vi "Beampointing_Multi_Pico2_upstairs01.vi"() -> ()   [LabVIEW 2011]
uses:
  GUI_Template/GUI_master/tcp_new_data_event.ctl
  GUI_Template/GUI_master/tcp new data cluster.ctl
  Ctrs/beam detection.ctl
  GUI_Beampointing_single_TRA/Ctrs/move.ctl
  <vilib>/Utility/file.llb/Read From Spreadsheet File (string).vi
  <userlib>/_OpenG.lib/array/array.llb/Filter 1D Array with Scalar (String)__ogtk.vi
  <vilib>/Utility/file.llb/Write To Spreadsheet File (string).vi
  <vilib>/Analysis/NI_AALBase.lvlib
panel:
  out "Moving Y":string
  out "Moving X":string
  out "particles":T1(array[cluster])
  out "millisecond timer value":u32
  out "appended path":path
  out "millisecond timer 2":u32
  in  "GUIdevice 98":string
  in  "Position.Axis 111::98":dbl=77.0 caption="Motor Axis 1" min=-999999.0 max=999999.0 format="%#_6f"
  in  "Position.Axis 112::98":dbl=77.0 caption="Motor Axis 1" min=-999999.0 max=999999.0 format="%#_6f"
  in  "Position.Axis 113::98":dbl=77.0 caption="Motor Axis 1" min=-999999.0 max=999999.0 format="%#_6f"
  in  "Position.Axis 121::98":dbl=77.0 caption="Motor Axis 1" min=-999999.0 max=999999.0 format="%#_6f"
  in  "Position.Axis 122::98":dbl=77.0 caption="Motor Axis 1" min=-999999.0 max=999999.0 format="%#_6f"
  in  "Position.Axis 123::98":dbl=77.0 caption="Motor Axis 1" min=-999999.0 max=999999.0 format="%#_6f"
  in  "Position.Axis 131::98":dbl=77.0 caption="Motor Axis 1" min=-999999.0 max=999999.0 format="%#_6f"
  in  "Position.Axis 132::98":dbl=77.0 caption="Motor Axis 1" min=-999999.0 max=999999.0 format="%#_6f"
  in  "Position.Axis 133::98":dbl=77.0 caption="Motor Axis 1" min=-999999.0 max=999999.0 format="%#_6f"
  in  "Position.Axis 141::98":dbl=77.0 caption="Motor Axis 1" min=-999999.0 max=999999.0 format="%#_6f"
  in  "Position.Axis 142::98":dbl=77.0 caption="Motor Axis 1" min=-999999.0 max=999999.0 format="%#_6f"
  in  "Position.Axis 143::98":dbl=77.0 caption="Motor Axis 1" min=-999999.0 max=999999.0 format="%#_6f"
  in  "Position.Axis 211::98":dbl=77.0 caption="Motor Axis 1" min=-999999.0 max=999999.0 format="%#_6f"
  in  "Position.Axis 212::98":dbl=77.0 caption="Motor Axis 1" min=-999999.0 max=999999.0 format="%#_6f"
  in  "Position.Axis 213::98":dbl=77.0 caption="Motor Axis 1" min=-999999.0 max=999999.0 format="%#_6f"
  in  "Position.Axis 221::98":dbl=77.0 caption="Motor Axis 1" min=-999999.0 max=999999.0 format="%#_6f"
  in  "Position.Axis 222::98":dbl=77.0 caption="Motor Axis 1" min=-999999.0 max=999999.0 format="%#_6f"
  in  "Position.Axis 223::98":dbl=77.0 caption="Motor Axis 1" min=-999999.0 max=999999.0 format="%#_6f"
  in  "Position.Axis 231::98":dbl=77.0 caption="Motor Axis 1" min=-999999.0 max=999999.0 format="%#_6f"
  in  "Position.Axis 232::98":dbl=77.0 caption="Motor Axis 1" min=-999999.0 max=999999.0 format="%#_6f"
  in  "Position.Axis 233::98":dbl=77.0 caption="Motor Axis 1" min=-999999.0 max=999999.0 format="%#_6f"
  in  "Position.Axis 241::98":dbl=77.0 caption="Motor Axis 1" min=-999999.0 max=999999.0 format="%#_6f"
  in  "Position.Axis 242::98":dbl=77.0 caption="Motor Axis 1" min=-999999.0 max=999999.0 format="%#_6f"
  in  "Position.Axis 243::98":dbl=77.0 caption="Motor Axis 1" min=-999999.0 max=999999.0 format="%#_6f"
  in  "Position.Axis 311::98":dbl=77.0 caption="Motor Axis 1" min=-999999.0 max=999999.0 format="%#_6f"
  in  "Position.Axis 312::98":dbl=77.0 caption="Motor Axis 1" min=-999999.0 max=999999.0 format="%#_6f"
  in  "Position.Axis 313::98":dbl=77.0 caption="Motor Axis 1" min=-999999.0 max=999999.0 format="%#_6f"
  in  "Position.Axis 321::98":dbl=77.0 caption="Motor Axis 1" min=-999999.0 max=999999.0 format="%#_6f"
  in  "Position.Axis 322::98":dbl=77.0 caption="Motor Axis 1" min=-999999.0 max=999999.0 format="%#_6f"
  in  "Position.Axis 323::98":dbl=77.0 caption="Motor Axis 1" min=-999999.0 max=999999.0 format="%#_6f"
  in  "Position.Axis 331::98":dbl=77.0 caption="Motor Axis 1" min=-999999.0 max=999999.0 format="%#_6f"
  in  "Position.Axis 332::98":dbl=77.0 caption="Motor Axis 1" min=-999999.0 max=999999.0 format="%#_6f"
  in  "Position.Axis 333::98":dbl=77.0 caption="Motor Axis 1" min=-999999.0 max=999999.0 format="%#_6f"
  in  "Position.Axis 341::98":dbl=77.0 caption="Motor Axis 1" min=-999999.0 max=999999.0 format="%#_6f"
  in  "Position.Axis 342::98":dbl=77.0 caption="Motor Axis 1" min=-999999.0 max=999999.0 format="%#_6f"
  in  "Position.Axis 343::98":dbl=77.0 caption="Motor Axis 1" min=-999999.0 max=999999.0 format="%#_6f"
  in  "Position.Axis 411::98":dbl=77.0 caption="Motor Axis 1" min=-999999.0 max=999999.0 format="%#_6f"
  in  "Position.Axis 412::98":dbl=77.0 caption="Motor Axis 1" min=-999999.0 max=999999.0 format="%#_6f"
  in  "Position.Axis 413::98":dbl=77.0 caption="Motor Axis 1" min=-999999.0 max=999999.0 format="%#_6f"
  in  "Position.Axis 421::98":dbl=77.0 caption="Motor Axis 1" min=-999999.0 max=999999.0 format="%#_6f"
  in  "Position.Axis 422::98":dbl=77.0 caption="Motor Axis 1" min=-999999.0 max=999999.0 format="%#_6f"
  in  "Position.Axis 423::98":dbl=77.0 caption="Motor Axis 1" min=-999999.0 max=999999.0 format="%#_6f"
  in  "Position.Axis 431::98":dbl=77.0 caption="Motor Axis 1" min=-999999.0 max=999999.0 format="%#_6f"
  in  "Position.Axis 432::98":dbl=77.0 caption="Motor Axis 1" min=-999999.0 max=999999.0 format="%#_6f"
  in  "Position.Axis 433::98":dbl=77.0 caption="Motor Axis 1" min=-999999.0 max=999999.0 format="%#_6f"
  in  "Position.Axis 441::98":dbl=77.0 caption="Motor Axis 1" min=-999999.0 max=999999.0 format="%#_6f"
  in  "Position.Axis 442::98":dbl=77.0 caption="Motor Axis 1" min=-999999.0 max=999999.0 format="%#_6f"
  in  "Position.Axis 443::98":dbl=77.0 caption="Motor Axis 1" min=-999999.0 max=999999.0 format="%#_6f"
  in  "Position.Axis 511::98":dbl=77.0 caption="Motor Axis 1" min=-999999.0 max=999999.0 format="%#_6f"
  in  "Position.Axis 512::98":dbl=77.0 caption="Motor Axis 1" min=-999999.0 max=999999.0 format="%#_6f"
  in  "Position.Axis 513::98":dbl=77.0 caption="Motor Axis 1" min=-999999.0 max=999999.0 format="%#_6f"
  in  "Position.Axis 521::98":dbl=77.0 caption="Motor Axis 1" min=-999999.0 max=999999.0 format="%#_6f"
  in  "Position.Axis 522::98":dbl=77.0 caption="Motor Axis 1" min=-999999.0 max=999999.0 format="%#_6f"
  in  "Position.Axis 523::98":dbl=77.0 caption="Motor Axis 1" min=-999999.0 max=999999.0 format="%#_6f"
  in  "Position.Axis 531::98":dbl=77.0 caption="Motor Axis 1" min=-999999.0 max=999999.0 format="%#_6f"
  in  "Position.Axis 532::98":dbl=77.0 caption="Motor Axis 1" min=-999999.0 max=999999.0 format="%#_6f"
  in  "Position.Axis 533::98":dbl=77.0 caption="Motor Axis 1" min=-999999.0 max=999999.0 format="%#_6f"
  in  "Position.Axis 541::98":dbl=77.0 caption="Motor Axis 1" min=-999999.0 max=999999.0 format="%#_6f"
  in  "Position.Axis 542::98":dbl=77.0 caption="Motor Axis 1" min=-999999.0 max=999999.0 format="%#_6f"
  in  "Position.Axis 543::98":dbl=77.0 caption="Motor Axis 1" min=-999999.0 max=999999.0 format="%#_6f"
  in  "Numeric":dbl
  out "Current State":string
  in  "output cluster 2":T5 {"detection para"."smal para"."Measurement Parameter" items=["Center of Mass X", "Center of Mass Y", "First Pixel X", "First Pixel Y", "Bounding Rect Left", "Bounding Rect Top", "Bounding Rect Right", "Bounding Rect Bottom", "Max Feret Diameter Start X", "Max Feret Diameter Start Y", "Max Feret Diameter End X", "Max Feret Diameter End Y", "Max Horiz. Segment Length Left", "Max Horiz. Segment Length Right", "Max Horiz. Segment Length Row", "-", "Bounding Rect Width", "Bounding Rect Height", "Bounding Rect Diagonal", "Perimeter", "Convex Hull Perimeter", "Holes' Perimeter", "Max Feret Diameter", "Equivalent Ellipse Major Axis", "Equivalent Ellipse Minor Axis", "Equivalent Ellipse Minor Axis (Feret)", "Equivalent Rect Long Side", "Equivalent Rect Short Side", "Equivalent Rect Diagonal", "Equivalent Rect Short Side (Feret)", "Average Horiz. Segment Length", "Average Vert. Segment Length", "Hydraulic Radius", "Waddel Disk Diameter", "-", "Area", "Holes' Area", "Particle & Holes' Area", "Convex Hull Area", "Image Area", "-", "Number of Holes", "Number of Horiz. Segments", "Number of Vert. Segments", "-", "Orientation", "Max Feret Diameter Orientation", "-", "% Area/Image Area", "% Area/(Particle & Holes' Area)", "Ratio of Equivalent Ellipse Axes", "Ratio of Equivalent Rect Sides", "-", "Elongation Factor", "Compactness Factor", "Heywood Circularity Factor", "Type Factor", "-", "Sum X", "Sum Y", "Sum XX", "Sum XY", "Sum YY", "Sum XXX", "Sum XXY", "Sum XYY", "Sum YYY", "-", "Moment of Inertia XX", "Moment of Inertia XY", "Moment of Inertia YY", "Moment of Inertia XXX", "Moment of Inertia XXY", "Moment of Inertia XYY", "Moment of Inertia YYY", "Norm. Moment of Inertia XX", "Norm. Moment of Inertia XY", "Norm. Moment of Inertia YY", "Norm. Moment of Inertia XXX", "Norm. Moment of Inertia XXY", "Norm. Moment of Inertia XYY", "Norm. Moment of Inertia YYY", "Hu Moment 1", "Hu Moment 2", "Hu Moment 3", "Hu Moment 4", "Hu Moment 5", "Hu Moment 6", "Hu Moment 7"]; "detection para"."smal para"."Range Lower Value" format="%.2f"; "detection para"."smal para"."Range Upper Value" format="%.2f"; "detection para"."detection method" items=["clustering", "entropy", "metric", "moments", "inter-class variance"]; "detection para"."Filter" items=["No Filter", "Median Filter", "Low Pass Filter"]}
  out "CCDs":string[](array[string])
  in  "GUIdevice 12":string
  in  "GUIdevice 11":string
  in  "GUIdevice 10":string
  in  "GUIdevice 9":string
  out "error out 2":errorcluster
  in  "active cams":string[](array[string])
  in  "Motor Y":dbl[][](array[numeric])
  in  "Motor X":dbl[][](array[numeric])
  out "Names":string[](array[string])
  in  "Offset X stats":dbl[][](array[numeric])
  in  "Offset Y stats":dbl[][](array[numeric])
  out "Box":T6(array[cluster])
  in  "Tab Control 2":enum32{"Config ", "Main", "History"}(tab)=enum."Main"
  out "Waveform Chart":u32(graph)
  in  "associated motors":T7 {"Motor CCD 12" items=["PA2_Input1", "PA2_Input2", "XPW_cam", "L1_TelInpNear", "A", "B", "a", "D", "", "TSa", "", "", "Focuscam", "Mirrorcam", "", "", "", "", "", ""]; "Motor CCD 11" items=["PA2_Input1", "PA2_Input2", "XPW_cam", "L1_TelInpNear", "A", "B", "a", "D", "", "TSa", "", "", "Focuscam", "Mirrorcam", "", "", "", "", "", ""]; "Motor CCD 10" items=["PA2_Input1", "PA2_Input2", "XPW_cam", "L1_TelInpNear", "A", "B", "a", "D", "", "TSa", "", "", "Focuscam", "Mirrorcam", "", "", "", "", "", ""]; "Motor CCD 9" items=["PA2_Input1", "PA2_Input2", "XPW_cam", "L1_TelInpNear", "A", "B", "a", "D", "", "TSa", "", "", "Focuscam", "Mirrorcam", "", "", "", "", "", ""]; "Motor CCD 8" items=["PA2_Input1", "PA2_Input2", "XPW_cam", "L1_TelInpNear", "A", "B", "a", "D", "", "TSa", "", "", "Focuscam", "Mirrorcam", "", "", "", "", "", ""]; "Motor CCD 7" items=["PA2_Input1", "PA2_Input2", "XPW_cam", "L1_TelInpNear", "A", "B", "a", "D", "", "TSa", "", "", "Focuscam", "Mirrorcam", "", "", "", "", "", ""]; "Motor CCD 6" items=["PA2_Input1", "PA2_Input2", "XPW_cam", "L1_TelInpNear", "A", "B", "a", "D", "", "TSa", "", "", "Focuscam", "Mirrorcam", "", "", "", "", "", ""]; "Motor CCD 5" items=["PA2_Input1", "PA2_Input2", "XPW_cam", "L1_TelInpNear", "A", "B", "a", "D", "", "TSa", "", "", "Focuscam", "Mirrorcam", "", "", "", "", "", ""]; "Motor CCD 4" items=["PA2_Input1", "PA2_Input2", "XPW_cam", "L1_TelInpNear", "A", "B", "a", "D", "", "TSa", "", "", "Focuscam", "Mirrorcam", "", "", "", "", "", ""]; "Motor CCD 3" items=["PA2_Input1", "PA2_Input2", "XPW_cam", "L1_TelInpNear", "A", "B", "a", "D", "", "TSa", "", "", "Focuscam", "Mirrorcam", "", "", "", "", "", ""]; "Motor CCD 2" items=["PA2_Input1", "PA2_Input2", "XPW_cam", "L1_TelInpNear", "A", "B", "a", "D", "", "TSa", "", "", "Focuscam", "Mirrorcam", "", "", "", "", "", ""]; "Motor CCD 1" items=["PA2_Input1", "PA2_Input2", "XPW_cam", "L1_TelInpNear", "A", "B", "a", "D", "", "TSa", "", "", "Focuscam", "Mirrorcam", "", "", "", "", "", ""]}
  out "Cameras":T8
  out "Status":cluster{i32, i32, "Centroid X":dbl[][]}(graph)
  in  "Exposure:12":dbl=0.095 min=0.0001 max=1.0 format="%#_6f"
  in  "Triggerdelay::12":dbl=0.003 min=0.0 max=0.09 format="%#_6f"
  in  "Exposure::11":dbl=0.095 min=0.0001 max=1.0 format="%#_6f"
  in  "Triggerdelay::11":dbl=0.003 min=0.0 max=0.09 format="%#_6f"
  in  "Exposure::10":dbl=0.095 min=0.0001 max=1.0 format="%#_6f"
  in  "Triggerdelay::10":dbl=0.003 min=0.0 max=0.09 format="%#_6f"
  in  "Exposure::9":dbl=0.095 min=0.0001 max=1.0 format="%#_6f"
  in  "Triggerdelay::9":dbl=0.003 min=0.0 max=0.09 format="%#_6f"
  in  "Trigger::9":bool
  in  "Trigger::10":bool caption="Trigger:10"
  in  "Trigger::11":bool
  in  "Trigger::12":bool
  in  "Target.Y::9":dbl=45.0 caption="T9y" min=0.0 max=2000.0 format="%#_6f"
  in  "Target.X::9":dbl=47.0 caption="Tx9" min=0.0 max=2000.0 format="%#_6f"
  in  "Target.Y::10":dbl=45.0 caption="T10y" min=0.0 max=2000.0 format="%#_6f"
  in  "Target.X::10":dbl=47.0 caption="T10x" min=0.0 max=2000.0 format="%#_6f"
  in  "Target.Y::11":dbl=45.0 caption="T11y" min=0.0 max=2000.0 format="%#_6f"
  in  "Target.X::11":dbl=47.0 caption="T11x" min=0.0 max=2000.0 format="%#_6f"
  in  "Target.Y::12":dbl=45.0 caption="T12y" min=0.0 max=2000.0 format="%#_6f"
  in  "Target.X::12":dbl=47.0 caption="T12x" min=0.0 max=2000.0 format="%#_6f"
  in  "Exposure::8":dbl=0.095 min=0.01 max=1.0 format="%#_6f"
  in  "Triggerdelay::8":dbl=0.003 min=0.0 max=0.09 format="%#_6f"
  in  "Trigger::8":bool
  in  "Target.Y::8":dbl=45.0 caption="T8y" min=0.0 max=2000.0 format="%#_6f"
  in  "Target.X::8":dbl=47.0 caption="T8x" min=0.0 max=2000.0 format="%#_6f"
  in  "Target.Y::7":dbl=45.0 caption="T7x" min=0.0 max=2000.0 format="%#_6f"
  in  "Target.X::7":dbl=47.0 caption="T7y" min=0.0 max=2000.0 format="%#_6f"
  in  "Target.Y::6":dbl=45.0 caption="T6y" min=0.0 max=2000.0 format="%#_6f"
  in  "Target.X::6":dbl=47.0 caption="T6x" min=0.0 max=2000.0 format="%#_6f"
  in  "Target.Y::5":dbl=45.0 caption="T5y" min=0.0 max=2000.0 format="%#_6f"
  in  "Target.X::5":dbl=47.0 caption="T5x" min=0.0 max=2000.0 format="%#_6f"
  in  "Target.Y::4":dbl=45.0 caption="T4y" min=0.0 max=2000.0 format="%#_6f"
  in  "Target.X::4":dbl=47.0 caption="T4x" min=0.0 max=2000.0 format="%#_6f"
  in  "Target.Y::3":dbl=163.0 caption="T3y" min=0.0 max=2000.0 format="%#_6f"
  in  "Target.X::3":dbl=152.0 caption="T3x" min=0.0 max=2000.0 format="%#_6f"
  in  "Target.Y::2":dbl=74.0 caption="T2y" min=0.0 max=2000.0 format="%#_6f"
  in  "Target.X::2":dbl=75.0 caption="T2x" min=0.0 max=2000.0 format="%#_6f"
  in  "Target.Y::1":dbl=61.0 caption="T1y" min=0.0 max=2000.0 format="%#_6f"
  in  "Target.X::1":dbl=77.0 caption="T1x" min=0.0 max=2000.0 format="%#_6f"
  in  "Exposure::7":dbl=0.095 min=0.0001 max=1.0 format="%#_6f"
  in  "Triggerdelay::7":dbl=0.003 min=0.0 max=0.09 format="%#_6f"
  in  "Trigger::7":bool
  in  "Exposure::6":dbl=0.095 min=0.0001 max=1.0 format="%#_6f"
  in  "Triggerdelay::6":dbl=0.003 min=0.0 max=0.09 format="%#_6f"
  in  "Trigger::6":bool
  in  "Exposure::5":dbl=0.095 min=0.0001 max=1.0 format="%#_6f"
  in  "Triggerdelay::5":dbl=0.003 min=0.0 max=0.09 format="%#_6f"
  in  "Trigger::5":bool
  in  "Exposure::4":dbl=0.095 min=0.0001 max=1.0 format="%#_6f"
  in  "Triggerdelay::4":dbl=0.003 min=0.0 max=0.09 format="%#_6f"
  in  "Trigger::4":bool
  in  "Exposure::3":dbl=0.095 min=0.0001 max=1.0 format="%#_6f"
  in  "Triggerdelay::3":dbl=0.003 min=0.0 max=0.09 format="%#_6f"
  in  "Trigger::3":bool
  in  "Exposure::2":dbl=0.095 min=0.0001 max=1.0 format="%#_6f"
  in  "Triggerdelay::2":dbl=0.003 min=0.0 max=0.09 format="%#_6f"
  in  "Trigger::2":bool
  out "image::1":T9(plugin-control) caption="LM_Mirrorcam"
  out "image::2":T9(plugin-control) caption="LM_Focuscam"
  out "image::3":T9(plugin-control) caption="TS-253a_in"
  out "image::4":T9(plugin-control)
  out "image::5":T9(plugin-control)
  out "image::6":T9(plugin-control)
  out "image::7":T9(plugin-control)
  out "image::8":T9(plugin-control)
  in  "Exposure::1":dbl=0.095 min=0.0001 max=1.0 format="%#_6f"
  in  "Triggerdelay::1":dbl=0.003 min=0.0 max=0.09 format="%#_6f"
  in  "Trigger::1":bool
  in  "UDP error message":string
  out "required Y":bool[](array[boolean])
  out "required X":bool[](array[boolean])
  out "detected":bool[](array[boolean])
  out "name array":string[](array[string])
  out "image::9":T9(plugin-control)
  out "image::10":T9(plugin-control)
  out "image::11":T9(plugin-control)
  out "image::12":T9(plugin-control)
  out "speedmode X":bool[](array[boolean])
  out "speedmode Y":bool[](array[boolean])
  out "CCD 9":cluster{timestamp[], dbl[]}[](graph)
  out "CCD 10":cluster{timestamp[], dbl[]}[](graph)
  out "CCD 11":cluster{timestamp[], dbl[]}[](graph)
  out "CCD 12":cluster{timestamp[], dbl[]}[](graph)
  out "CCD 5":cluster{timestamp[], dbl[]}[](graph)
  out "CCD 6":cluster{timestamp[], dbl[]}[](graph)
  out "CCD 7":cluster{timestamp[], dbl[]}[](graph)
  out "CCD 8":cluster{timestamp[], dbl[]}[](graph)
  out "CCD 2":cluster{timestamp[], dbl[]}[](graph)
  out "CCD 1":cluster{timestamp[], dbl[]}[](graph)
  out "CCD 3":cluster{timestamp[], dbl[]}[](graph)
  out "CCD 4":cluster{timestamp[], dbl[]}[](graph)
  out "History index":i32
  in  "History Size":i32=500
  out "Particle Reports (Pixels)":T10(array[cluster])
  in  "Feedback Global":bool
  in  "detection para":T3[](array[typedef])=[{"Filter"=1, "Filter Para"={"X Size"=5, "Y Size"=5, "% Tolerance"=1}, "detection method"=4, "smal para"=[{"Measurement Parameter"=35, "Range Lower Value"=0.0, "Range Upper Value"=0.0, "Range"=TRUE, "Measurement Type"=FALSE}], "Remove small Objects"=TRUE, "Restrict to round Objects"=FALSE}, {"Filter"=1, "Filter Para"={"X Size"=5, "Y Size"=5, "% Tolerance"=1}, "detection method"=4, "smal para"=[{"Measurement Parameter"=35, "Range Lower Value"=0.0, "Range Upper Value"=500.0, "Range"=FALSE, "Measurement Type"=FALSE}], "Remove small Objects"=TRUE, "Restrict to round Objects"=FALSE}, {"Filter"=1, "Filter Para"={"X Size"=5, "Y Size"=5, "% Tolerance"=1}, "detection method"=4, "smal para"=[{"Measurement Parameter"=35, "Range Lower Value"=0.0, "Range Upper Value"=500.0, "Range"=TRUE, "Measurement Type"=FALSE}], "Remove small Objects"=TRUE, "Restrict to round Objects"=FALSE}, {"Filter"=1, "Filter Para"={"X Size"=5, "Y Size"=5, "% Tolerance"=1}, "detection method"=4, "smal para"=[{"Measurement Parameter"=35, "Range Lower Value"=0.0, "Range Upper Value"=500.0, "Range"=TRUE, "Measurement Type"=FALSE}], "Remove small Objects"=TRUE, "Restrict to round Objects"=FALSE}, {"Filter"=1, "Filter Para"={"X Size"=5, "Y Size"=5, "% Tolerance"=1}, "detection method"=4, "smal para"=[{"Measurement Parameter"=35, "Range Lower Value"=0.0, "Range Upper Value"=500.0, "Range"=TRUE, "Measurement Type"=FALSE}], "Remove small Objects"=TRUE, "Restrict to round Objects"=FALSE}, {"Filter"=1, "Filter Para"={"X Size"=5, "Y Size"=5, "% Tolerance"=1}, "detection method"=4, "smal para"=[{"Measurement Parameter"=35, "Range Lower Value"=0.0, "Range Upper Value"=500.0, "Range"=TRUE, "Measurement Type"=FALSE}], "Remove small Objects"=TRUE, "Restrict to round Objects"=FALSE}, {"Filter"=1, "Filter Para"={"X Size"=5, "Y Size"=5, "% Tolerance"=1}, "detection method"=4, "smal para"=[{"Measurement Parameter"=35, "Range Lower Value"=0.0, "Range Upper Value"=500.0, "Range"=TRUE, "Measurement Type"=FALSE}], "Remove small Objects"=TRUE, "Restrict to round Objects"=FALSE}, {"Filter"=1, "Filter Para"={"X Size"=5, "Y Size"=5, "% Tolerance"=1}, "detection method"=3, "smal para"=[{"Measurement Parameter"=35, "Range Lower Value"=0.0, "Range Upper Value"=0.0, "Range"=FALSE, "Measurement Type"=FALSE}], "Remove small Objects"=TRUE, "Restrict to round Objects"=FALSE}, {"Filter"=1, "Filter Para"={"X Size"=5, "Y Size"=5, "% Tolerance"=1}, "detection method"=4, "smal para"=[{"Measurement Parameter"=35, "Range Lower Value"=0.0, "Range Upper Value"=0.0, "Range"=FALSE, "Measurement Type"=FALSE}], "Remove small Objects"=TRUE, "Restrict to round Objects"=FALSE}, {"Filter"=1, "Filter Para"={"X Size"=5, "Y Size"=5, "% Tolerance"=1}, "detection method"=4, "smal para"=[{"Measurement Parameter"=35, "Range Lower Value"=0.0, "Range Upper Value"=500.0, "Range"=TRUE, "Measurement Type"=FALSE}], "Remove small Objects"=TRUE, "Restrict to round Objects"=FALSE}, {"Filter"=1, "Filter Para"={"X Size"=5, "Y Size"=5, "% Tolerance"=1}, "detection method"=4, "smal para"=[{"Measurement Parameter"=35, "Range Lower Value"=0.0, "Range Upper Value"=500.0, "Range"=TRUE, "Measurement Type"=FALSE}], "Remove small Objects"=TRUE, "Restrict to round Objects"=FALSE}, {"Filter"=1, "Filter Para"={"X Size"=5, "Y Size"=5, "% Tolerance"=1}, "detection method"=4, "smal para"=[{"Measurement Parameter"=35, "Range Lower Value"=0.0, "Range Upper Value"=500.0, "Range"=TRUE, "Measurement Type"=FALSE}], "Remove small Objects"=TRUE, "Restrict to round Objects"=FALSE}] {"smal para"."Measurement Parameter" items=["Center of Mass X", "Center of Mass Y", "First Pixel X", "First Pixel Y", "Bounding Rect Left", "Bounding Rect Top", "Bounding Rect Right", "Bounding Rect Bottom", "Max Feret Diameter Start X", "Max Feret Diameter Start Y", "Max Feret Diameter End X", "Max Feret Diameter End Y", "Max Horiz. Segment Length Left", "Max Horiz. Segment Length Right", "Max Horiz. Segment Length Row", "-", "Bounding Rect Width", "Bounding Rect Height", "Bounding Rect Diagonal", "Perimeter", "Convex Hull Perimeter", "Holes' Perimeter", "Max Feret Diameter", "Equivalent Ellipse Major Axis", "Equivalent Ellipse Minor Axis", "Equivalent Ellipse Minor Axis (Feret)", "Equivalent Rect Long Side", "Equivalent Rect Short Side", "Equivalent Rect Diagonal", "Equivalent Rect Short Side (Feret)", "Average Horiz. Segment Length", "Average Vert. Segment Length", "Hydraulic Radius", "Waddel Disk Diameter", "-", "Area", "Holes' Area", "Particle & Holes' Area", "Convex Hull Area", "Image Area", "-", "Number of Holes", "Number of Horiz. Segments", "Number of Vert. Segments", "-", "Orientation", "Max Feret Diameter Orientation", "-", "% Area/Image Area", "% Area/(Particle & Holes' Area)", "Ratio of Equivalent Ellipse Axes", "Ratio of Equivalent Rect Sides", "-", "Elongation Factor", "Compactness Factor", "Heywood Circularity Factor", "Type Factor", "-", "Sum X", "Sum Y", "Sum XX", "Sum XY", "Sum YY", "Sum XXX", "Sum XXY", "Sum XYY", "Sum YYY", "-", "Moment of Inertia XX", "Moment of Inertia XY", "Moment of Inertia YY", "Moment of Inertia XXX", "Moment of Inertia XXY", "Moment of Inertia XYY", "Moment of Inertia YYY", "Norm. Moment of Inertia XX", "Norm. Moment of Inertia XY", "Norm. Moment of Inertia YY", "Norm. Moment of Inertia XXX", "Norm. Moment of Inertia XXY", "Norm. Moment of Inertia XYY", "Norm. Moment of Inertia YYY", "Hu Moment 1", "Hu Moment 2", "Hu Moment 3", "Hu Moment 4", "Hu Moment 5", "Hu Moment 6", "Hu Moment 7"]; "smal para"."Range Lower Value" format="%.2f"; "smal para"."Range Upper Value" format="%.2f"; "detection method" items=["clustering", "entropy", "metric", "moments", "inter-class variance"]; "Filter" items=["No Filter", "Median Filter", "Low Pass Filter"]}
  in  "GUIdevice 8":string="B5_CompressorOut"
  in  "Tab Control":T11(tab)
  in  "Center":bool
  in  "Save Stats":bool
  in  "Save Config":bool
  in  "Load Config":bool
  in  "update speed [ms]":i32=200
  in  "Img to avg":i32=20
  in  "Reset History":bool
  in  "save path":path=path "W:/BP_DATA"
  in  "autodetect":bool
  in  "Detection Rate":dbl=0.8 min=0.001 max=1.0
  in  "new tdms":bool
  in  "Speedmode @":dbl=3.0 min=1.0 max=20.0
  in  "Align":bool
  in  "deivice ini":bool
  in  "beam detection para":T3={"Filter"=1, "Filter Para"={"X Size"=5, "Y Size"=5, "% Tolerance"=1}, "detection method"=4, "smal para"=[{"Measurement Parameter"=35, "Range Lower Value"=0.0, "Range Upper Value"=500.0, "Range"=FALSE, "Measurement Type"=FALSE}], "Remove small Objects"=TRUE, "Restrict to round Objects"=FALSE} {"smal para"."Measurement Parameter" items=["Center of Mass X", "Center of Mass Y", "First Pixel X", "First Pixel Y", "Bounding Rect Left", "Bounding Rect Top", "Bounding Rect Right", "Bounding Rect Bottom", "Max Feret Diameter Start X", "Max Feret Diameter Start Y", "Max Feret Diameter End X", "Max Feret Diameter End Y", "Max Horiz. Segment Length Left", "Max Horiz. Segment Length Right", "Max Horiz. Segment Length Row", "-", "Bounding Rect Width", "Bounding Rect Height", "Bounding Rect Diagonal", "Perimeter", "Convex Hull Perimeter", "Holes' Perimeter", "Max Feret Diameter", "Equivalent Ellipse Major Axis", "Equivalent Ellipse Minor Axis", "Equivalent Ellipse Minor Axis (Feret)", "Equivalent Rect Long Side", "Equivalent Rect Short Side", "Equivalent Rect Diagonal", "Equivalent Rect Short Side (Feret)", "Average Horiz. Segment Length", "Average Vert. Segment Length", "Hydraulic Radius", "Waddel Disk Diameter", "-", "Area", "Holes' Area", "Particle & Holes' Area", "Convex Hull Area", "Image Area", "-", "Number of Holes", "Number of Horiz. Segments", "Number of Vert. Segments", "-", "Orientation", "Max Feret Diameter Orientation", "-", "% Area/Image Area", "% Area/(Particle & Holes' Area)", "Ratio of Equivalent Ellipse Axes", "Ratio of Equivalent Rect Sides", "-", "Elongation Factor", "Compactness Factor", "Heywood Circularity Factor", "Type Factor", "-", "Sum X", "Sum Y", "Sum XX", "Sum XY", "Sum YY", "Sum XXX", "Sum XXY", "Sum XYY", "Sum YYY", "-", "Moment of Inertia XX", "Moment of Inertia XY", "Moment of Inertia YY", "Moment of Inertia XXX", "Moment of Inertia XXY", "Moment of Inertia XYY", "Moment of Inertia YYY", "Norm. Moment of Inertia XX", "Norm. Moment of Inertia XY", "Norm. Moment of Inertia YY", "Norm. Moment of Inertia XXX", "Norm. Moment of Inertia XXY", "Norm. Moment of Inertia XYY", "Norm. Moment of Inertia YYY", "Hu Moment 1", "Hu Moment 2", "Hu Moment 3", "Hu Moment 4", "Hu Moment 5", "Hu Moment 6", "Hu Moment 7"]; "smal para"."Range Lower Value" format="%.2f"; "smal para"."Range Upper Value" format="%.2f"; "detection method" items=["clustering", "entropy", "metric", "moments", "inter-class variance"]; "Filter" items=["No Filter", "Median Filter", "Low Pass Filter"]}
  in  "move config":T2={"Tolerance [%]"=0.1, "Stepsize"=0.0001, "Invert Axis"=TRUE, "Invert Direction X"=FALSE, "Invert Direction Y"=TRUE, "enable feedback"=FALSE, "Set Centriod Target"=FALSE}
  in  "ActiveMotor":u16(ring)=7 items=["PA2_Input1", "PA2_Input2", "XPW_cam", "L1_TelInpNear", "A", "B", "a", "D", "", "TSa", "", "", "Focuscam", "Mirrorcam", "", "", "", "", "", ""]
  in  "ActiveMotorName::99":string
  in  "RelativeMove.Axis 1.CCW::99":bool caption="RelativeMove.Axis 1.CCW::1"
  in  "RelativeMove.Axis 1.CW::99":bool caption="RelativeMove.Axis 1.CW::1"
  in  "RelativeMove.Axis 2.CCW::99":bool caption="RelativeMove.Axis. 2.CCW::1"
  in  "RelativeMove.Axis 2.CW::99":bool caption="RelativeMove.Axis 2.CW::1"
  in  "RelativeSettings.Axis 1.Position::99":dbl caption="Axis 1 Position" min=-999999.0 max=999999.0 format="%_4p"
  in  "RelativeSettings.Axis 2.Position::99":dbl caption="Axis 2 Position" min=-999999.0 max=999999.0 format="%_4p"
  in  "RelativeSettings.Axis 2.StepSize::99":dbl=50.0 caption="Axis 2 StepSize" min=0.0 max=999999.0 format="%_4p"
  in  "RelativeSettings.Axis 1.StepSize::99":dbl=50.0 caption="Axis 1 Stepsize" min=0.0 max=999999.0 format="%_4p"
  out "Arguments Y":string
  in  "active axis refs 2":T12(array[cluster])
  in  "active Axis ref":cluster{"Ref X":refnum<vi>, "Ref Y":refnum<vi>}
  in  "CCDs":u16(ring) items=["LM_Mirrorcam", "LM_Focuscam", "TS-253a_in", "", "", "", "", "", "", "", "", ""]
  out "motor refs":refnum<vi>[](array[refnum])
  in  "Position.Axis 511::99":dbl=77.0 caption="Motor Axis 1" min=-999999.0 max=999999.0 format="%#_6f"
  in  "Position.Axis 512::99":dbl=77.0 caption="Motor Axis 1" min=-999999.0 max=999999.0 format="%#_6f"
  in  "Position.Axis 513::99":dbl=77.0 caption="Motor Axis 1" min=-999999.0 max=999999.0 format="%#_6f"
  in  "Position.Axis 521::99":dbl=77.0 caption="Motor Axis 1" min=-999999.0 max=999999.0 format="%#_6f"
  in  "Position.Axis 522::99":dbl=77.0 caption="Motor Axis 1" min=-999999.0 max=999999.0 format="%#_6f"
  in  "Position.Axis 523::99":dbl=77.0 caption="Motor Axis 1" min=-999999.0 max=999999.0 format="%#_6f"
  in  "Position.Axis 531::99":dbl=77.0 caption="Motor Axis 1" min=-999999.0 max=999999.0 format="%#_6f"
  in  "Position.Axis 532::99":dbl=77.0 caption="Motor Axis 1" min=-999999.0 max=999999.0 format="%#_6f"
  in  "Position.Axis 533::99":dbl=77.0 caption="Motor Axis 1" min=-999999.0 max=999999.0 format="%#_6f"
  in  "Position.Axis 541::99":dbl=77.0 caption="Motor Axis 1" min=-999999.0 max=999999.0 format="%#_6f"
  in  "Position.Axis 542::99":dbl=77.0 caption="Motor Axis 1" min=-999999.0 max=999999.0 format="%#_6f"
  in  "Position.Axis 543::99":dbl=77.0 caption="Motor Axis 1" min=-999999.0 max=999999.0 format="%#_6f"
  in  "Position.Axis 411::99":dbl=77.0 caption="Motor Axis 1" min=-999999.0 max=999999.0 format="%#_6f"
  in  "Position.Axis 412::99":dbl=77.0 caption="Motor Axis 1" min=-999999.0 max=999999.0 format="%#_6f"
  in  "Position.Axis 413::99":dbl=77.0 caption="Motor Axis 1" min=-999999.0 max=999999.0 format="%#_6f"
  in  "Position.Axis 421::99":dbl=77.0 caption="Motor Axis 1" min=-999999.0 max=999999.0 format="%#_6f"
  in  "Position.Axis 422::99":dbl=77.0 caption="Motor Axis 1" min=-999999.0 max=999999.0 format="%#_6f"
  in  "Position.Axis 423::99":dbl=77.0 caption="Motor Axis 1" min=-999999.0 max=999999.0 format="%#_6f"
  in  "Position.Axis 431::99":dbl=77.0 caption="Motor Axis 1" min=-999999.0 max=999999.0 format="%#_6f"
  in  "Position.Axis 432::99":dbl=77.0 caption="Motor Axis 1" min=-999999.0 max=999999.0 format="%#_6f"
  in  "Position.Axis 433::99":dbl=77.0 caption="Motor Axis 1" min=-999999.0 max=999999.0 format="%#_6f"
  in  "Position.Axis 441::99":dbl=77.0 caption="Motor Axis 1" min=-999999.0 max=999999.0 format="%#_6f"
  in  "Position.Axis 442::99":dbl=77.0 caption="Motor Axis 1" min=-999999.0 max=999999.0 format="%#_6f"
  in  "Position.Axis 443::99":dbl=77.0 caption="Motor Axis 1" min=-999999.0 max=999999.0 format="%#_6f"
  in  "Position.Axis 311::99":dbl=77.0 caption="Motor Axis 1" min=-999999.0 max=999999.0 format="%#_6f"
  in  "Position.Axis 312::99":dbl=77.0 caption="Motor Axis 1" min=-999999.0 max=999999.0 format="%#_6f"
  in  "Position.Axis 313::99":dbl=77.0 caption="Motor Axis 1" min=-999999.0 max=999999.0 format="%#_6f"
  in  "Position.Axis 321::99":dbl=77.0 caption="Motor Axis 1" min=-999999.0 max=999999.0 format="%#_6f"
  in  "Position.Axis 322::99":dbl=77.0 caption="Motor Axis 1" min=-999999.0 max=999999.0 format="%#_6f"
  in  "Position.Axis 323::99":dbl=77.0 caption="Motor Axis 1" min=-999999.0 max=999999.0 format="%#_6f"
  in  "Position.Axis 331::99":dbl=77.0 caption="Motor Axis 1" min=-999999.0 max=999999.0 format="%#_6f"
  in  "Position.Axis 332::99":dbl=77.0 caption="Motor Axis 1" min=-999999.0 max=999999.0 format="%#_6f"
  in  "Position.Axis 333::99":dbl=77.0 caption="Motor Axis 1" min=-999999.0 max=999999.0 format="%#_6f"
  in  "Position.Axis 341::99":dbl=77.0 caption="Motor Axis 1" min=-999999.0 max=999999.0 format="%#_6f"
  in  "Position.Axis 342::99":dbl=77.0 caption="Motor Axis 1" min=-999999.0 max=999999.0 format="%#_6f"
  in  "Position.Axis 343::99":dbl=77.0 caption="Motor Axis 1" min=-999999.0 max=999999.0 format="%#_6f"
  in  "Position.Axis 241::99":dbl=77.0 caption="Motor Axis 1" min=-999999.0 max=999999.0 format="%#_6f"
  in  "Position.Axis 242::99":dbl=77.0 caption="Motor Axis 1" min=-999999.0 max=999999.0 format="%#_6f"
  in  "Position.Axis 243::99":dbl=77.0 caption="Motor Axis 1" min=-999999.0 max=999999.0 format="%#_6f"
  in  "Position.Axis 231::99":dbl=77.0 caption="Motor Axis 1" min=-999999.0 max=999999.0 format="%#_6f"
  in  "Position.Axis 232::99":dbl=77.0 caption="Motor Axis 1" min=-999999.0 max=999999.0 format="%#_6f"
  in  "Position.Axis 233::99":dbl=77.0 caption="Motor Axis 1" min=-999999.0 max=999999.0 format="%#_6f"
  in  "Position.Axis 221::99":dbl=77.0 caption="Motor Axis 1" min=-999999.0 max=999999.0 format="%#_6f"
  in  "Position.Axis 222::99":dbl=77.0 caption="Motor Axis 1" min=-999999.0 max=999999.0 format="%#_6f"
  in  "Position.Axis 223::99":dbl=77.0 caption="Motor Axis 1" min=-999999.0 max=999999.0 format="%#_6f"
  in  "Position.Axis 211::99":dbl=77.0 caption="Motor Axis 1" min=-999999.0 max=999999.0 format="%#_6f"
  in  "Position.Axis 212::99":dbl=77.0 caption="Motor Axis 1" min=-999999.0 max=999999.0 format="%#_6f"
  in  "Position.Axis 213::99":dbl=77.0 caption="Motor Axis 1" min=-999999.0 max=999999.0 format="%#_6f"
  in  "Position.Axis 141::99":dbl=77.0 caption="Motor Axis 1" min=-999999.0 max=999999.0 format="%#_6f"
  in  "Position.Axis 142::99":dbl=77.0 caption="Motor Axis 1" min=-999999.0 max=999999.0 format="%#_6f"
  in  "Position.Axis 143::99":dbl=77.0 caption="Motor Axis 1" min=-999999.0 max=999999.0 format="%#_6f"
  in  "Position.Axis 131::99":dbl=77.0 caption="Motor Axis 1" min=-999999.0 max=999999.0 format="%#_6f"
  in  "Position.Axis 132::99":dbl=77.0 caption="Motor Axis 1" min=-999999.0 max=999999.0 format="%#_6f"
  in  "Position.Axis 133::99":dbl=77.0 caption="Motor Axis 1" min=-999999.0 max=999999.0 format="%#_6f"
  in  "Position.Axis 121::99":dbl=77.0 caption="Motor Axis 1" min=-999999.0 max=999999.0 format="%#_6f"
  in  "Position.Axis 122::99":dbl=77.0 caption="Motor Axis 1" min=-999999.0 max=999999.0 format="%#_6f"
  in  "Position.Axis 123::99":dbl=77.0 caption="Motor Axis 1" min=-999999.0 max=999999.0 format="%#_6f"
  in  "Position.Axis 113::99":dbl=77.0 caption="Motor Axis 1" min=-999999.0 max=999999.0 format="%#_6f"
  in  "Position.Axis 112::99":dbl=77.0 caption="Motor Axis 1" min=-999999.0 max=999999.0 format="%#_6f"
  in  "Position.Axis 111::99":dbl=77.0 caption="Motor Axis 1" min=-999999.0 max=999999.0 format="%#_6f"
  out "Arguments X":string
  in  "GUIdevice 99":string="Picopad23"
  in  "move properties":T2[](array[typedef])=[{"Tolerance [%]"=0.1, "Stepsize"=0.0001, "Invert Axis"=TRUE, "Invert Direction X"=FALSE, "Invert Direction Y"=TRUE, "enable feedback"=FALSE, "Set Centriod Target"=FALSE}, {"Tolerance [%]"=0.1, "Stepsize"=0.0001, "Invert Axis"=TRUE, "Invert Direction X"=FALSE, "Invert Direction Y"=TRUE, "enable feedback"=FALSE, "Set Centriod Target"=FALSE}, {"Tolerance [%]"=0.1, "Stepsize"=0.0001, "Invert Axis"=TRUE, "Invert Direction X"=FALSE, "Invert Direction Y"=TRUE, "enable feedback"=FALSE, "Set Centriod Target"=FALSE}, {"Tolerance [%]"=0.1, "Stepsize"=0.0001, "Invert Axis"=TRUE, "Invert Direction X"=FALSE, "Invert Direction Y"=TRUE, "enable feedback"=FALSE, "Set Centriod Target"=FALSE}, {"Tolerance [%]"=0.1, "Stepsize"=0.0001, "Invert Axis"=TRUE, "Invert Direction X"=FALSE, "Invert Direction Y"=TRUE, "enable feedback"=FALSE, "Set Centriod Target"=FALSE}, {"Tolerance [%]"=0.1, "Stepsize"=0.0001, "Invert Axis"=TRUE, "Invert Direction X"=FALSE, "Invert Direction Y"=TRUE, "enable feedback"=FALSE, "Set Centriod Target"=FALSE}, {"Tolerance [%]"=0.1, "Stepsize"=0.0001, "Invert Axis"=TRUE, "Invert Direction X"=FALSE, "Invert Direction Y"=TRUE, "enable feedback"=FALSE, "Set Centriod Target"=FALSE}, {"Tolerance [%]"=0.1, "Stepsize"=0.0001, "Invert Axis"=TRUE, "Invert Direction X"=FALSE, "Invert Direction Y"=TRUE, "enable feedback"=FALSE, "Set Centriod Target"=FALSE}, {"Tolerance [%]"=0.1, "Stepsize"=0.0001, "Invert Axis"=TRUE, "Invert Direction X"=FALSE, "Invert Direction Y"=TRUE, "enable feedback"=FALSE, "Set Centriod Target"=FALSE}, {"Tolerance [%]"=0.1, "Stepsize"=0.0001, "Invert Axis"=TRUE, "Invert Direction X"=FALSE, "Invert Direction Y"=TRUE, "enable feedback"=FALSE, "Set Centriod Target"=FALSE}, {"Tolerance [%]"=0.1, "Stepsize"=0.0001, "Invert Axis"=TRUE, "Invert Direction X"=FALSE, "Invert Direction Y"=TRUE, "enable feedback"=FALSE, "Set Centriod Target"=FALSE}, {"Tolerance [%]"=0.1, "Stepsize"=0.0001, "Invert Axis"=TRUE, "Invert Direction X"=FALSE, "Invert Direction Y"=TRUE, "enable feedback"=FALSE, "Set Centriod Target"=FALSE}, {"Tolerance [%]"=0.1, "Stepsize"=0.0001, "Invert Axis"=TRUE, "Invert Direction X"=FALSE, "Invert Direction Y"=TRUE, "enable feedback"=FALSE, "Set Centriod Target"=FALSE}]
  in  "Time":timestamp[][](array[timestamp])
  in  "Mean Size":dbl[][](array[numeric])
  in  "Size":dbl[][](array[numeric])
  in  "active CCDs":i32(listbox)=1
  in  "Offset Y":dbl[][](array[numeric])
  in  "Offset X":dbl[][](array[numeric])
  in  "Mean Centroid X":dbl[][](array[numeric])
  in  "Mean Centroid Y":dbl[][](array[numeric])
  in  "Centroid Y":dbl[][](array[numeric])
  in  "Centroid X":dbl[][](array[numeric])
  in  "GUIdevice 7":string="B2_TelLens1"
  in  "GUIdevice 6":string="B1_TelInput"
  in  "GUIdevice 5":string="L8_M10Leak"
  in  "GUIdevice 4":string="L7_TREXPass4"
  in  "GUIdevice 3":string="L6_TREXpass3"
  in  "GUIdevice 2":string="L5_TREXPass2"
  in  "insert tag":bool=TRUE
  in  "stop":bool
  in  "GUIdevice 1":string="L4_TREXpass1"
  out "tcp data event":T13
  out "error IO 2":errorcluster
  # "x [Tolerance]"
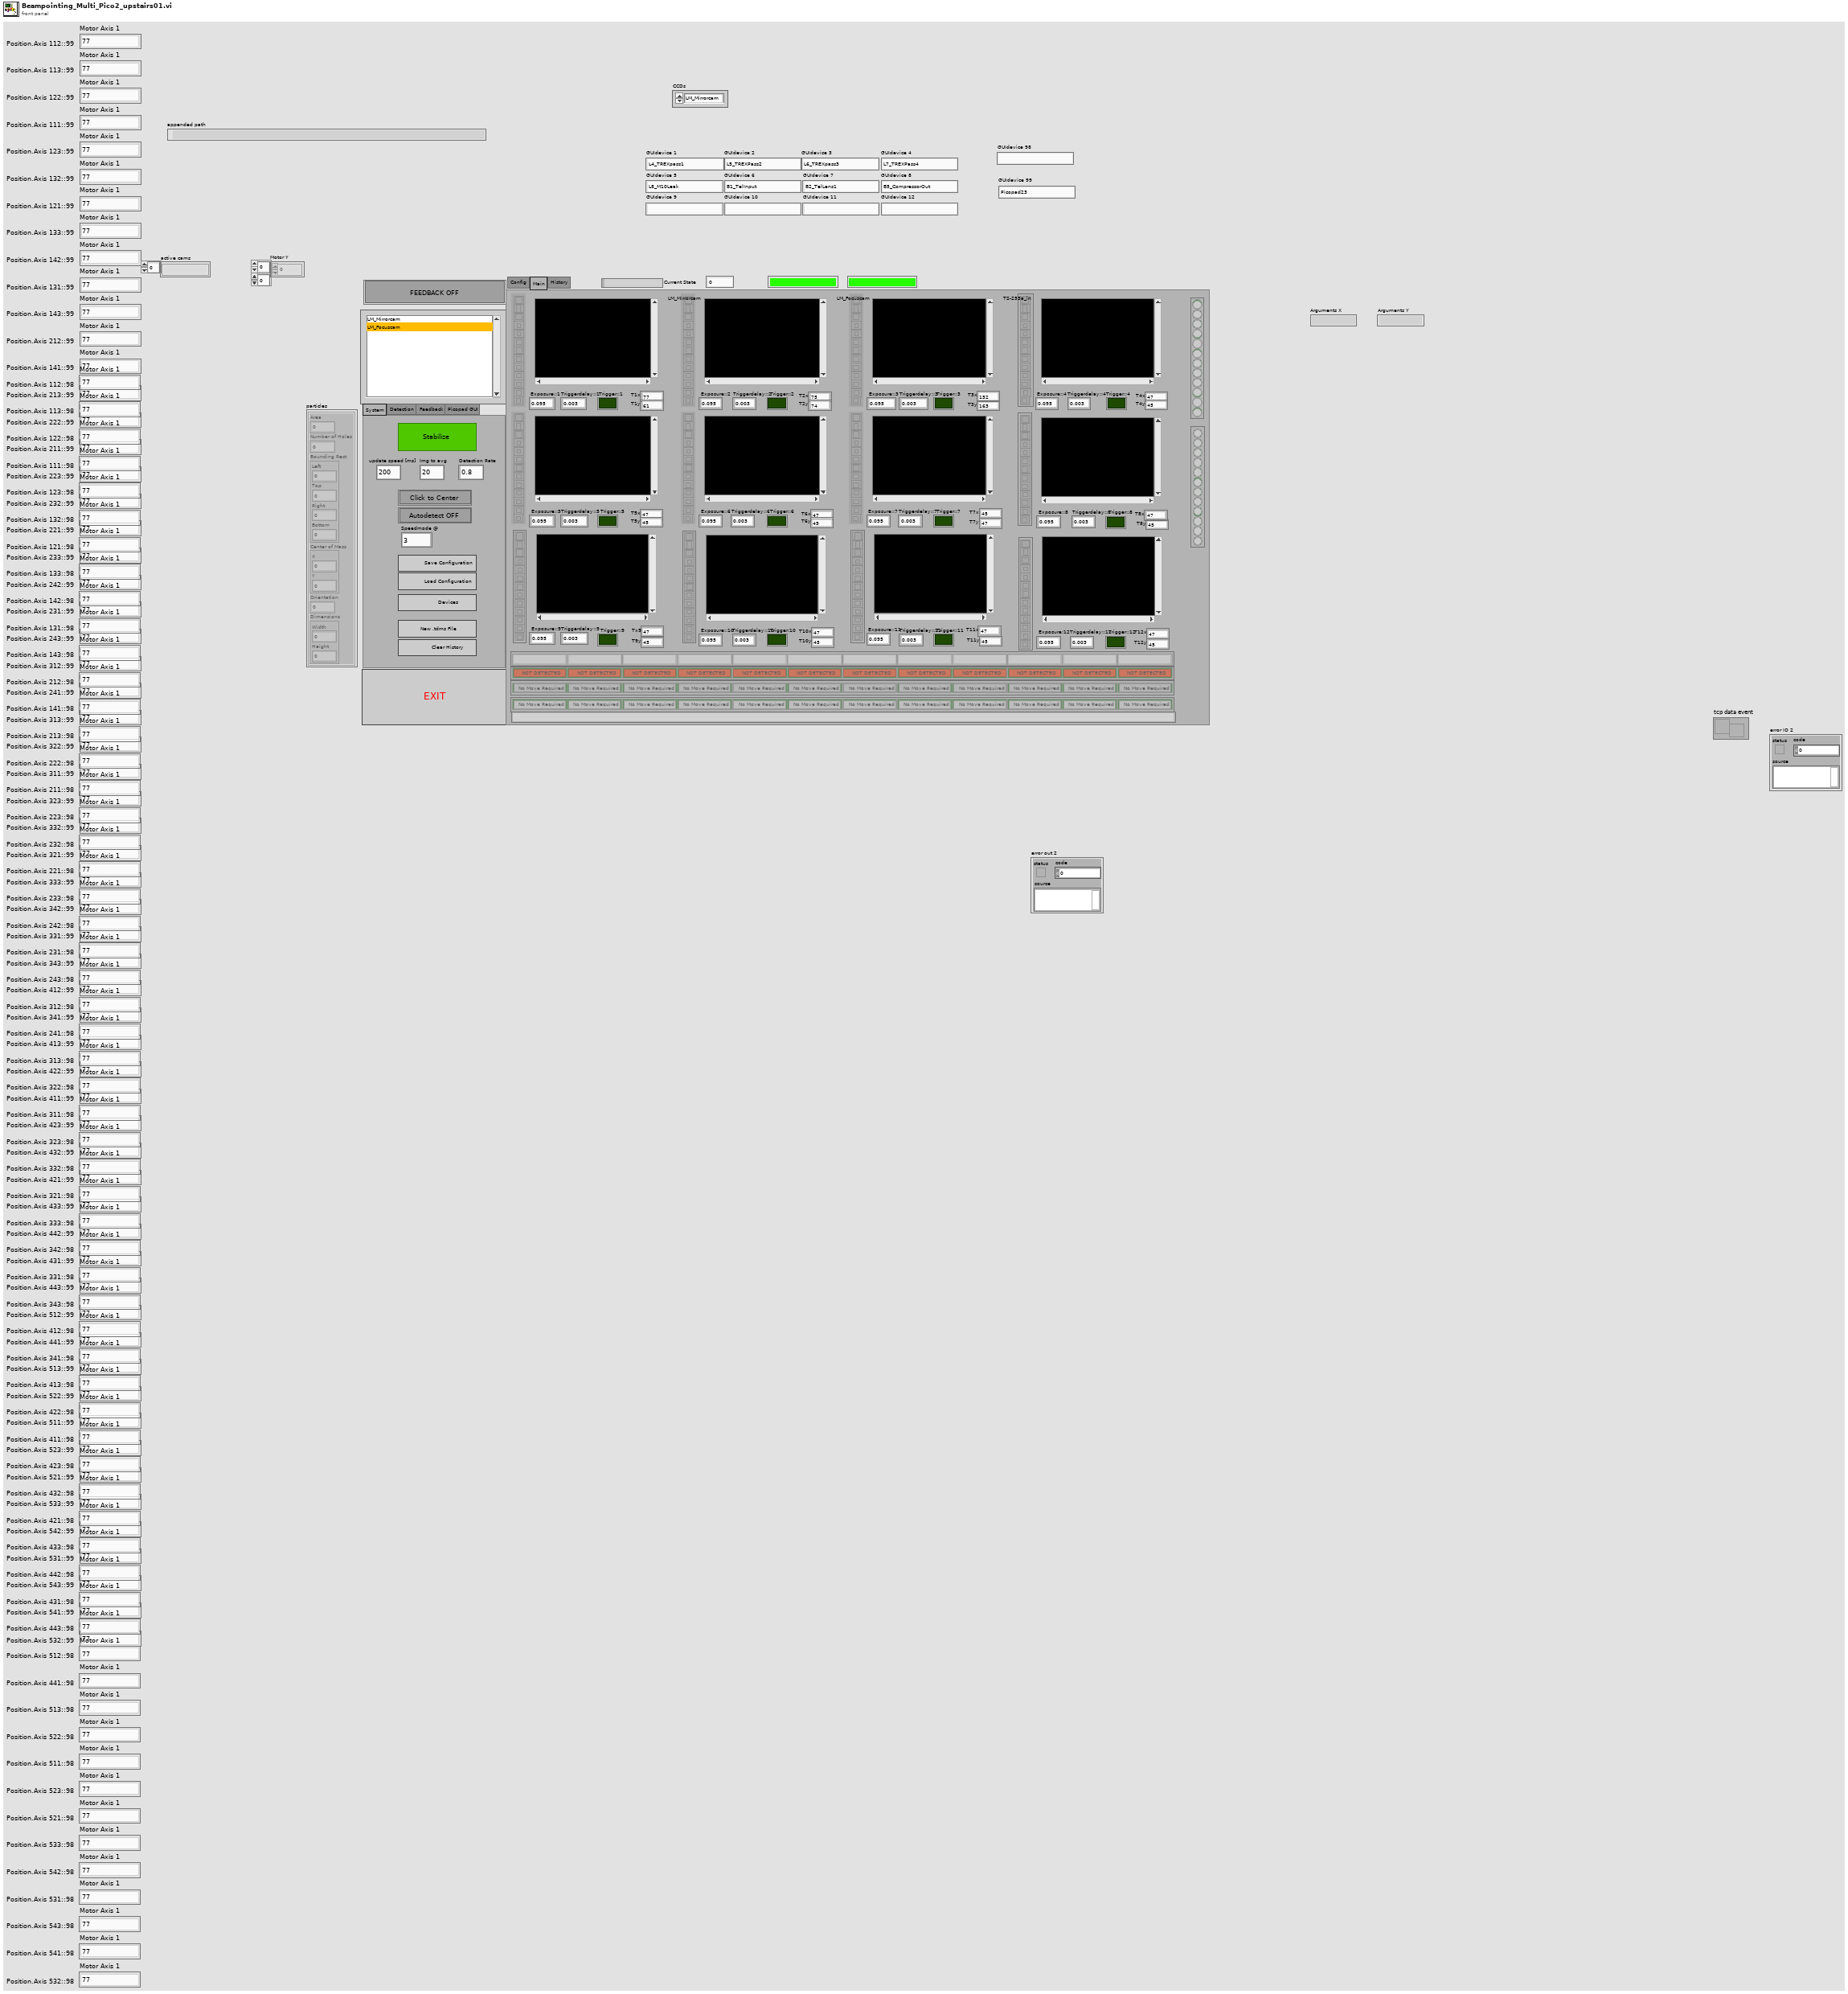
[diagram p1: front panel]
types:
  T1 = cluster{"Area":dbl, "Number of Holes":dbl, "Bounding Rect":cluster{"Left":dbl, "Top":dbl, "Right":dbl, "Bottom":dbl}, "Center of Mass":cluster{"X":dbl, "Y":dbl}, "Orientation":dbl, "Dimensions":cluster{"Width":dbl, "Height":dbl}}[]
  T2 = typedef "move.ctl" = cluster{"Tolerance [%]":dbl, "Stepsize":dbl, "Invert Axis":bool, "Invert Direction X":bool, "Invert Direction Y":bool, "enable feedback":bool, "Set Centriod Target":bool}
  T3 = typedef "beam detection.ctl" = cluster{"Filter":u16, "Filter Para":cluster{"X Size":i32, "Y Size":i32, "% Tolerance":i32}, "detection method":i32, "smal para":cluster{"Measurement Parameter":T4, "Range Lower Value":dbl, "Range Upper Value":dbl, "Range":bool, "Measurement Type":bool}[], "Remove small Objects":bool, "Restrict to round Objects":bool}
  T4 = typedef "Particle Parameters" = i32
  T5 = cluster{"CCDs":string[], "move properties":T2[], "detection para":T3[], "thresholds":cluster{"Lower value":sgl, "Upper value":sgl}[], "Value":cluster{"Motor CCD 1":u16, "Motor CCD 2":u16, "Motor CCD 3":u16, "Motor CCD 4":u16, "Motor CCD 5":u16, "Motor CCD 6":u16, "Motor CCD 7":u16, "Motor CCD 8":u16, "Motor CCD 9":u16, "Motor CCD 10":u16, "Motor CCD 11":u16, "Motor CCD 12":u16}}
  T6 = cluster{"Left":dbl, "Top":dbl, "Right":dbl, "Bottom":dbl}[]
  T7 = cluster{"Motor CCD 1":u16, "Motor CCD 2":u16, "Motor CCD 3":u16, "Motor CCD 4":u16, "Motor CCD 5":u16, "Motor CCD 6":u16, "Motor CCD 7":u16, "Motor CCD 8":u16, "Motor CCD 9":u16, "Motor CCD 10":u16, "Motor CCD 11":u16, "Motor CCD 12":u16}
  T8 = cluster{"[0]":string, "[1]":string, "[2]":string, "[3]":string, "[4]":string, "[5]":string, "[6]":string, "[7]":string, "[8]":string, "[8] 2":string, "[8] 3":string, "[8] 4":string}
  T9 = typedef "IMAQ Image.ctl" = refnum<image>
  T10 = cluster{"Area":dbl, "Number of Holes":dbl, "Bounding Rect":cluster{"Left":dbl, "Top":dbl, "Right":dbl, "Bottom":dbl}, "Center of Mass":cluster{"X":dbl, "Y":dbl}, "Orientation":dbl, "Dimensions":cluster{"Width":dbl, "Height":dbl}}[][]
  T11 = enum32{"System", "Detection", "Feedback", "Picopad GUI"}
  T12 = cluster{"Ref X":refnum<vi>, "Ref Y":refnum<vi>}[]
  T13 = typedef "tcp_new_data_event.ctl" = refnum<user-event>
  T14 = typedef "tcp new data cluster.ctl" = cluster{"EventEnum":enum16{"new data", "connection status update"}, "Device name":string}
  T15 = cluster{"Left":i32, "Top":i32, "Right":i32, "Bottom":i32}
  T16 = enum32{"invalid app kind", "Development System", "Run Time System", "Student Edition", "Embedded LabVIEW", "Evaluation", "Custom"}
  T17 = enum16{"open", "open or create", "create or replace", "create", "open (read-only)"}
  T18 = enum32{"Invalid", "Standard", "Closed", "Hidden", "Minimized", "Maximized"}
  T19 = enum16{"open", "replace", "create", "open or create", "replace or create", "replace or create with confirmation"}
  T20 = typedef "Image Type" = u32
  T21 = cluster{"[0]":string, "[1]":string, "[2]":string, "[3]":string, "[4]":string, "[5]":string, "[6]":string, "[7]":string, "[8]":string, "[9]":string, "[10]":string, "[11]":string}
  T22 = cluster{"Target.X::1":refnum<vi>, "Target.Y::1":refnum<vi>}
  T23 = cluster{"Target.X::2":refnum<vi>, "Target.Y::2":refnum<vi>}
  T24 = cluster{"Target.X::3":refnum<vi>, "Target.Y::3":refnum<vi>}
  T25 = cluster{"Target.X::4":refnum<vi>, "Target.Y::4":refnum<vi>}
  T26 = cluster{"Target.X::5":refnum<vi>, "Target.Y::5":refnum<vi>}
  T27 = cluster{"Target.X::6":refnum<vi>, "Target.Y::6":refnum<vi>}
  T28 = cluster{"Target.X::7":refnum<vi>, "Target.Y::7":refnum<vi>}
  T29 = cluster{"Target.X::8":refnum<vi>, "Target.Y::8":refnum<vi>}
  T30 = cluster{"Target.X::12":refnum<vi>, "Target.Y::12":refnum<vi>}
  T31 = cluster{"Target.X::9":refnum<vi>, "Target.Y::9":refnum<vi>}
  T32 = cluster{"Target.X::10":refnum<vi>, "Target.Y::10":refnum<vi>}
  T33 = cluster{"Target.X::11":refnum<vi>, "Target.Y::11":refnum<vi>}
  T34 = cluster{"Target.X::12":refnum<vi>, "Target.Y::12":refnum<vi>}[]
  T35 = cluster{"Left":dbl, "Top":dbl, "Right":dbl, "Bottom":dbl}
  T36 = cluster{"Core":cluster{"Current VI Reference":refnum<vi>, "Close Panel on Exit?":bool}, "detection para":T3[], "thresholds":cluster{"Lower value":sgl, "Upper value":sgl}[], "Centroid X":dbl[][], "Centroid Y":dbl[][], "img to avg":i32, "Mean Centroid X":dbl[][], "Mean Centroid Y":dbl[][], "Offset X":dbl[][], "Offset Y":dbl[][], "Offset X stats ":dbl[][], "Offset Y stats ":dbl[][], "Size":dbl[][], "Mean Size":dbl[][], "Time":timestamp[][], "move properties":T2[], "active axis refs 2":cluster{"Ref X":refnum<vi>, "Ref Y":refnum<vi>}[], "active ccd":i32, "Feedback global":bool, "Motor X":dbl[][], "Motor Y":dbl[][], "active cams":string[], "Data Value Reference out":refnum<k34>, "detected":bool[], "speedmode X":bool[], "speedmode Y":bool[]}
  T37 = cluster{"Current VI Reference":refnum<vi>, "Close Panel on Exit?":bool}
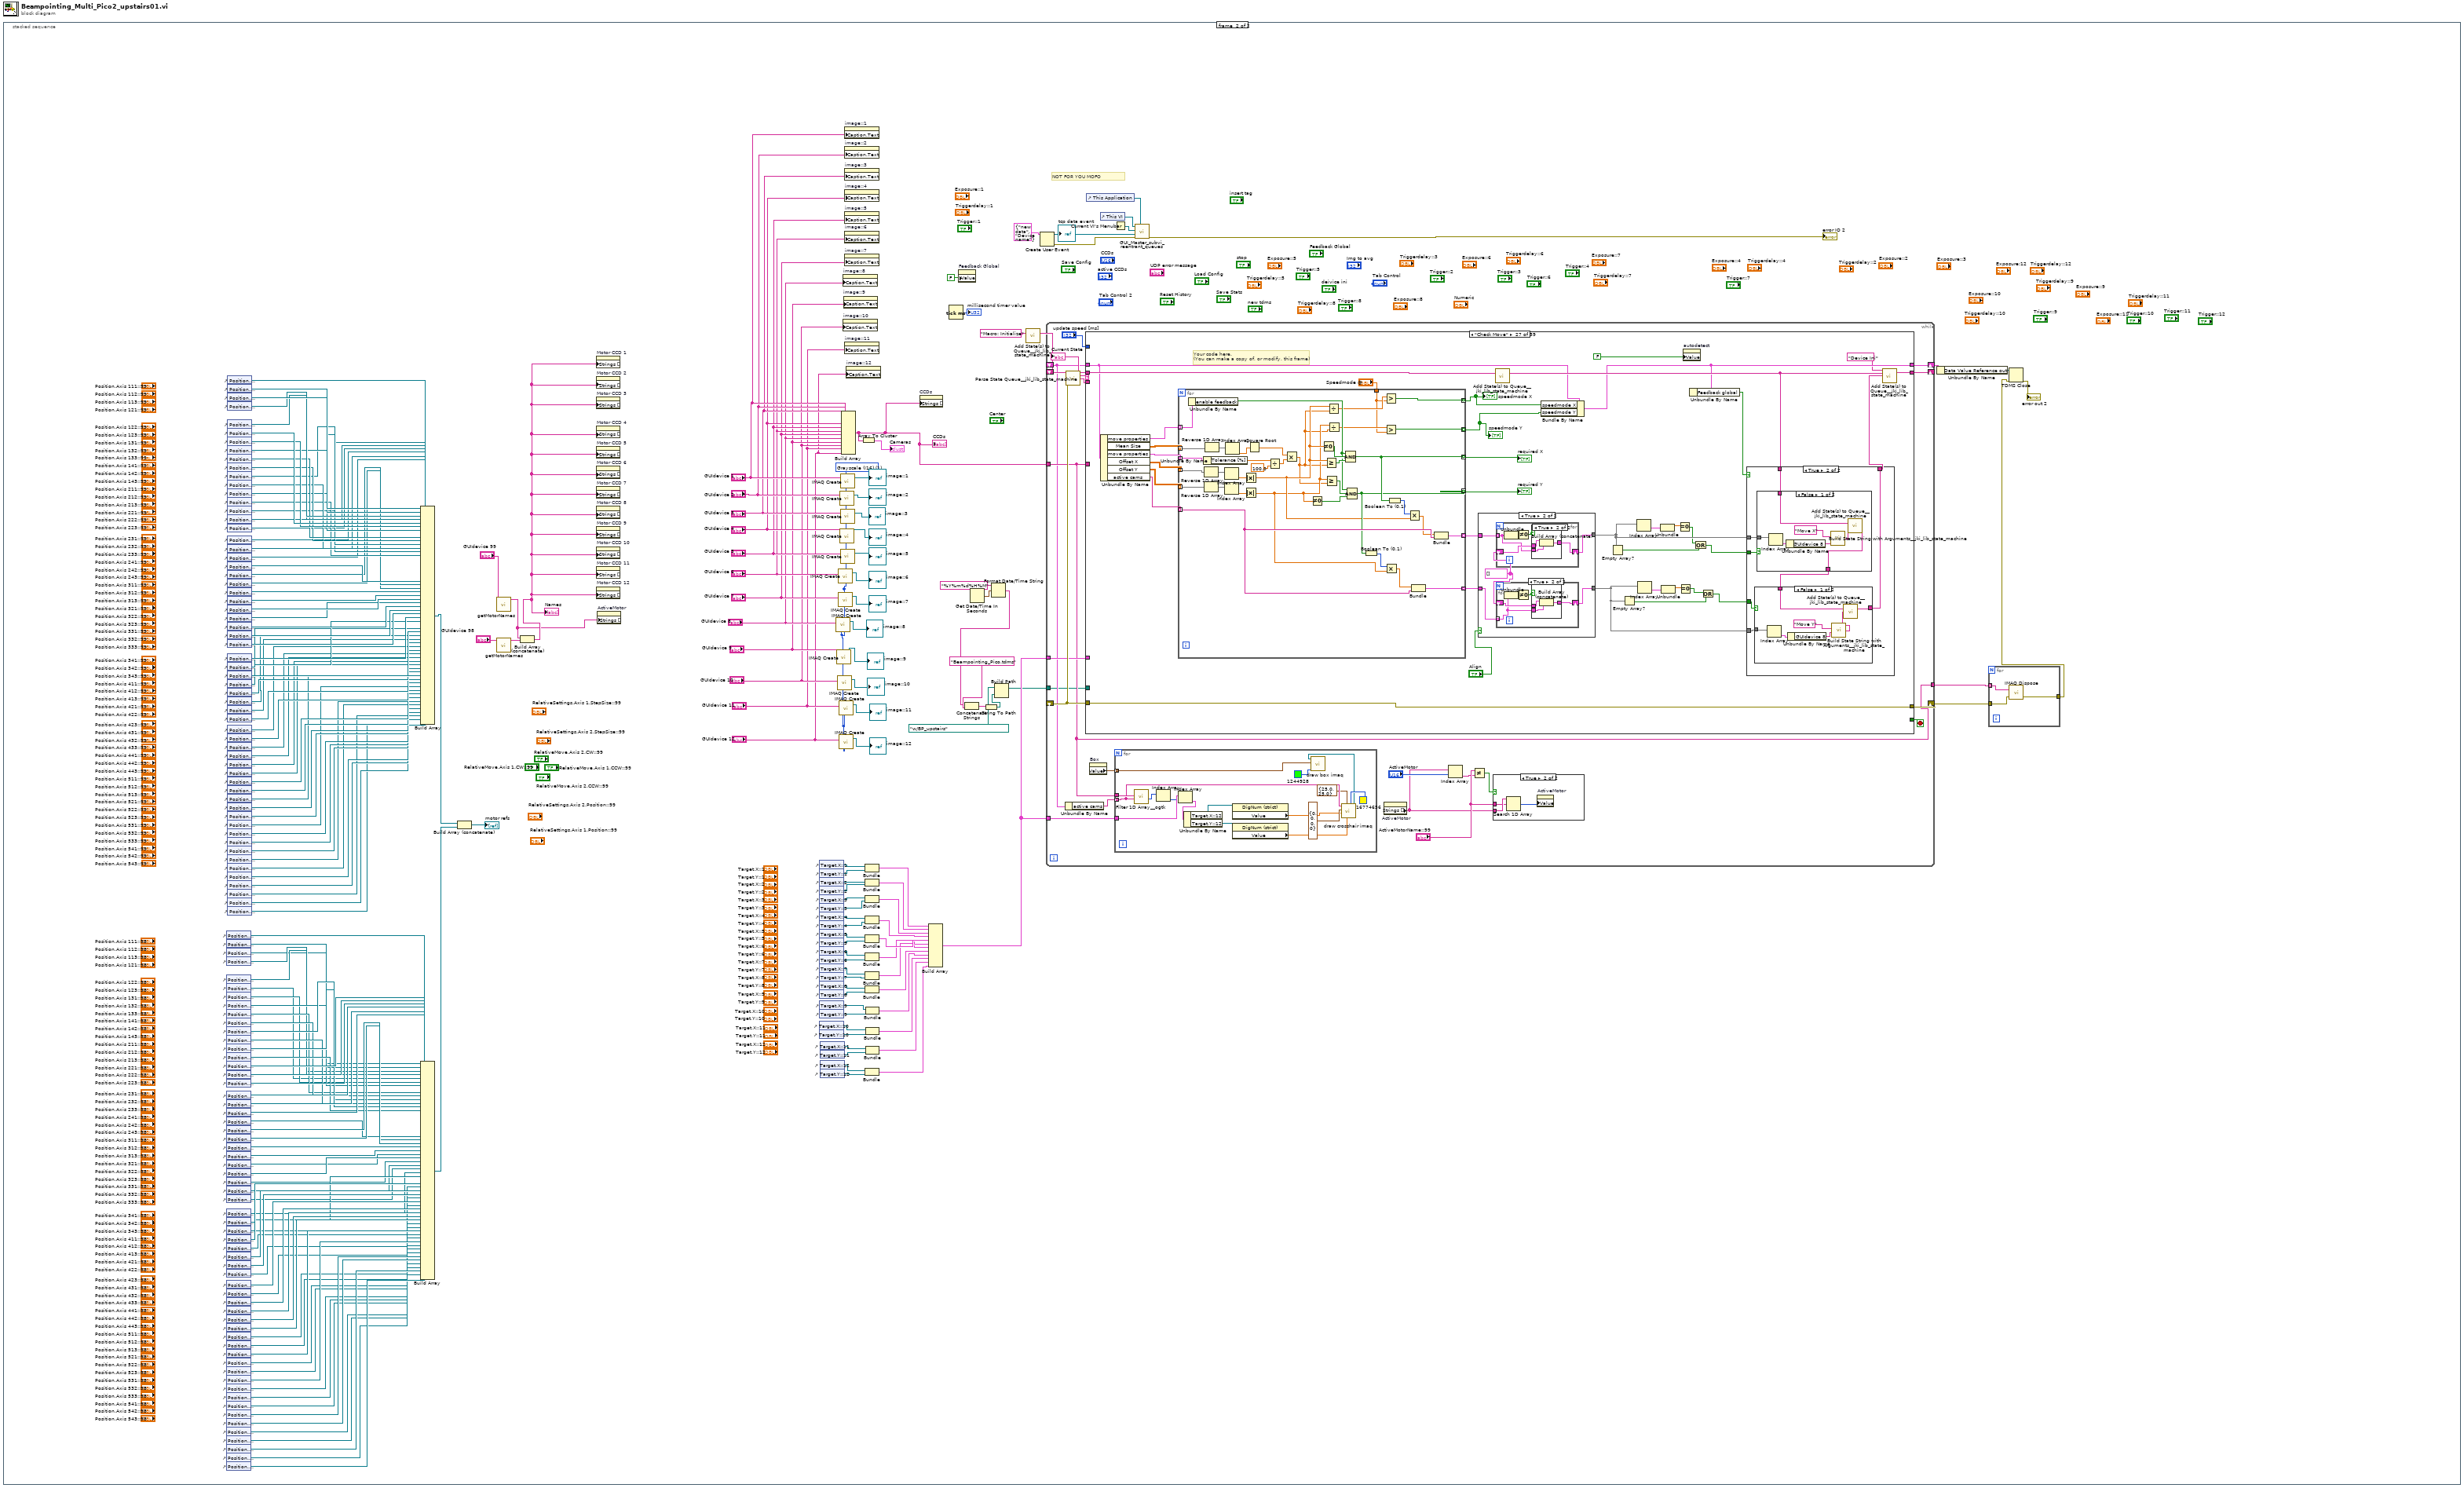
[diagram p0: block diagram]
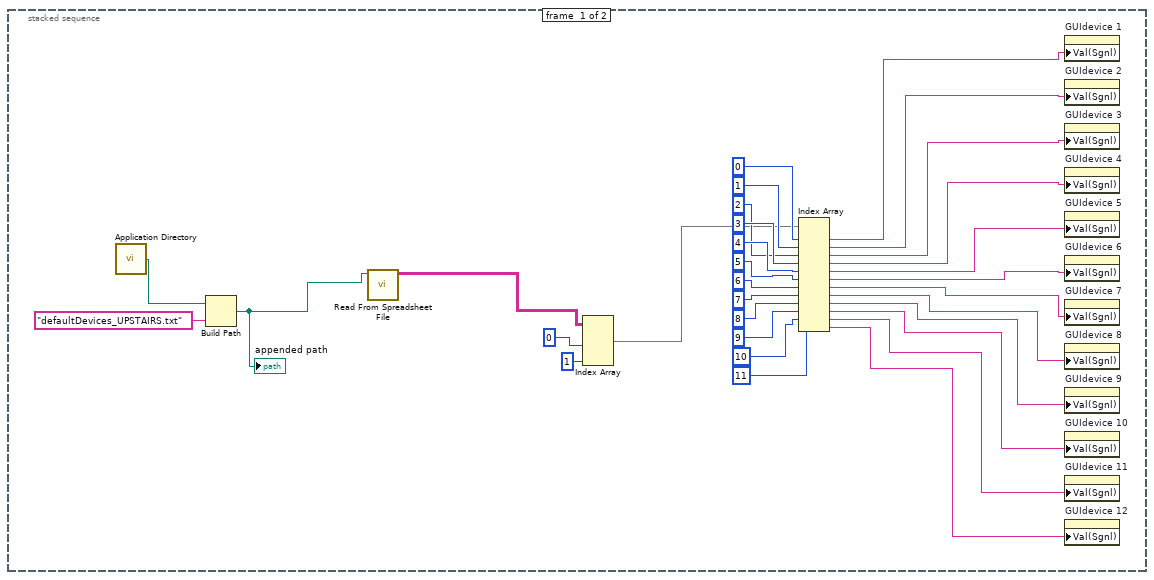
[diagram p2: hidden frame]
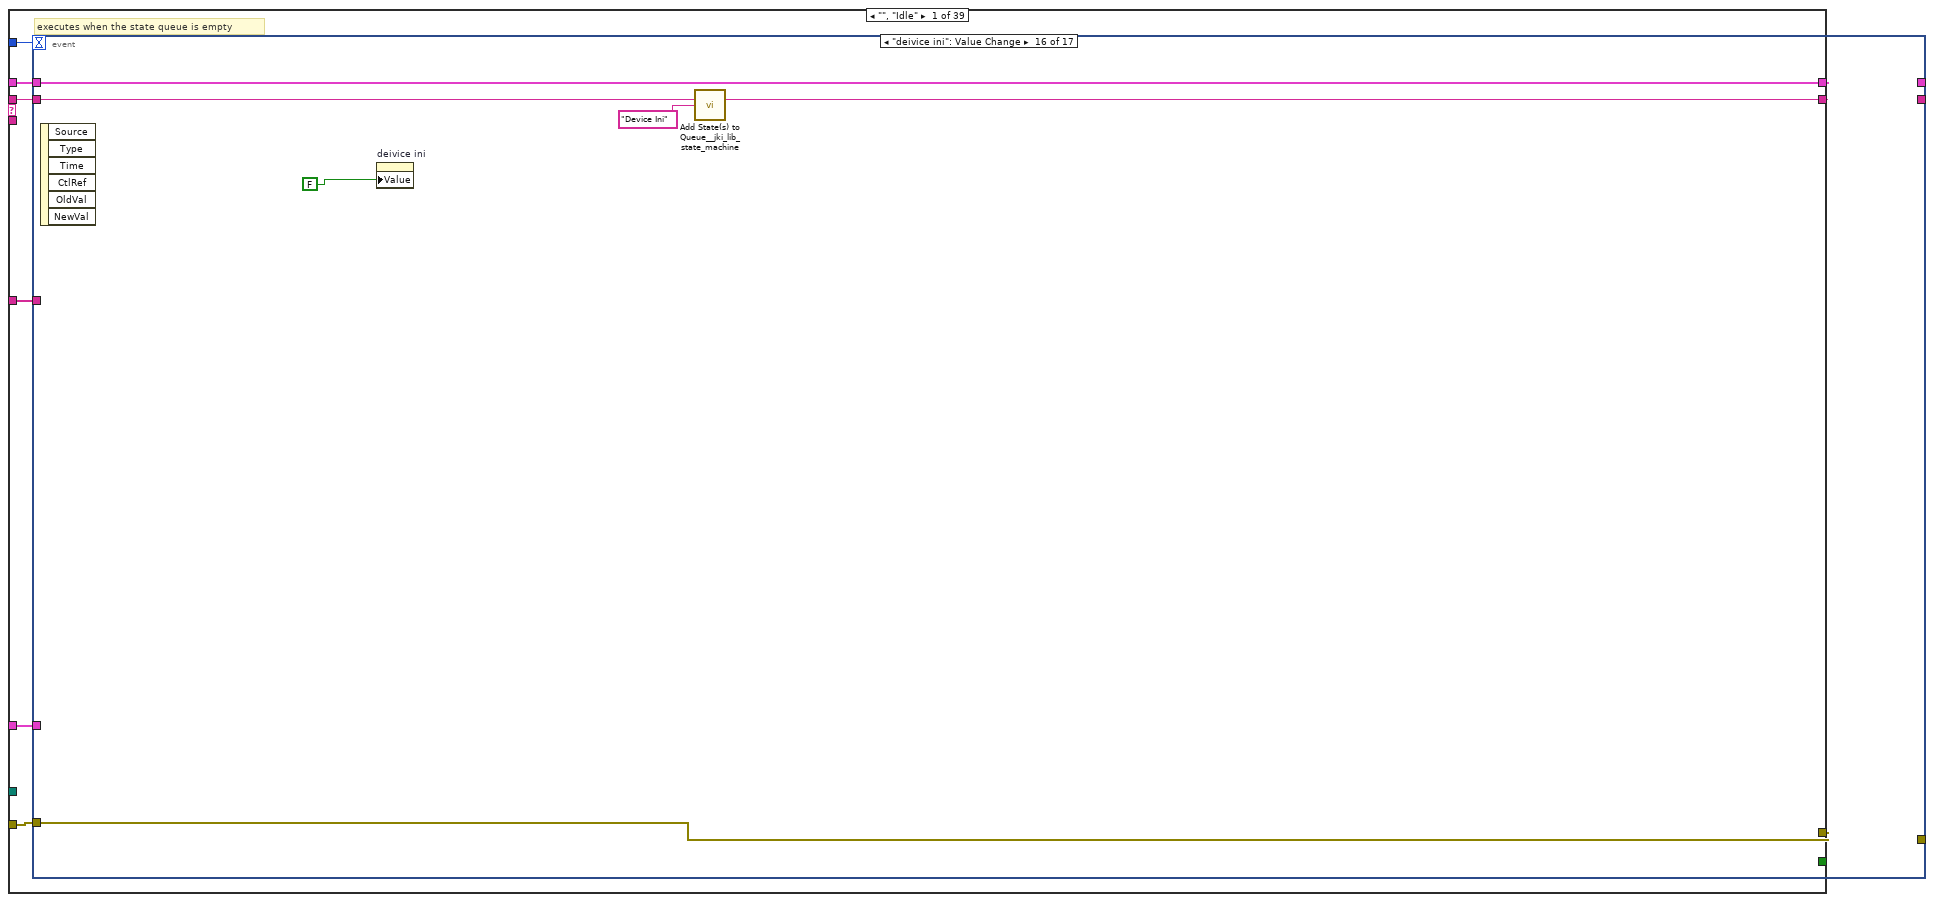
[diagram p4: hidden frame]
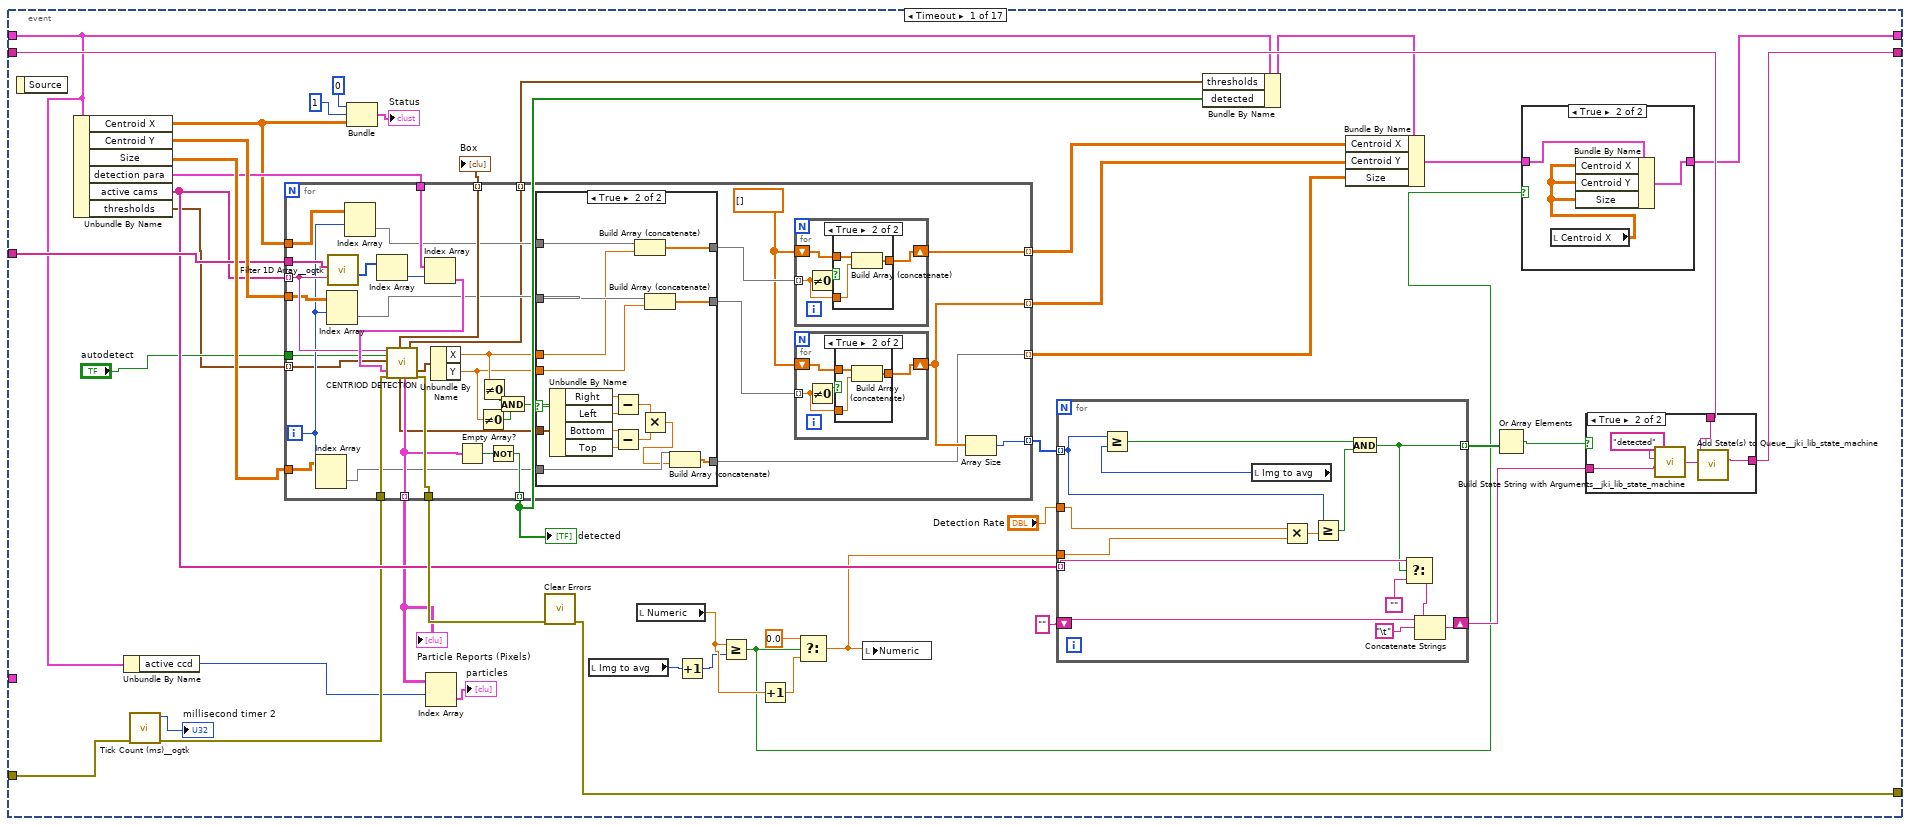
[diagram p5: hidden frame]
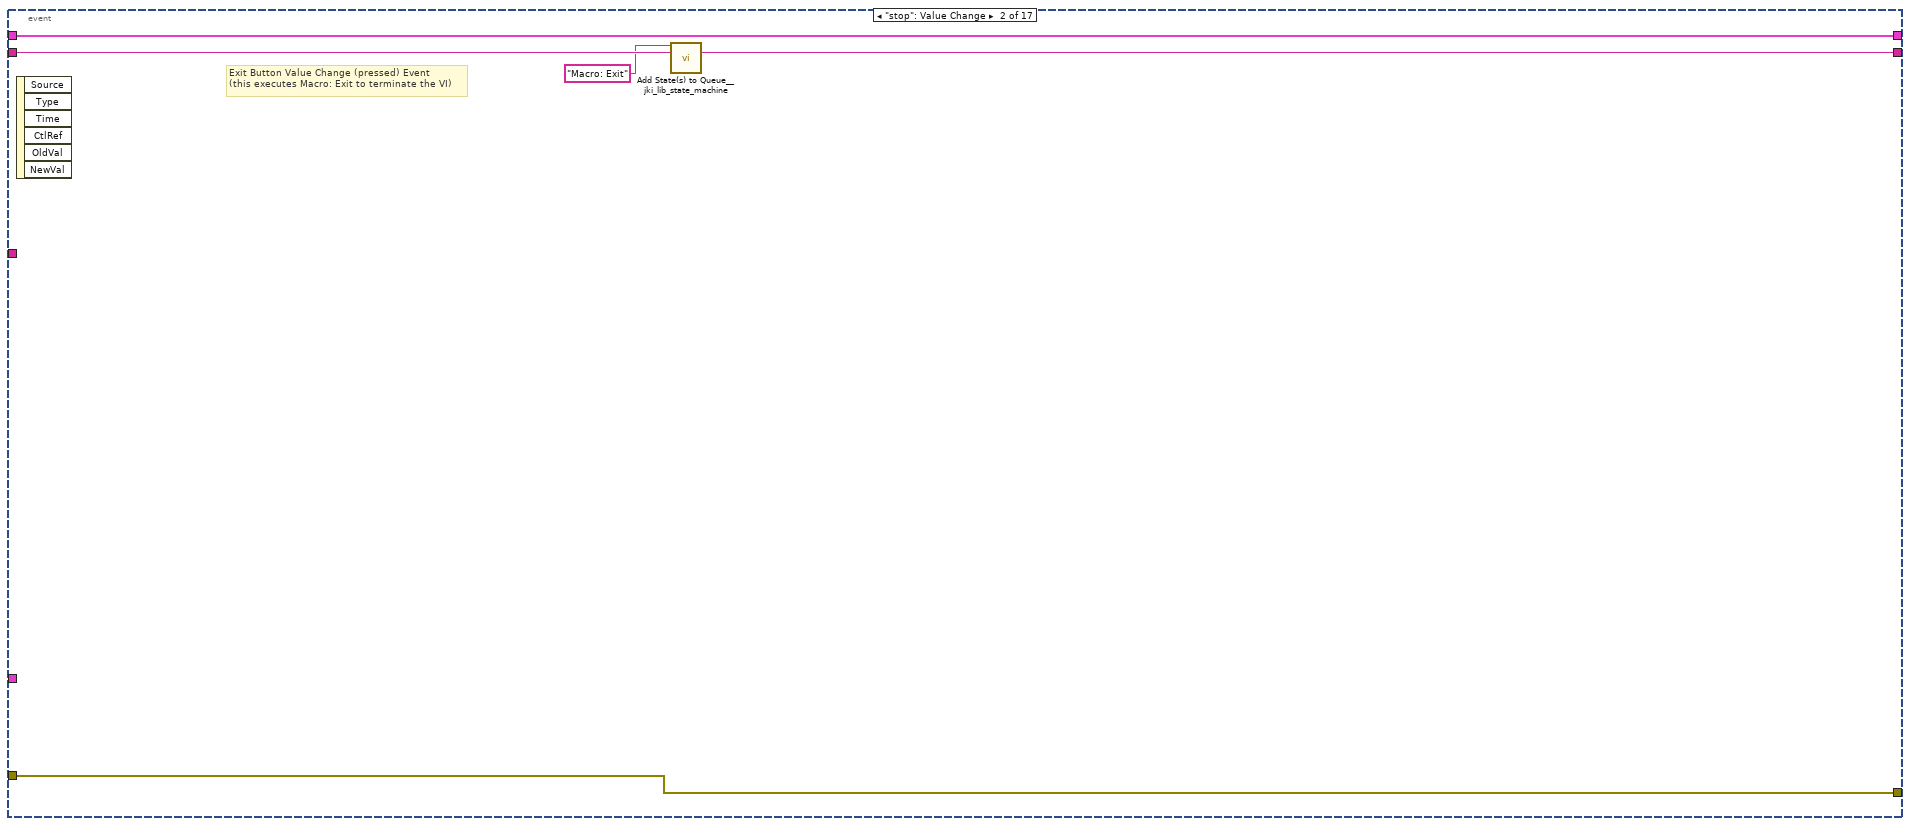
[diagram p11: hidden frame]
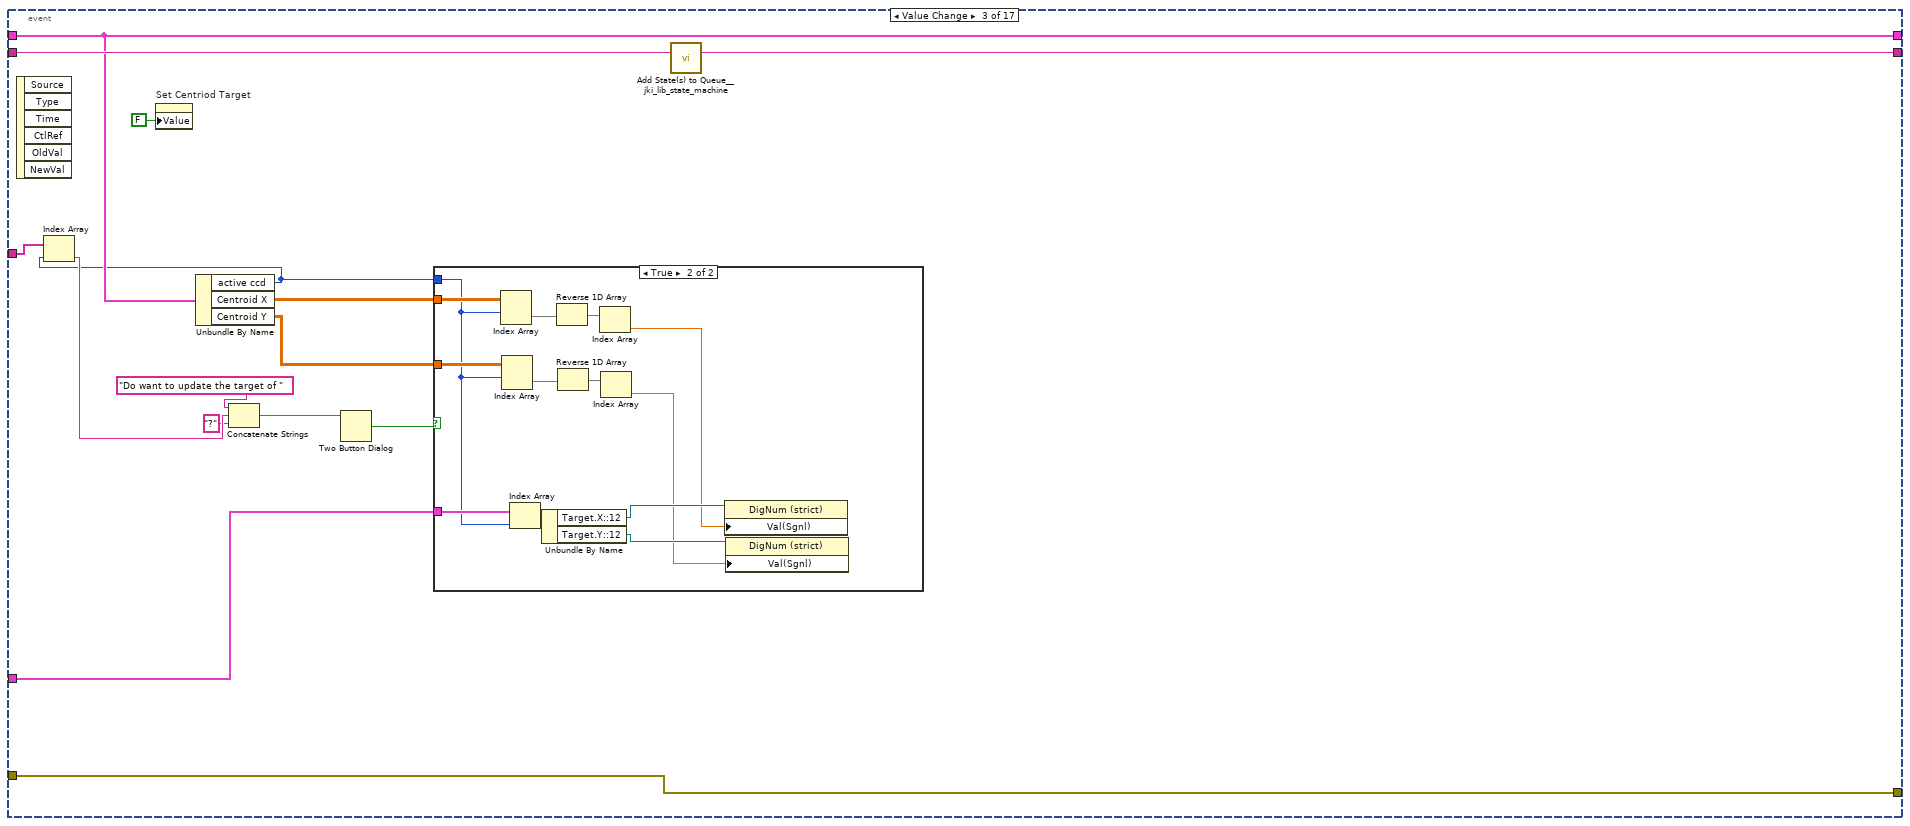
[diagram p12: hidden frame]
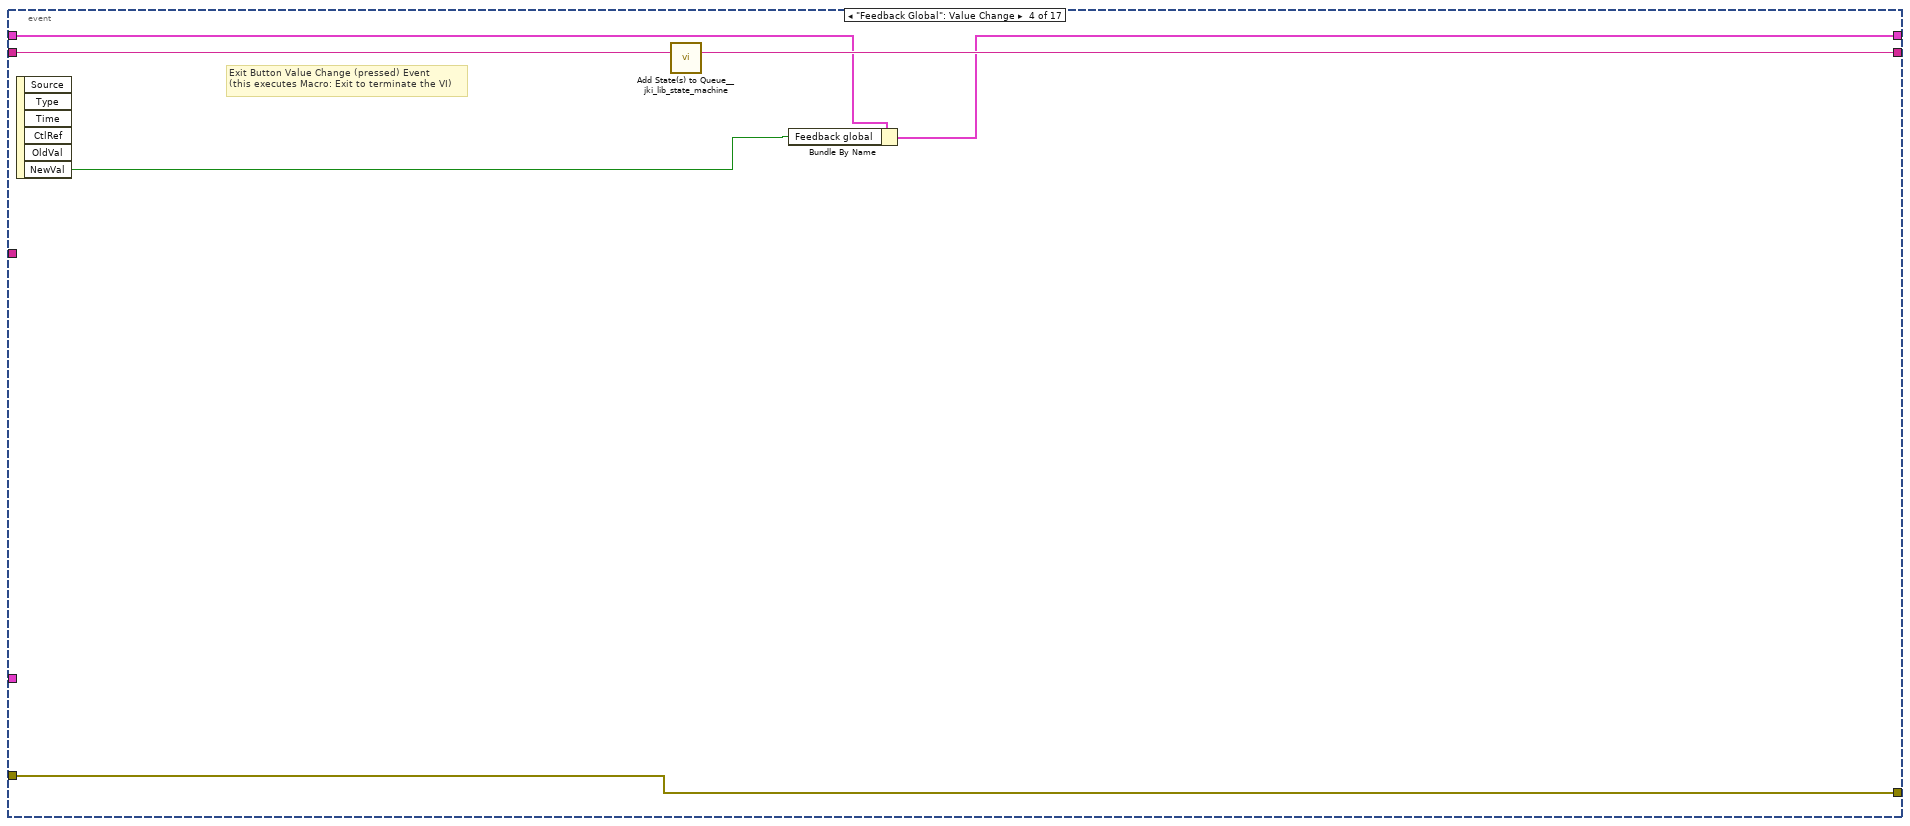
[diagram p14: hidden frame]
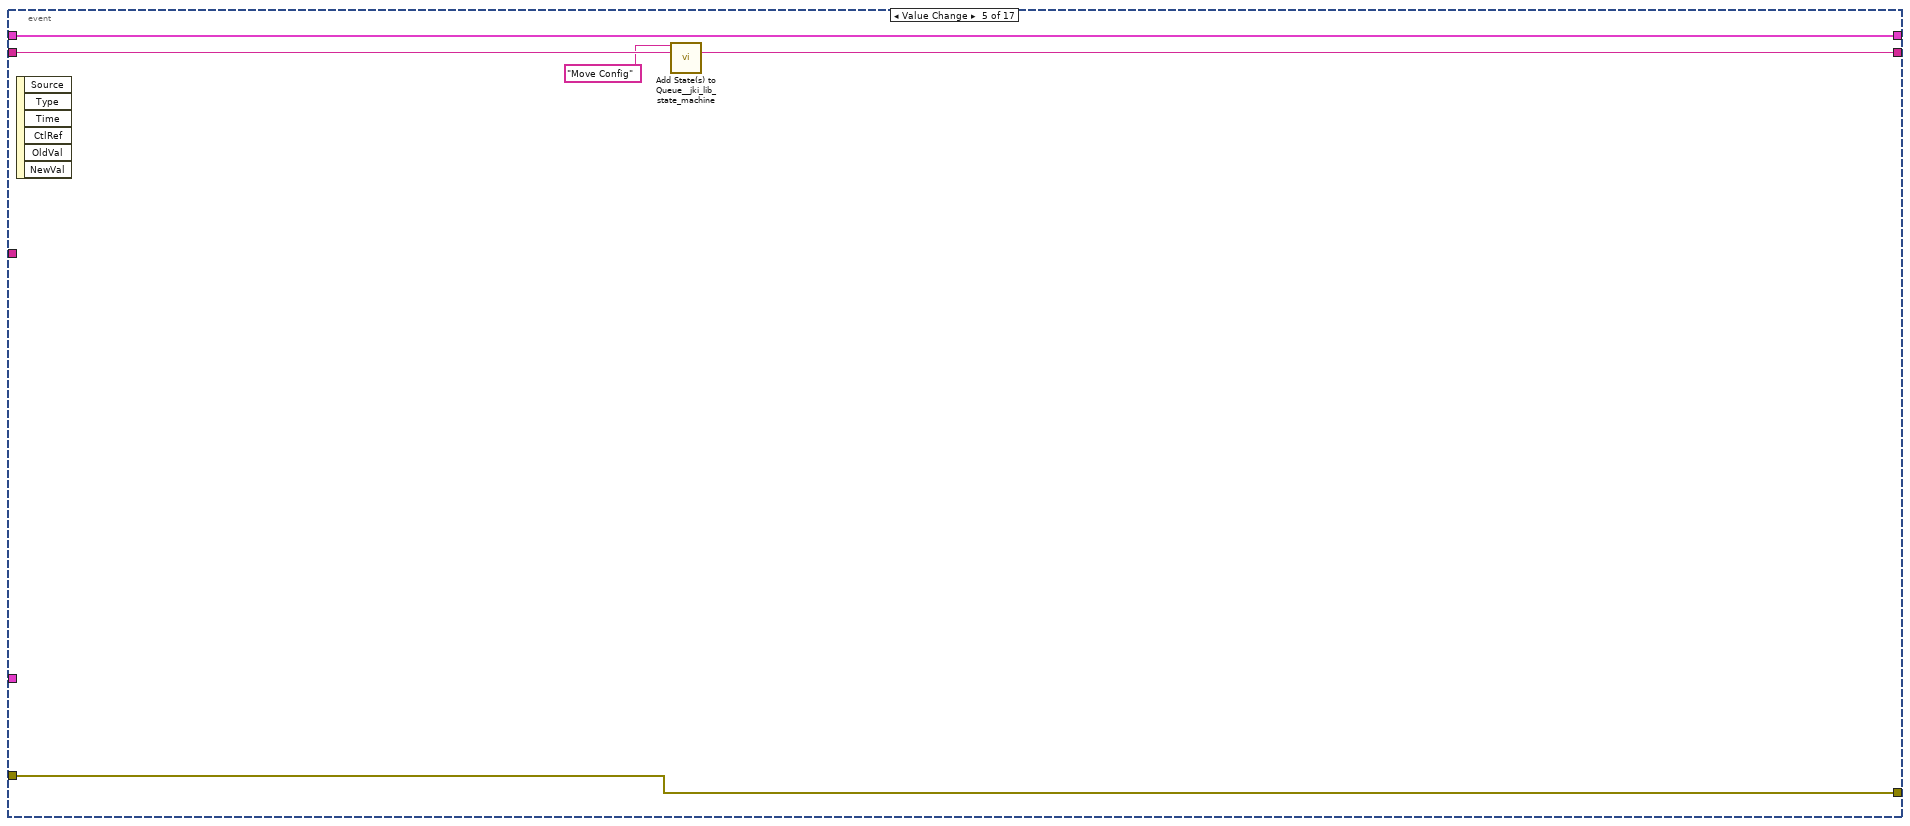
[diagram p15: hidden frame]
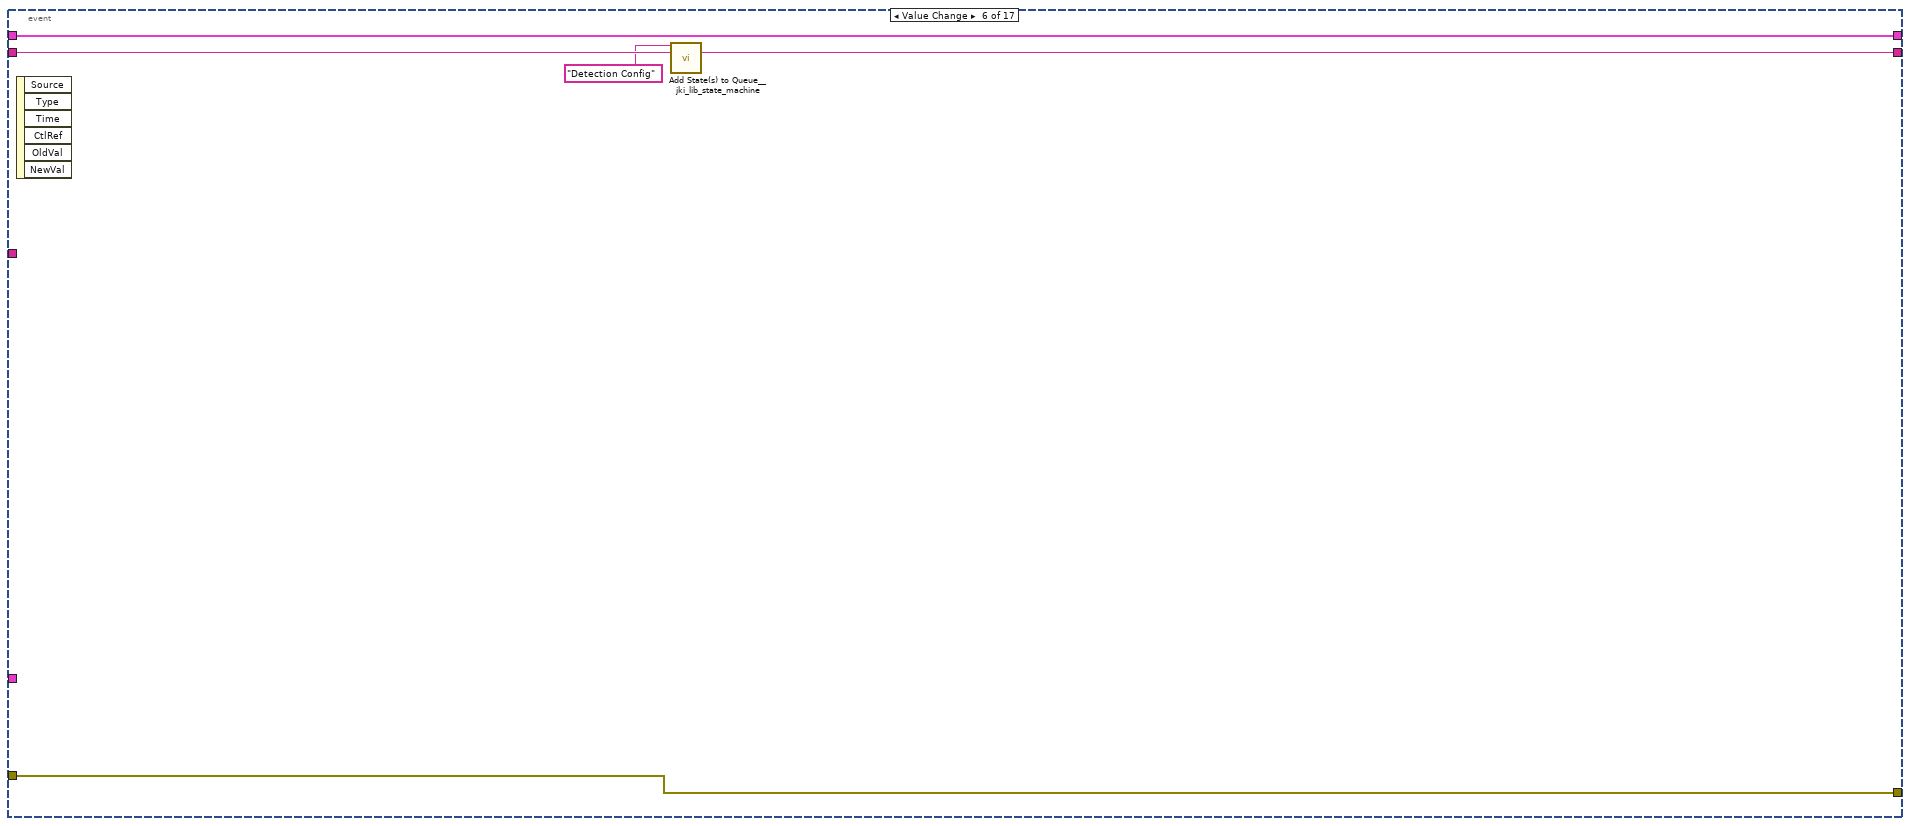
[diagram p16: hidden frame]
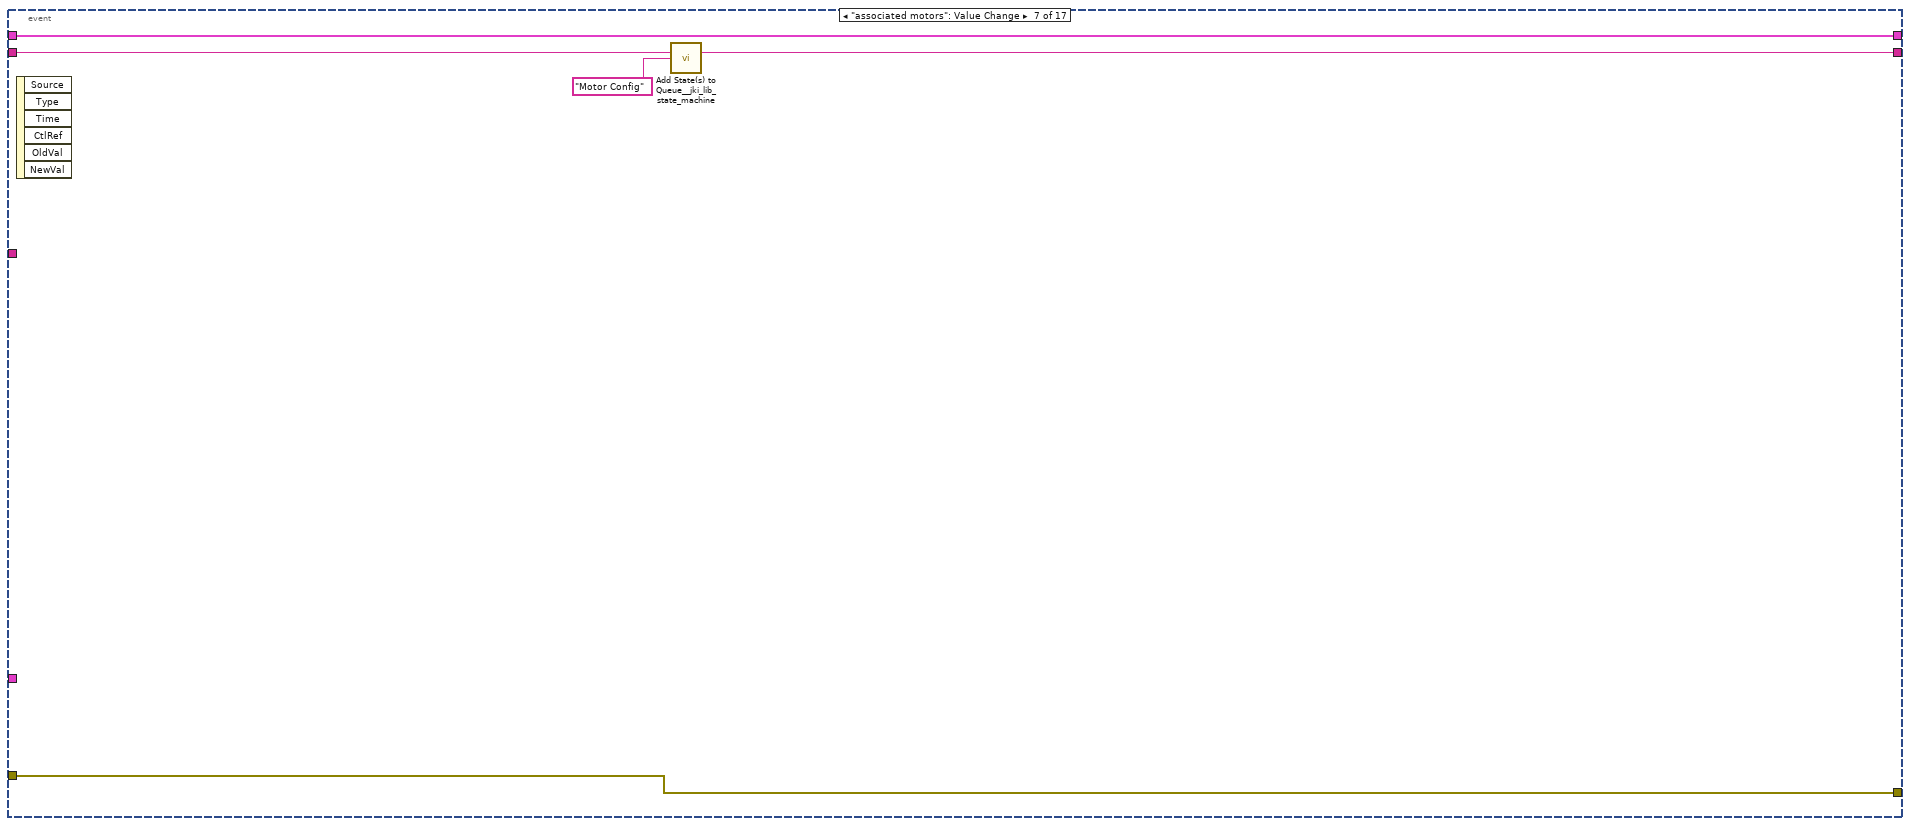
[diagram p17: hidden frame]
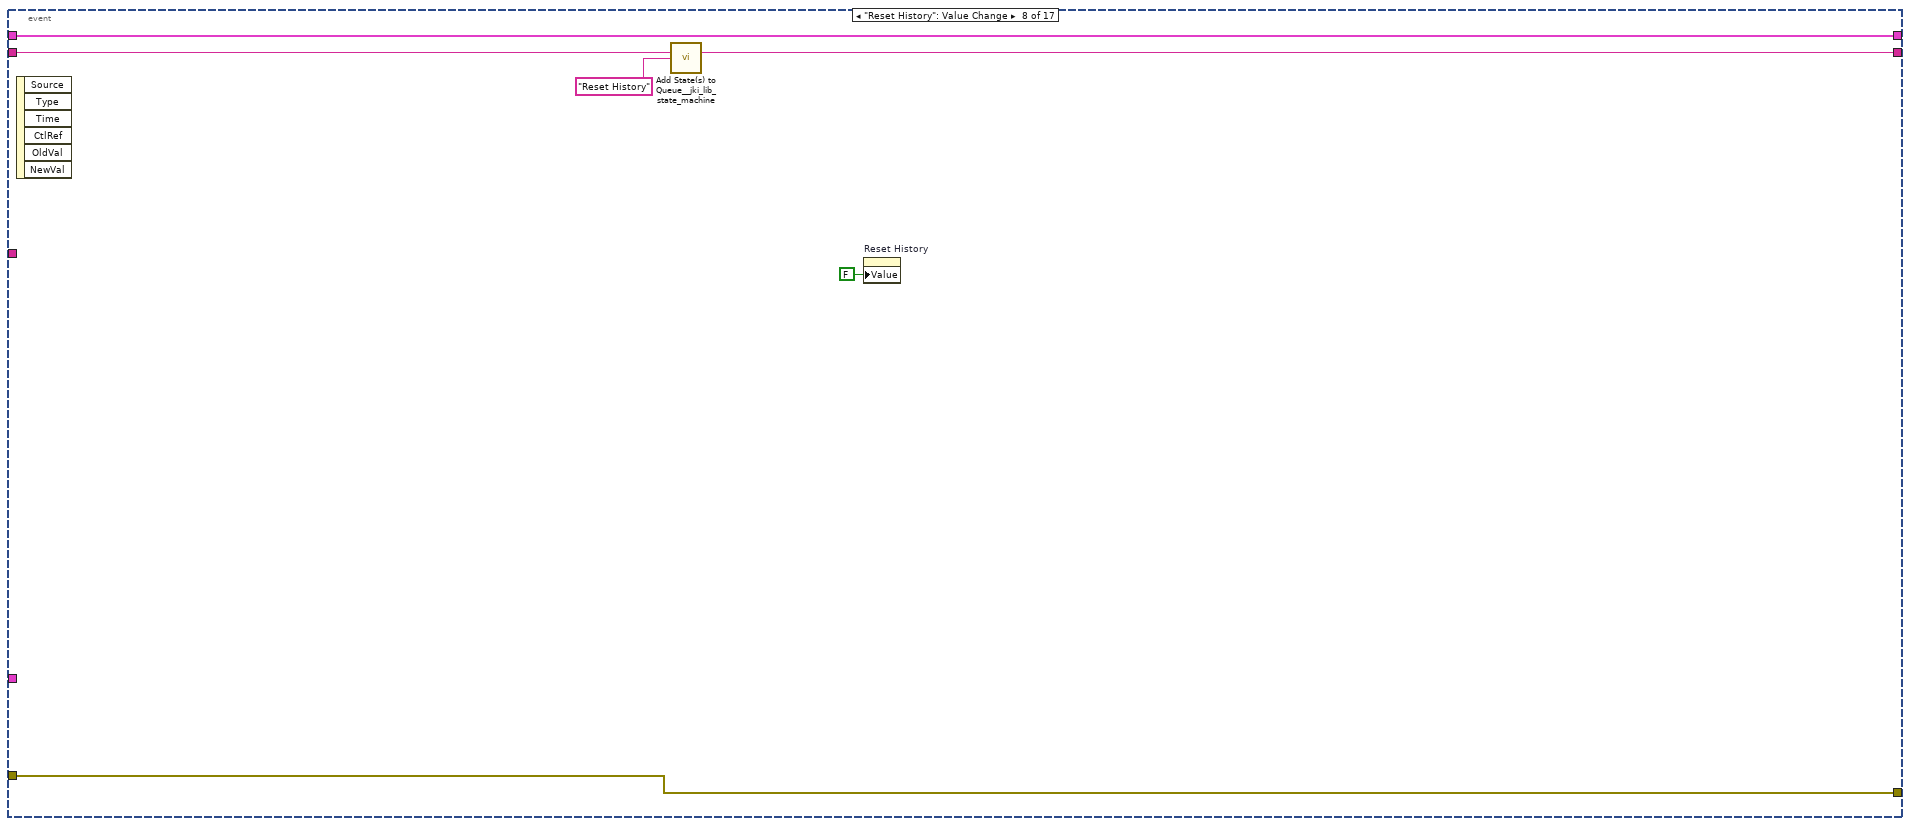
[diagram p18: hidden frame]
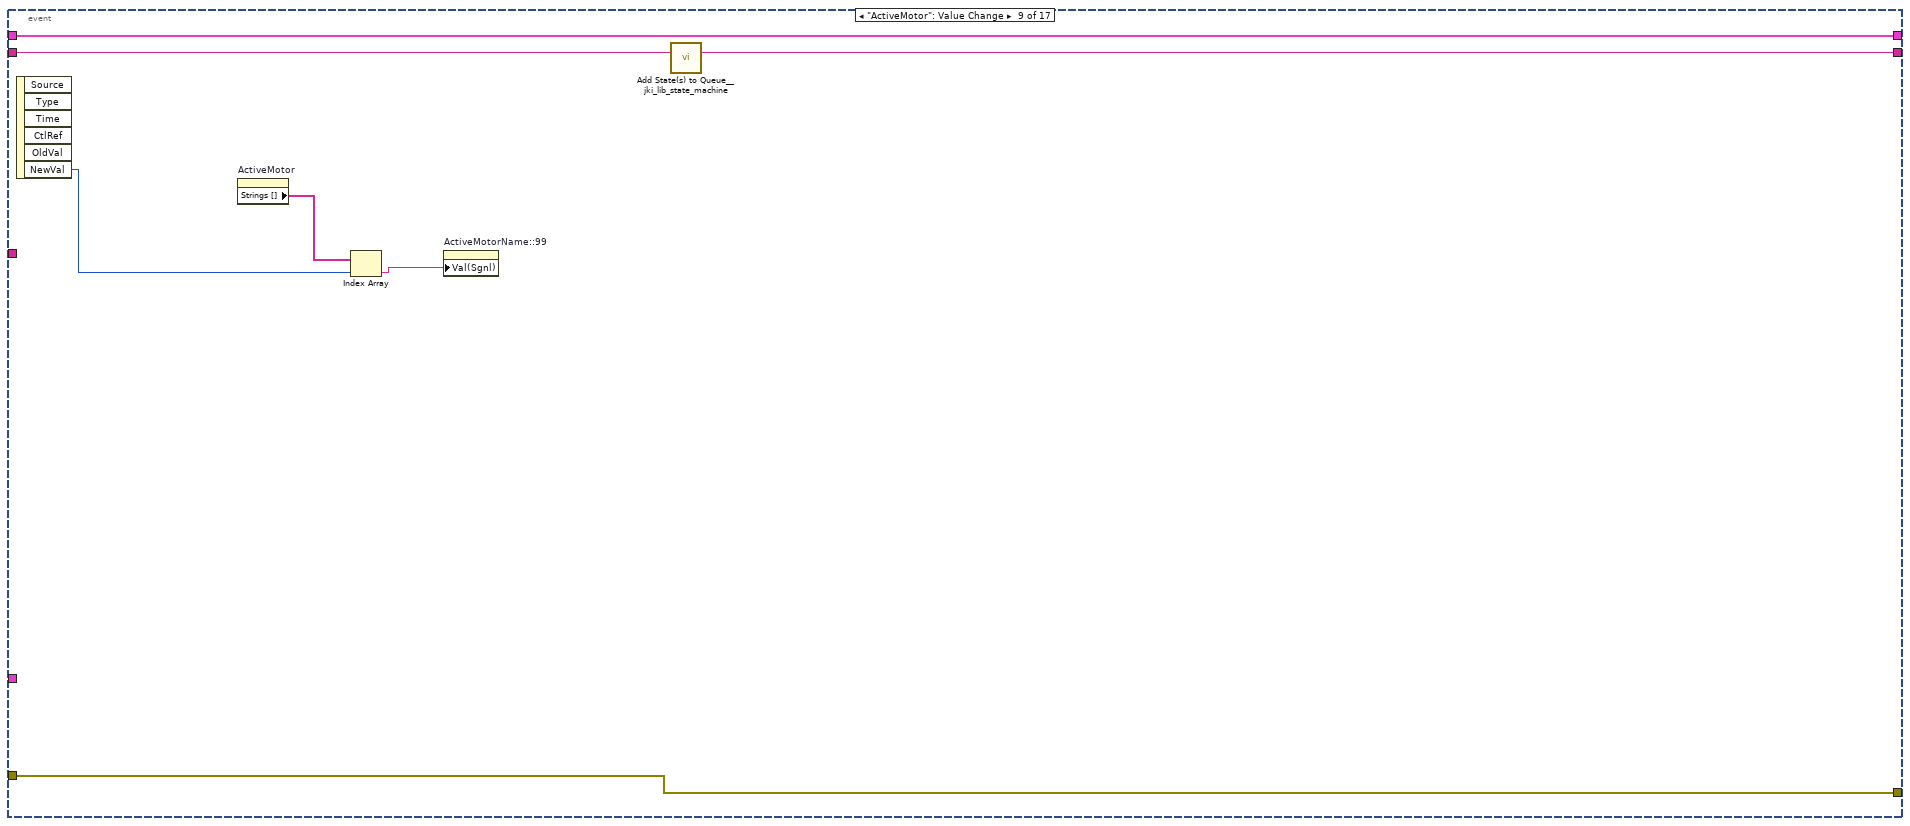
[diagram p19: hidden frame]
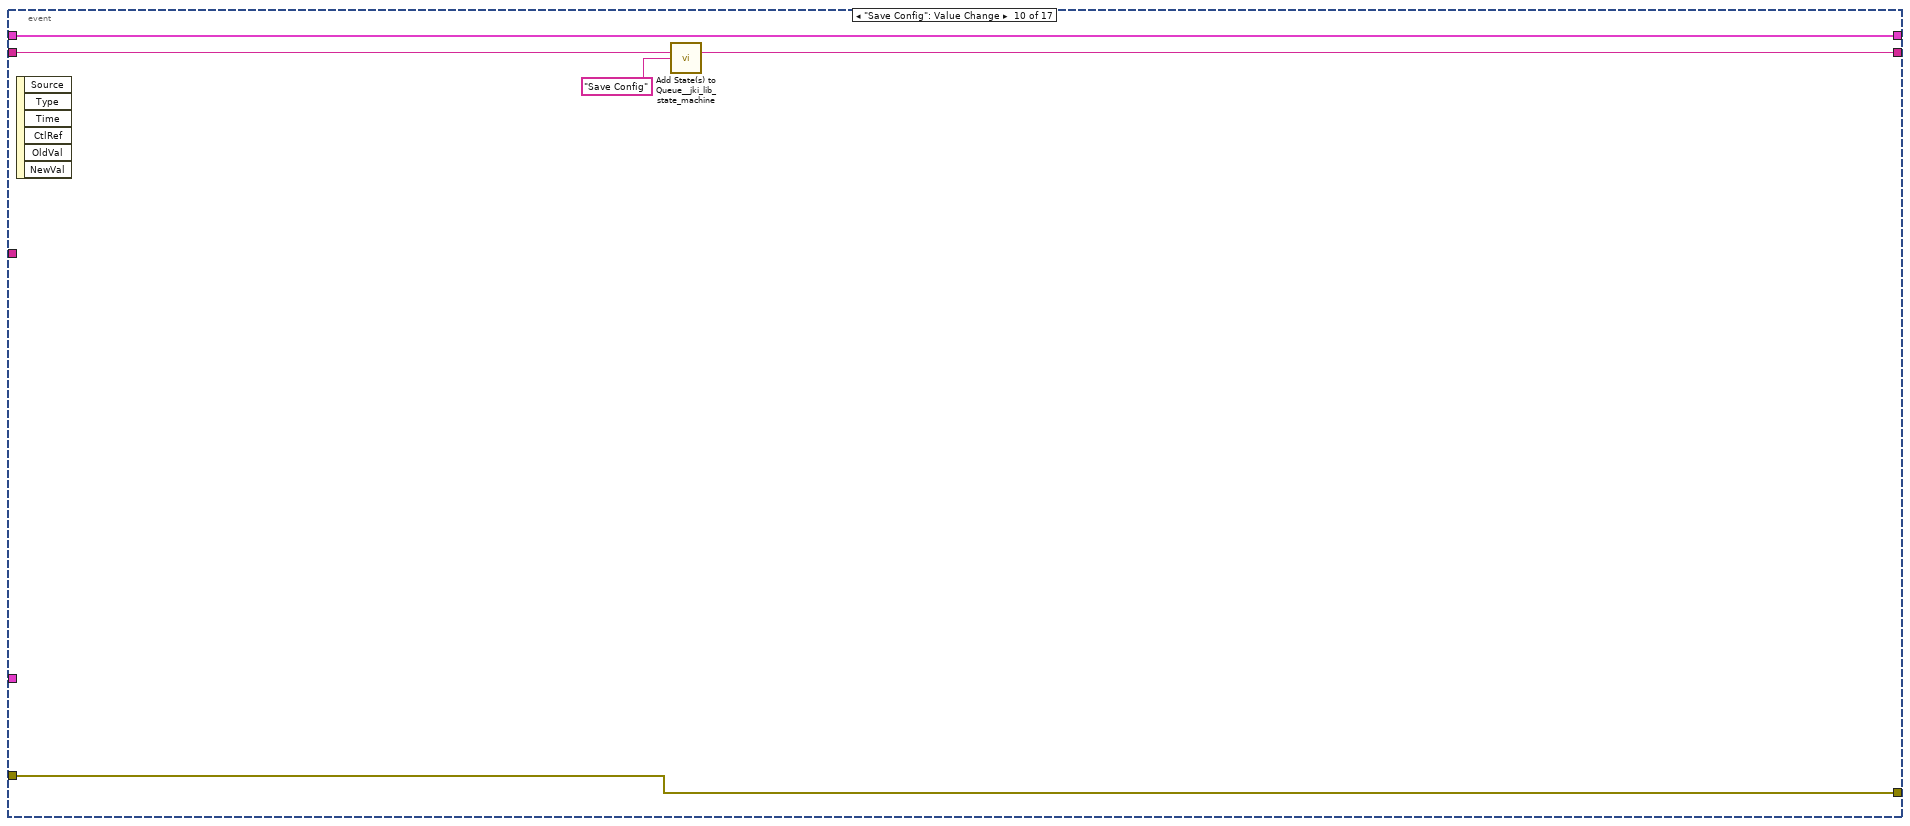
[diagram p20: hidden frame]
diagram:
  n1 = stacked-sequence {
    frame #0 {
      n2 = call <vilib>:"Application Directory.vi"() -> ("Application Directory"=w13:path)
      n3 = Build Path(base path=w13, name or relative path="defaultDevices_UPSTAIRS.txt") -> (appended path=w15:path)
      "appended path" <- w15
      n4 = call-poly <vilib>:"Read From Spreadsheet File.vi"("file path (dialog if empty)"=w15) -> ("all rows"=w16:string[][])  [unwired: 6 in, 4 out]
      n5 = Index Array(array=w16, index (col) #1=0 ("disabled index (col)"), index (col) #2=1 ("index (col)")) -> (element #1=w19:string[])  [unwired: 2 in, 1 out]
      n6 = Index Array(array=w19, index #1=0 ("index"), index #2=1 ("index"), index #3=2 ("index"), index #4=3 ("index"), index #5=4 ("index"), index #6=5 ("index"), index #7=6 ("index"), index #8=7 ("index"), index #9=8 ("index"), index #10=9 ("index"), index #11=10 ("index"), index #12=11 ("index")) -> (element #1=w12:string, element #2=w11:string, element #3=w10:string, element #4=w9:string, element #5=w8:string, element #6=w7:string, element #7=w6:string, element #8=w5:string, element #9=w4:string, element #10=w3:string, element #11=w2:string, element #12=w1:string)
      n7 = property on="GUIdevice 1" class="Str"("Val(Sgnl)"=w12) -> ()  [unwired: 2 in, 2 out]
      n8 = property on="GUIdevice 2" class="Str"("Val(Sgnl)"=w11) -> ()  [unwired: 2 in, 2 out]
      n9 = property on="GUIdevice 3" class="Str"("Val(Sgnl)"=w10) -> ()  [unwired: 2 in, 2 out]
      n10 = property on="GUIdevice 4" class="Str"("Val(Sgnl)"=w9) -> ()  [unwired: 2 in, 2 out]
      n11 = property on="GUIdevice 5" class="Str"("Val(Sgnl)"=w8) -> ()  [unwired: 2 in, 2 out]
      n12 = property on="GUIdevice 6" class="Str"("Val(Sgnl)"=w7) -> ()  [unwired: 2 in, 2 out]
      n13 = property on="GUIdevice 7" class="Str"("Val(Sgnl)"=w6) -> ()  [unwired: 2 in, 2 out]
      n14 = property on="GUIdevice 8" class="Str"("Val(Sgnl)"=w5) -> ()  [unwired: 2 in, 2 out]
      n15 = property on="GUIdevice 9" class="Str"("Val(Sgnl)"=w4) -> ()  [unwired: 2 in, 2 out]
      n16 = property on="GUIdevice 10" class="Str"("Val(Sgnl)"=w3) -> ()  [unwired: 2 in, 2 out]
      n17 = property on="GUIdevice 11" class="Str"("Val(Sgnl)"=w2) -> ()  [unwired: 2 in, 2 out]
      n18 = property on="GUIdevice 12" class="Str"("Val(Sgnl)"=w1) -> ()  [unwired: 2 in, 2 out]
    }
    frame #1 {
      w104 = T20 1 items=["Grayscale (U8)", "Grayscale (I16)", "Grayscale (SGL)", "Complex (CSG)", "RGB (U32)", "HSL (U32)", "RGB (U64)", "Grayscale (U16)"] ("Image Type")
      # "NOT FOR YOU MOFO"
      n19 = control-ref of="Position.Axis 111::98"() -> (w41:refnum<vi>)
      n20 = control-ref of="Position.Axis 112::98"() -> (w42:refnum<vi>)
      n21 = control-ref of="Position.Axis 113::98"() -> (w43:refnum<vi>)
      n22 = control-ref of="Position.Axis 121::98"() -> (w44:refnum<vi>)
      n23 = control-ref of="Position.Axis 122::98"() -> (w45:refnum<vi>)
      n24 = control-ref of="Position.Axis 123::98"() -> (w46:refnum<vi>)
      n25 = control-ref of="Position.Axis 131::98"() -> (w47:refnum<vi>)
      n26 = control-ref of="Position.Axis 132::98"() -> (w48:refnum<vi>)
      n27 = control-ref of="Position.Axis 133::98"() -> (w49:refnum<vi>)
      n28 = control-ref of="Position.Axis 141::98"() -> (w50:refnum<vi>)
      n29 = control-ref of="Position.Axis 142::98"() -> (w51:refnum<vi>)
      n30 = control-ref of="Position.Axis 143::98"() -> (w52:refnum<vi>)
      n31 = control-ref of="Position.Axis 211::98"() -> (w53:refnum<vi>)
      n32 = control-ref of="Position.Axis 212::98"() -> (w54:refnum<vi>)
      n33 = control-ref of="Position.Axis 213::98"() -> (w55:refnum<vi>)
      n34 = control-ref of="Position.Axis 221::98"() -> (w56:refnum<vi>)
      n35 = control-ref of="Position.Axis 222::98"() -> (w57:refnum<vi>)
      n36 = control-ref of="Position.Axis 223::98"() -> (w58:refnum<vi>)
      n37 = control-ref of="Position.Axis 231::98"() -> (w59:refnum<vi>)
      n38 = control-ref of="Position.Axis 232::98"() -> (w60:refnum<vi>)
      n39 = control-ref of="Position.Axis 233::98"() -> (w61:refnum<vi>)
      n40 = control-ref of="Position.Axis 241::98"() -> (w62:refnum<vi>)
      n41 = control-ref of="Position.Axis 242::98"() -> (w63:refnum<vi>)
      n42 = control-ref of="Position.Axis 243::98"() -> (w64:refnum<vi>)
      n43 = control-ref of="Position.Axis 311::98"() -> (w65:refnum<vi>)
      n44 = control-ref of="Position.Axis 312::98"() -> (w66:refnum<vi>)
      n45 = control-ref of="Position.Axis 313::98"() -> (w67:refnum<vi>)
      n46 = control-ref of="Position.Axis 321::98"() -> (w68:refnum<vi>)
      n47 = control-ref of="Position.Axis 322::98"() -> (w69:refnum<vi>)
      n48 = control-ref of="Position.Axis 323::98"() -> (w70:refnum<vi>)
      n49 = control-ref of="Position.Axis 331::98"() -> (w71:refnum<vi>)
      n50 = control-ref of="Position.Axis 332::98"() -> (w72:refnum<vi>)
      n51 = control-ref of="Position.Axis 333::98"() -> (w73:refnum<vi>)
      n52 = control-ref of="Position.Axis 341::98"() -> (w74:refnum<vi>)
      n53 = control-ref of="Position.Axis 342::98"() -> (w75:refnum<vi>)
      n54 = control-ref of="Position.Axis 343::98"() -> (w76:refnum<vi>)
      n55 = control-ref of="Position.Axis 411::98"() -> (w77:refnum<vi>)
      n56 = control-ref of="Position.Axis 412::98"() -> (w78:refnum<vi>)
      n57 = control-ref of="Position.Axis 413::98"() -> (w79:refnum<vi>)
      n58 = control-ref of="Position.Axis 421::98"() -> (w80:refnum<vi>)
      n59 = control-ref of="Position.Axis 422::98"() -> (w81:refnum<vi>)
      n60 = control-ref of="Position.Axis 423::98"() -> (w82:refnum<vi>)
      n61 = control-ref of="Position.Axis 431::98"() -> (w83:refnum<vi>)
      n62 = control-ref of="Position.Axis 432::98"() -> (w84:refnum<vi>)
      n63 = control-ref of="Position.Axis 433::98"() -> (w85:refnum<vi>)
      n64 = control-ref of="Position.Axis 441::98"() -> (w86:refnum<vi>)
      n65 = control-ref of="Position.Axis 442::98"() -> (w87:refnum<vi>)
      n66 = control-ref of="Position.Axis 443::98"() -> (w88:refnum<vi>)
      n67 = control-ref of="Position.Axis 511::98"() -> (w89:refnum<vi>)
      n68 = control-ref of="Position.Axis 512::98"() -> (w90:refnum<vi>)
      n69 = control-ref of="Position.Axis 513::98"() -> (w91:refnum<vi>)
      n70 = control-ref of="Position.Axis 521::98"() -> (w92:refnum<vi>)
      n71 = control-ref of="Position.Axis 522::98"() -> (w93:refnum<vi>)
      n72 = control-ref of="Position.Axis 523::98"() -> (w94:refnum<vi>)
      n73 = control-ref of="Position.Axis 531::98"() -> (w95:refnum<vi>)
      n74 = control-ref of="Position.Axis 532::98"() -> (w96:refnum<vi>)
      n75 = control-ref of="Position.Axis 533::98"() -> (w97:refnum<vi>)
      n76 = control-ref of="Position.Axis 541::98"() -> (w98:refnum<vi>)
      n77 = control-ref of="Position.Axis 542::98"() -> (w99:refnum<vi>)
      n78 = control-ref of="Position.Axis 543::98"() -> (w100:refnum<vi>)
      n79 = control-ref of="Position.Axis 111::99"() -> (w232:refnum<vi>)
      n80 = control-ref of="Position.Axis 112::99"() -> (w231:refnum<vi>)
      n81 = control-ref of="Position.Axis 113::99"() -> (w230:refnum<vi>)
      n82 = control-ref of="Position.Axis 121::99"() -> (w229:refnum<vi>)
      n83 = control-ref of="Position.Axis 122::99"() -> (w228:refnum<vi>)
      n84 = control-ref of="Position.Axis 123::99"() -> (w227:refnum<vi>)
      n85 = control-ref of="Position.Axis 131::99"() -> (w226:refnum<vi>)
      n86 = control-ref of="Position.Axis 132::99"() -> (w225:refnum<vi>)
      n87 = control-ref of="Position.Axis 133::99"() -> (w224:refnum<vi>)
      n88 = control-ref of="Position.Axis 141::99"() -> (w223:refnum<vi>)
      n89 = control-ref of="Position.Axis 142::99"() -> (w222:refnum<vi>)
      n90 = control-ref of="Position.Axis 143::99"() -> (w221:refnum<vi>)
      n91 = control-ref of="Position.Axis 211::99"() -> (w220:refnum<vi>)
      n92 = control-ref of="Position.Axis 212::99"() -> (w219:refnum<vi>)
      n93 = control-ref of="Position.Axis 213::99"() -> (w218:refnum<vi>)
      n94 = control-ref of="Position.Axis 221::99"() -> (w217:refnum<vi>)
      n95 = control-ref of="Position.Axis 222::99"() -> (w216:refnum<vi>)
      n96 = control-ref of="Position.Axis 223::99"() -> (w215:refnum<vi>)
      n97 = control-ref of="Position.Axis 231::99"() -> (w214:refnum<vi>)
      n98 = control-ref of="Position.Axis 232::99"() -> (w213:refnum<vi>)
      n99 = control-ref of="Position.Axis 233::99"() -> (w212:refnum<vi>)
      n100 = control-ref of="Position.Axis 241::99"() -> (w211:refnum<vi>)
      n101 = control-ref of="Position.Axis 242::99"() -> (w210:refnum<vi>)
      n102 = control-ref of="Position.Axis 243::99"() -> (w209:refnum<vi>)
      n103 = control-ref of="Position.Axis 311::99"() -> (w208:refnum<vi>)
      n104 = control-ref of="Position.Axis 312::99"() -> (w207:refnum<vi>)
      n105 = control-ref of="Position.Axis 313::99"() -> (w206:refnum<vi>)
      n106 = control-ref of="Position.Axis 321::99"() -> (w205:refnum<vi>)
      n107 = control-ref of="Position.Axis 322::99"() -> (w204:refnum<vi>)
      n108 = control-ref of="Position.Axis 323::99"() -> (w203:refnum<vi>)
      n109 = control-ref of="Position.Axis 331::99"() -> (w202:refnum<vi>)
      n110 = control-ref of="Position.Axis 332::99"() -> (w201:refnum<vi>)
      n111 = control-ref of="Position.Axis 333::99"() -> (w200:refnum<vi>)
      n112 = control-ref of="Position.Axis 341::99"() -> (w199:refnum<vi>)
      n113 = control-ref of="Position.Axis 342::99"() -> (w198:refnum<vi>)
      n114 = control-ref of="Position.Axis 343::99"() -> (w197:refnum<vi>)
      n115 = control-ref of="Position.Axis 411::99"() -> (w196:refnum<vi>)
      n116 = control-ref of="Position.Axis 412::99"() -> (w195:refnum<vi>)
      n117 = control-ref of="Position.Axis 413::99"() -> (w194:refnum<vi>)
      n118 = control-ref of="Position.Axis 421::99"() -> (w193:refnum<vi>)
      n119 = control-ref of="Position.Axis 422::99"() -> (w192:refnum<vi>)
      n120 = control-ref of="Position.Axis 423::99"() -> (w191:refnum<vi>)
      n121 = control-ref of="Position.Axis 431::99"() -> (w190:refnum<vi>)
      n122 = control-ref of="Position.Axis 432::99"() -> (w189:refnum<vi>)
      n123 = control-ref of="Position.Axis 433::99"() -> (w188:refnum<vi>)
      n124 = control-ref of="Position.Axis 441::99"() -> (w187:refnum<vi>)
      n125 = control-ref of="Position.Axis 442::99"() -> (w186:refnum<vi>)
      n126 = control-ref of="Position.Axis 443::99"() -> (w185:refnum<vi>)
      n127 = control-ref of="Position.Axis 511::99"() -> (w184:refnum<vi>)
      n128 = control-ref of="Position.Axis 512::99"() -> (w183:refnum<vi>)
      n129 = control-ref of="Position.Axis 513::99"() -> (w182:refnum<vi>)
      n130 = control-ref of="Position.Axis 521::99"() -> (w181:refnum<vi>)
      n131 = control-ref of="Position.Axis 522::99"() -> (w180:refnum<vi>)
      n132 = control-ref of="Position.Axis 523::99"() -> (w179:refnum<vi>)
      n133 = control-ref of="Position.Axis 531::99"() -> (w178:refnum<vi>)
      n134 = control-ref of="Position.Axis 532::99"() -> (w177:refnum<vi>)
      n135 = control-ref of="Position.Axis 533::99"() -> (w176:refnum<vi>)
      n136 = control-ref of="Position.Axis 541::99"() -> (w175:refnum<vi>)
      n137 = control-ref of="Position.Axis 542::99"() -> (w174:refnum<vi>)
      n138 = control-ref of="Position.Axis 543::99"() -> (w173:refnum<vi>)
      n139 = Build Array(w41, w42, w43, w44, w45, w46, w47, w48, w49, w50, w51, w52, w53, w54, w55, w56, w57, w58, w59, w60, w61, w62, w63, w64, w65, w66, w67, w68, w69, w70, w71, w72, w73, w74, w75, w76, w77, w78, w79, w80, w81, w82, w83, w84, w85, w86, w87, w88, w89, w90, w91, w92, w93, w94, w95, w96, w97, w98, w99, w100) -> (w38:refnum<vi>[])
      n140 = Build Array(w232, w231, w230, w229, w228, w227, w226, w225, w224, w223, w222, w221, w220, w219, w218, w217, w216, w215, w214, w213, w212, w211, w210, w209, w208, w207, w206, w205, w204, w203, w202, w201, w200, w199, w198, w197, w196, w195, w194, w193, w192, w191, w190, w189, w188, w187, w186, w185, w184, w183, w182, w181, w180, w179, w178, w177, w176, w175, w174, w173) -> (w37:refnum<vi>[])
      n141 = Build Array (concatenate)(w37, w38) -> (→"motor refs":refnum<vi>[])
      n142 = call "getMotorNames.vi"("DeviceName"="GUIdevice 99") -> ("elements"=w35:string[])  [unwired: 10 in]
      n143 = call "getMotorNames.vi"("DeviceName"="GUIdevice 98") -> ("elements"=w34:string[])  [unwired: 10 in]
      n144 = Build Array (concatenate)(w35, w34) -> (w39:string[])
      "Names" <- w39
      n145 = property on="Motor CCD 1" class="Ring (strict)"("Strings []"=w39) -> ()  [unwired: 2 in, 2 out]
      n146 = property on="Motor CCD 2" class="Ring (strict)"("Strings []"=w39) -> ()  [unwired: 2 in, 2 out]
      n147 = property on="Motor CCD 3" class="Ring (strict)"("Strings []"=w39) -> ()  [unwired: 2 in, 2 out]
      n148 = property on="Motor CCD 4" class="Ring (strict)"("Strings []"=w39) -> ()  [unwired: 2 in, 2 out]
      n149 = property on="Motor CCD 5" class="Ring (strict)"("Strings []"=w39) -> ()  [unwired: 2 in, 2 out]
      n150 = property on="Motor CCD 6" class="Ring (strict)"("Strings []"=w39) -> ()  [unwired: 2 in, 2 out]
      n151 = property on="Motor CCD 7" class="Ring (strict)"("Strings []"=w39) -> ()  [unwired: 2 in, 2 out]
      n152 = property on="Motor CCD 8" class="Ring (strict)"("Strings []"=w39) -> ()  [unwired: 2 in, 2 out]
      n153 = property on="Motor CCD 9" class="Ring (strict)"("Strings []"=w39) -> ()  [unwired: 2 in, 2 out]
      n154 = property on="Motor CCD 10" class="Ring (strict)"("Strings []"=w39) -> ()  [unwired: 2 in, 2 out]
      n155 = property on="Motor CCD 11" class="Ring (strict)"("Strings []"=w39) -> ()  [unwired: 2 in, 2 out]
      n156 = property on="Motor CCD 12" class="Ring (strict)"("Strings []"=w39) -> ()  [unwired: 2 in, 2 out]
      n157 = property on="ActiveMotor" class="Ring (strict)"("Strings []"=w35) -> ()  [unwired: 2 in, 2 out]
      n158 = control-ref of="Target.X::1"() -> (w159:refnum<vi>)
      n159 = control-ref of="Target.Y::1"() -> (w158:refnum<vi>)
      n160 = control-ref of="Target.X::2"() -> (w157:refnum<vi>)
      n161 = control-ref of="Target.Y::2"() -> (w156:refnum<vi>)
      n162 = control-ref of="Target.X::3"() -> (w155:refnum<vi>)
      n163 = control-ref of="Target.Y::3"() -> (w154:refnum<vi>)
      n164 = control-ref of="Target.X::4"() -> (w153:refnum<vi>)
      n165 = control-ref of="Target.Y::4"() -> (w152:refnum<vi>)
      n166 = control-ref of="Target.X::5"() -> (w151:refnum<vi>)
      n167 = control-ref of="Target.Y::5"() -> (w150:refnum<vi>)
      n168 = control-ref of="Target.X::6"() -> (w149:refnum<vi>)
      n169 = control-ref of="Target.Y::6"() -> (w148:refnum<vi>)
      n170 = control-ref of="Target.X::7"() -> (w147:refnum<vi>)
      n171 = control-ref of="Target.Y::7"() -> (w146:refnum<vi>)
      n172 = control-ref of="Target.X::8"() -> (w145:refnum<vi>)
      n173 = control-ref of="Target.Y::8"() -> (w144:refnum<vi>)
      n174 = control-ref of="Target.X::9"() -> (w121:refnum<vi>)
      n175 = control-ref of="Target.Y::9"() -> (w120:refnum<vi>)
      n176 = control-ref of="Target.X::10"() -> (w119:refnum<vi>)
      n177 = control-ref of="Target.Y::10"() -> (w118:refnum<vi>)
      n178 = control-ref of="Target.X::11"() -> (w117:refnum<vi>)
      n179 = control-ref of="Target.Y::11"() -> (w116:refnum<vi>)
      n180 = control-ref of="Target.X::12"() -> (w115:refnum<vi>)
      n181 = control-ref of="Target.Y::12"() -> (w114:refnum<vi>)
      n182 = call "IMAQ Create"("Image Name"="GUIdevice 8", "Image Type"=w104) -> ("New Image"=→"image::8":T9)  [unwired: 3 in, 1 out]
      n183 = call "IMAQ Create"("Image Name"="GUIdevice 9", "Image Type"=w104) -> ("New Image"=→"image::9":T9)  [unwired: 3 in, 1 out]
      n184 = call "IMAQ Create"("Image Name"="GUIdevice 10", "Image Type"=w104) -> ("New Image"=→"image::10":T9)  [unwired: 3 in, 1 out]
      n185 = call "IMAQ Create"("Image Name"="GUIdevice 6", "Image Type"=w104) -> ("New Image"=→"image::6":T9)  [unwired: 3 in, 1 out]
      n186 = call "IMAQ Create"("Image Name"="GUIdevice 7", "Image Type"=w104) -> ("New Image"=→"image::7":T9)  [unwired: 3 in, 1 out]
      n187 = call "IMAQ Create"("Image Name"="GUIdevice 11", "Image Type"=w104) -> ("New Image"=→"image::11":T9)  [unwired: 3 in, 1 out]
      n188 = call "IMAQ Create"("Image Name"="GUIdevice 12", "Image Type"=w104) -> ("New Image"=→"image::12":T9)  [unwired: 3 in, 1 out]
      n189 = call "IMAQ Create"("Image Name"="GUIdevice 2") -> ("New Image"=→"image::2":T9)  [unwired: 4 in, 1 out]
      n190 = call "IMAQ Create"("Image Name"="GUIdevice 4", "Image Type"=w104) -> ("New Image"=→"image::4":T9)  [unwired: 3 in, 1 out]
      n191 = call "IMAQ Create"("Image Name"="GUIdevice 1", "Image Type"=w104) -> ("New Image"=→"image::1":T9)  [unwired: 3 in, 1 out]
      n192 = call "IMAQ Create"("Image Name"="GUIdevice 3", "Image Type"=w104) -> ("New Image"=→"image::3":T9)  [unwired: 3 in, 1 out]
      n193 = call "IMAQ Create"("Image Name"="GUIdevice 5", "Image Type"=w104) -> ("New Image"=→"image::5":T9)  [unwired: 3 in, 1 out]
      n194 = Build Array("GUIdevice 1", "GUIdevice 2", "GUIdevice 3", "GUIdevice 4", "GUIdevice 5", "GUIdevice 6", "GUIdevice 7", "GUIdevice 8", "GUIdevice 9", "GUIdevice 10", "GUIdevice 11", "GUIdevice 12") -> (w133:string[])
      "CCDs" <- w133
      n195 = property on="image::8" class="ImageControl"("Caption.Text"="GUIdevice 8") -> ()  [unwired: 2 in, 2 out]
      n196 = property on="image::10" class="ImageControl"("Caption.Text"="GUIdevice 10") -> ()  [unwired: 2 in, 2 out]
      n197 = property on="image::9" class="ImageControl"("Caption.Text"="GUIdevice 9") -> ()  [unwired: 2 in, 2 out]
      n198 = property on="image::1" class="ImageControl"("Caption.Text"="GUIdevice 1") -> ()  [unwired: 2 in, 2 out]
      n199 = property on="image::2" class="ImageControl"("Caption.Text"="GUIdevice 2") -> ()  [unwired: 2 in, 2 out]
      n200 = property on="image::3" class="ImageControl"("Caption.Text"="GUIdevice 3") -> ()  [unwired: 2 in, 2 out]
      n201 = property on="image::4" class="ImageControl"("Caption.Text"="GUIdevice 4") -> ()  [unwired: 2 in, 2 out]
      n202 = property on="image::5" class="ImageControl"("Caption.Text"="GUIdevice 5") -> ()  [unwired: 2 in, 2 out]
      n203 = property on="image::6" class="ImageControl"("Caption.Text"="GUIdevice 6") -> ()  [unwired: 2 in, 2 out]
      n204 = property on="image::7" class="ImageControl"("Caption.Text"="GUIdevice 7") -> ()  [unwired: 2 in, 2 out]
      n205 = property on="image::11" class="ImageControl"("Caption.Text"="GUIdevice 11") -> ()  [unwired: 2 in, 2 out]
      n206 = property on="image::12" class="ImageControl"("Caption.Text"="GUIdevice 12") -> ()  [unwired: 2 in, 2 out]
      n207 = Array To Cluster(array=w133) -> (cluster=→"Cameras":T21)
      n208 = Bundle("Target.X::1"=w159, "Target.Y::1"=w158) -> (w143:T22)  [unwired: 1 in]
      n209 = Bundle("Target.X::2"=w157, "Target.Y::2"=w156) -> (w142:T23)  [unwired: 1 in]
      n210 = Bundle("Target.X::3"=w155, "Target.Y::3"=w154) -> (w141:T24)  [unwired: 1 in]
      n211 = Bundle("Target.X::4"=w153, "Target.Y::4"=w152) -> (w134:T25)  [unwired: 1 in]
      n212 = Bundle("Target.X::5"=w151, "Target.Y::5"=w150) -> (w140:T26)  [unwired: 1 in]
      n213 = Bundle("Target.X::6"=w149, "Target.Y::6"=w148) -> (w139:T27)  [unwired: 1 in]
      n214 = Bundle("Target.X::7"=w147, "Target.Y::7"=w146) -> (w138:T28)  [unwired: 1 in]
      n215 = Bundle("Target.X::8"=w145, "Target.Y::8"=w144) -> (w137:T29)  [unwired: 1 in]
      n216 = Bundle("Target.X::12"=w115, "Target.Y::12"=w114) -> (w110:T30)  [unwired: 1 in]
      n217 = Bundle("Target.X::9"=w121, "Target.Y::9"=w120) -> (w113:T31)  [unwired: 1 in]
      n218 = Bundle("Target.X::10"=w119, "Target.Y::10"=w118) -> (w112:T32)  [unwired: 1 in]
      n219 = Bundle("Target.X::11"=w117, "Target.Y::11"=w116) -> (w111:T33)  [unwired: 1 in]
      n220 = property on="CCDs" class="Ring (strict)"("Strings []"=w133) -> ()  [unwired: 2 in, 2 out]
      n221 = Build Array(w143, w142, w141, w134, w140, w139, w138, w137, w113, w112, w111, w110) -> (w136:T34)
      n222 = Tick Count (ms)() -> (millisecond timer value=→"millisecond timer value":u32)
      n223 = property on="Feedback Global" class="Bool (strict)"("Value"=FALSE ("Feedback Global")) -> ()  [unwired: 2 in, 2 out]
      n224 = Get Date/Time In Seconds() -> (seconds since 1Jan1904=w123:timestamp)
      n225 = Format Date/Time String(time format string (%c)="%Y%m%d%H%M", seconds (now)=w123) -> (date/time string=w122:string)  [unwired: 1 in]
      n226 = Concatenate Strings(w122, "Beampointing_Pico.tdms" ("string")) -> (w126:string)
      n227 = String To Path(string=w126) -> (path=w125:path)
      n228 = Build Path(base path=path "w:/BP_upstairs", name or relative path=w125) -> (appended path=w128:path)
      n229 = call <vilib>:"Add State(s) to Queue__jki_lib_state_machine.vi"("State(s) in (\"\")"="Macro: Initialize") -> ("States Out"=w234:string)  [unwired: 14 in]
      n230 = Create User Event(user event datatype=T14 {"EventEnum"=enum."new data", "Device name"="Device name"} ("New Event")) -> (user event=w242:refnum<user-event>, error out=w244:errorcluster)  [unwired: 1 in]
      "tcp data event" <- w242
      n231 = while "JKI - String-Based Queued State Machine (Basic) v1.0" {
        shift-right: [w266] -> w132
        shift-left: _ -> [w254]
        shift-right: [w269] -> w160
        shift-left: _ -> [w265]
        shift-right: [w268] -> _
        shift-left: w234 -> [w270]
        tunnel: w136 -> [w263]
        tunnel: w133 -> [w261]
        tunnel: [w261] -> w161
        tunnel: w136 -> [w262]
        tunnel: w128 -> [w252]
        stop <- w267 stop-if-true
        n232 = Unbundle By Name(w254) -> ("active cams"=w253:string[])
        n233 = call <vilib>:"Parse State Queue__jki_lib_state_machine.vi"("State Queue"=w270, "Error In (no error)"=w265) -> ("Remaining States"=w272:string, "Current State"=w273:string, "Arguments"=w271:string)  [unwired: 11 in]
        "Current State" <- w273
        n234 = case shown="\"Check Move\"" w273 {
          selector: w273 -> [_ _ w558 _ _ _ _ _ _ _ _ _ _ _ _ _ _ _ _ _ _ _ _ _ _ _ _ _ _ _ _ _ _ _ _ _ _ _ _]
          tunnel: w272 -> [w301 w557 w562 w580 w586 w591 w595 w633 w641 w645 w649 w655 w666 w690 w695 w705 w709 w727 w829 w868 w881 w890 w915 w936 w940 w950 w1088 w1234 w1325 w1391 w1429 w1449 w1464 w1538 w1590 w1600 w1623 w1643 w1670]
          tunnel: w271 -> [_ _ _ _ _ _ _ _ _ _ _ w650 w661 _ _ _ _ w722 _ _ w878 _ _ _ _ w952 _ w1211 w1302 _ _ _ _ _ _ _ _ _ _]
          tunnel: w254 -> [w299 w554 w560 w570 w583 w589 w592 _ w637 w642 w647 w653 w660 w687 w692 w697 w706 w719 w810 w866 w873 w886 w907 w929 w937 w968 w1082 w1227 w1318 w1388 w1400 w1446 w1461 w1536 w1587 w1597 w1609 w1640 w1661]
          tunnel: [w298 w555 w564 w578 errorcluster {"status"=FALSE, "code"=0, "source"=""} ("error out") w588 w593 w599 w634 w643 w646 w651 w663 w688 w693 w703 w707 w723 w774 w857 w879 w888 w913 w934 w938 w954 w1112 w1232 w1323 w1389 w1427 w1447 w1462 w1526 w1588 w1598 w1601 w1641 w1668] -> w269
          tunnel: w265 -> [w297 w555 w563 w578 w582 w588 w593 w606 w639 w643 w646 w652 w664 w688 w693 w703 w707 w723 w773 w858 w879 w888 w913 w934 w938 w954 w1112 w1232 w1323 w1389 w1427 w1447 w1462 w1531 w1588 w1598 w1607 w1641 w1668]
          tunnel: [w300 w556 w561 w579 w585 w590 w594 w632 w640 w644 w648 w654 w665 w689 w694 w704 w708 w710 w828 w867 w880 w889 w914 w935 w939 w957 w1113 w1233 w1324 w1390 w1428 w1448 w1463 w1537 w1589 w1599 w1622 w1642 w1669] -> w268
          tunnel: [_ _ _ _ _ TRUE _ _ _ _ _ _ _ _ _ _ _ _ _ _ _ _ _ _ _ _ _ _ _ _ _ _ _ _ _ _ _ _ _] -> w267
          tunnel: [w294 w554 w560 w569 w583 w589 w592 w627 w637 w642 w647 w653 w660 w687 w692 w697 w706 w724 w809 w866 w872 w885 w906 w928 w937 w982 w1081 w1227 w1318 w1387 w1400 w1446 w1461 w1536 w1586 w1597 w1610 w1640 w1660] -> w266
          tunnel: "update speed [ms]" -> [w296 _ _ _ _ _ _ _ _ _ _ _ _ _ _ _ _ _ _ _ _ _ _ _ _ _ _ _ _ _ _ _ _ _ _ _ _ _ _]
          tunnel: w263 -> [w293 _ _ _ _ _ _ _ _ _ _ _ _ _ _ _ _ _ _ _ _ _ _ _ _ w980 _ _ _ _ _ _ _ _ _ _ _ w1624 _]
          tunnel: w261 -> [w295 _ _ _ _ _ _ w597 _ _ _ _ _ _ _ _ _ w726 w808 _ w874 _ _ _ _ w943 _ w1231 w1322 _ w1401 _ w1450 w1534 _ _ w1604 _ _]
          tunnel: w252 -> [_ _ _ _ _ _ _ w604 _ _ _ _ _ _ _ _ _ _ _ _ _ _ _ _ _ _ _ _ _ _ _ _ _ _ _ _ _ _ _]
          frame "", "Idle" {
            # "executes when the state queue is empty"
            n235 = event shown="[15] \"deivice ini\": Value Change" {
              selector: _ -> [_ _ _ _ _ _ _ _ _ _ _ _ _ _ _ _ _]
              dyn-events: _ -> [_ _ _ _ _ _ _ _ _ _ _ _ _ _ _ _ _]
              timeout: w296 -> [_ _ _ _ _ _ _ _ _ _ _ _ _ _ _ _ _]
              tunnel: w301 -> [w337 w444 w459 w478 w483 w488 w493 w499 w506 w511 w516 w521 w530 w535 w541 w547 w553]
              tunnel: [w314 w443 w458 w477 w482 w487 w492 w498 w505 w510 w515 w520 w529 w534 w540 w546 w552] -> w300
              tunnel: w299 -> [w303 w441 w455 w474 w480 w485 w490 w496 w503 w508 w513 w518 w523 w532 w538 w544 w550]
              tunnel: [w307 w442 w457 w476 w481 w486 w491 w497 w504 w509 w514 w519 w528 w533 w539 w545 w551] -> w298
              tunnel: w297 -> [w310 w442 w457 w476 w481 w486 w491 w497 w504 w509 w514 w519 w528 w533 w539 w545 w551]
              tunnel: [w312 w441 w455 w473 w480 w485 w490 w496 w503 w508 w513 w518 w523 w532 w538 w544 w550] -> w294
              tunnel: w295 -> [w333 _ w451 _ _ _ _ _ _ _ _ _ _ _ _ _ _]
              tunnel: w293 -> [_ _ w453 _ _ _ _ _ _ _ _ _ _ _ _ _ _]
              event Timeout {
                n236 = event-data() -> ()  [unwired: 1 in, 1 out]
                n237 = Unbundle By Name(w303) -> ("Centroid X"=w331:dbl[][], "Centroid Y"=w344:dbl[][], "Size"=w336:dbl[][], "detection para"=w332:T3[], "active cams"=w326:string[], "thresholds"=w322:cluster{"Lower value":sgl, "Upper value":sgl}[])
                n238 = Unbundle By Name(w303) -> ("active ccd"=w302:i32)
                n239 = call <userlib>:"Tick Count (ms)__ogtk.vi"("error in (no error)"=w310) -> ("error out"=w309:errorcluster, "millisecond timer value"=→"millisecond timer 2":u32)  [unwired: 9 in]
                n240 = for {
                  tunnel: w326 -> [w382] mode=indexing
                  tunnel: [w396] -> w343 mode=indexing
                  tunnel: [w393] -> w345 mode=indexing
                  tunnel: [w399] -> w342 mode=indexing
                  tunnel: w331 -> [w379]
                  tunnel: w344 -> [w377]
                  tunnel: w336 -> [w374]
                  tunnel: [w392] -> w335 mode=indexing
                  tunnel: w333 -> [w389]
                  tunnel: w332 -> [w387]
                  tunnel: [w385] -> w306 mode=indexing
                  tunnel: [w384] -> w304 mode=indexing
                  tunnel: [w381] -> w327 mode=indexing
                  tunnel: [w372] -> w324 mode=indexing
                  tunnel: "autodetect" -> [w371]
                  tunnel: w322 -> [w370] mode=indexing
                  tunnel: w309 -> [w390]
                  tunnel: [w391] -> w334
                  i -> [w375]
                  w395 = dbl[] [] ("Array 4")
                  n241 = Index Array(array=w374, index (row)=w375) -> (element=w373:dbl[])  [unwired: 1 in]
                  n242 = Index Array(array=w377, index (row)=w375) -> (element=w376:dbl[])  [unwired: 1 in]
                  n243 = call-poly <userlib>:"Filter 1D Array__ogtk.vi"("items to filter"=w382, "array"=w389) -> ("filtered item indices"=w388:i32[])  [unwired: 4 in, 1 out]
                  n244 = Index Array(array=w379, index (row)=w375) -> (element=w378:dbl[])  [unwired: 1 in]
                  n245 = Index Array(array=w388) -> (element=w380:i32)  [unwired: 1 in]
                  n246 = Index Array(array=w387, index=w380) -> (element=w383:T3)
                  n247 = call "CENTRIOD DETECTION.vi"("Refnum in"=w382, "auto threshold"=w371, "Threshold Range In"=w370, "beam detection para"=w383, "error in (no error)"=w390) -> ("Bounding Rect"=w381:T35, "Particle Reports (Pixels)"=w384:T1, "Threshold Range Out"=w372:cluster{"Lower value":sgl, "Upper value":sgl}, "Centriod"=w404:cluster{"X":dbl, "Y":dbl}, "error out"=w391:errorcluster)  [unwired: 7 in, 3 out]
                  n248 = Unbundle By Name(w404) -> ("X"=w401:dbl, "Y"=w400:dbl)
                  n249 = Empty Array?(array=w384) -> (empty?=w386:bool)
                  n250 = Not Equal To 0?(x=w400) -> (x != 0?=w402:bool)
                  n251 = Not Equal To 0?(x=w401) -> (x != 0?=w403:bool)
                  n252 = Not(x=w386) -> (.not. x?=w385:bool)
                  n253 = And(x=w403, y=w402) -> (x .and. y?=w398:bool)
                  n254 = case shown="True" w398 {
                    tunnel: w401 -> [_ w437]
                    tunnel: w400 -> [_ w436]
                    tunnel: w378 -> [w423 w439]
                    tunnel: w376 -> [w422 w438]
                    tunnel: [w423 w435] -> w397
                    tunnel: [w422 w434] -> w394
                    tunnel: w381 -> [_ w433]
                    tunnel: w373 -> [w421 w426]
                    tunnel: [w421 w424] -> w392
                    frame False {
                    }
                    frame True {
                      n255 = Unbundle By Name(w433) -> ("Right"=w432:dbl, "Left"=w431:dbl, "Bottom"=w430:dbl, "Top"=w429:dbl)
                      n256 = Subtract(x=w432, y=w431) -> (x-y=w427:dbl)
                      n257 = Subtract(x=w430, y=w429) -> (x-y=w428:dbl)
                      n258 = Build Array (concatenate)(w439, w437) -> (w435:dbl[])
                      n259 = Multiply(x=w427, y=w428) -> (x*y=w425:dbl)
                      n260 = Build Array (concatenate)(w438, w436) -> (w434:dbl[])
                      n261 = Build Array (concatenate)(w426, w425) -> (w424:dbl[])
                    }
                  }
                  n262 = for {
                    tunnel: w397 -> [w414] mode=indexing
                    shift-right: [w413] -> w396
                    shift-left: w395 -> [w415]
                    n263 = Not Equal To 0?(x=w414) -> (x != 0?=w416:bool)
                    n264 = case shown="True" w416 {
                      tunnel: w415 -> [w417 w420]
                      tunnel: w414 -> [_ w419]
                      tunnel: [w417 w418] -> w413
                      frame False {
                      }
                      frame True {
                        n265 = Build Array (concatenate)(w420, w419) -> (w418:dbl[])
                      }
                    }
                  }
                  n266 = for {
                    tunnel: w394 -> [w406] mode=indexing
                    shift-right: [w405] -> w393
                    shift-left: w395 -> [w407]
                    n267 = Not Equal To 0?(x=w406) -> (x != 0?=w408:bool)
                    n268 = case shown="True" w408 {
                      tunnel: w407 -> [w409 w412]
                      tunnel: w406 -> [_ w411]
                      tunnel: [w409 w410] -> w405
                      frame False {
                      }
                      frame True {
                        n269 = Build Array (concatenate)(w412, w411) -> (w410:dbl[])
                      }
                    }
                  }
                  n270 = Array Size(array=w393) -> (size(s)=w399:i32)
                }
                "detected" <- w306
                "Particle Reports (Pixels)" <- w304
                "Box" <- w327
                n271 = Bundle(0, 1, "Centroid X"=w331) -> (→"Status":cluster{i32, i32, "Centroid X":dbl[][]})  [unwired: 1 in]
                n272 = Index Array(array=w304, index (row)=w302) -> (element=→"particles":T1)  [unwired: 1 in]
                n273 = call <vilib>:"Clear Errors.vi"("error in (no error)"=w334) -> ("error out"=w307:errorcluster)  [unwired: 6 in]
                n274 = local read "Img to avg"() -> (w316:i32)
                n275 = local read "Numeric"() -> (w319:dbl)
                n276 = Increment(x=w316) -> (x+1=w315:i32)
                n277 = Greater Or Equal?(x=w319, y=w315) -> (x >= y?=w311:bool)
                n278 = Increment(x=w319) -> (x+1=w318:dbl)
                n279 = Select(t=0.0, s=w311, f=w318) -> (s? t:f=w317:dbl)
                n280 = local write "Numeric"(w317) -> ()
                n281 = for {
                  tunnel: w342 -> [w362] mode=indexing
                  tunnel: w326 -> [w369] mode=indexing
                  shift-right: [w364] -> w338
                  shift-left: "" ("GUIdevice 7") -> [w367]
                  tunnel: [w357] -> w340 mode=indexing
                  tunnel: "Detection Rate" -> [w361]
                  tunnel: w317 -> [w359]
                  n282 = local read "Img to avg"() -> (w363:i32)
                  n283 = Greater Or Equal?(x=w362, y=w363) -> (x >= y?=w358:bool)
                  n284 = Multiply(x=w361, y=w359) -> (x*y=w360:dbl)
                  n285 = Greater Or Equal?(x=w362, y=w360) -> (x >= y?=w356:bool)
                  n286 = And(x=w358, y=w356) -> (x .and. y?=w357:bool)
                  n287 = Select(t=w369, s=w357, f="") -> (s? t:f=w365:string)
                  n288 = Concatenate Strings(w367, "\t", w365) -> (w364:string)
                }
                n289 = Bundle By Name(cluster=w303, "thresholds"=w324, "detected"=w306) -> (w323:T36)
                n290 = Bundle By Name(cluster=w323, "Centroid X"=w343, "Centroid Y"=w345, "Size"=w335) -> (w313:T36)
                n291 = Or Array Elements(Boolean array=w340) -> (logical OR=w339:bool)
                n292 = case shown="True" w311 {
                  tunnel: w313 -> [w346 w349]
                  tunnel: [w346 w348] -> w312
                  frame False {
                  }
                  frame True {
                    n293 = local read "Centroid X"() -> (w347:dbl[][])
                    n294 = Bundle By Name(cluster=w349, "Centroid X"=w347, "Centroid Y"=w347, "Size"=w347) -> (w348:T36)
                  }
                }
                n295 = case shown="True" w339 {
                  tunnel: w338 -> [_ w354]
                  tunnel: w337 -> [w350 w352]
                  tunnel: [w350 w351] -> w314
                  frame False {
                  }
                  frame True {
                    n296 = call <vilib>:"Build State String with Arguments__jki_lib_state_machine.vi"("Arguments (\"\")"=w354, "State"="detected") -> ("State with Arguments"=w353:string)  [unwired: 4 in]
                    n297 = call <vilib>:"Add State(s) to Queue__jki_lib_state_machine.vi"("State(s) in (\"\")"=w352, "State(s) at Back (\"\")"=w353) -> ("States Out"=w351:string)  [unwired: 13 in]
                  }
                }
              }
              event "stop": Value Change {
                # "Exit Button Value Change (pressed) Event\n(this executes Macro: Exit to terminate the VI)"
                n298 = event-data() -> ()  [unwired: 1 in, 6 out]
                n299 = call <vilib>:"Add State(s) to Queue__jki_lib_state_machine.vi"("State(s) in Front (\"\")"="Macro: Exit", "State(s) in (\"\")"=w444) -> ("States Out"=w443:string)  [unwired: 13 in]
              }
              event Value Change {
                n300 = event-data() -> ()  [unwired: 1 in, 6 out]
                n301 = property on="Set Centriod Target" class="Bool (strict)"("Value"=FALSE) -> ()  [unwired: 2 in, 2 out]
                n302 = Unbundle By Name(w455) -> ("active ccd"=w447:i32, "Centroid X"=w446:dbl[][], "Centroid Y"=w445:dbl[][])
                n303 = Index Array(array=w451, index=w447) -> (element=w450:string)
                n304 = Concatenate Strings("Do want to update the target of " ("message"), w450, "?" ("string")) -> (w448:string)
                n305 = Two Button Dialog(message=w448) -> (T button?=w454:bool)  [unwired: 2 in]
                n306 = case shown="True" w454 {
                  tunnel: w453 -> [_ w466]
                  tunnel: w447 -> [_ w465]
                  tunnel: w446 -> [_ w472]
                  tunnel: w445 -> [_ w467]
                  frame False {
                  }
                  frame True {
                    n307 = Index Array(array=w472, index (row)=w465) -> (element=w471:dbl[])  [unwired: 1 in]
                    n308 = Index Array(array=w467, index (row)=w465) -> (element=w468:dbl[])  [unwired: 1 in]
                    n309 = Index Array(array=w466, index=w465) -> (element=w464:T30)
                    n310 = Unbundle By Name(w464) -> ("Target.X::12"=w463:refnum<vi>, "Target.Y::12"=w461:refnum<vi>)
                    n311 = Reverse 1D Array(array=w471) -> (reversed array=w470:dbl[])
                    n312 = Reverse 1D Array(array=w468) -> (reversed array=w469:dbl[])
                    n313 = Index Array(array=w470) -> (element=w462:dbl)  [unwired: 1 in]
                    n314 = Index Array(array=w469) -> (element=w460:dbl)  [unwired: 1 in]
                    n315 = property class="DigNum (strict)"(reference=w463, "Val(Sgnl)"=w462) -> ()  [unwired: 1 in, 2 out]
                    n316 = property class="DigNum (strict)"(reference=w461, "Val(Sgnl)"=w460) -> ()  [unwired: 1 in, 2 out]
                  }
                }
                n317 = call <vilib>:"Add State(s) to Queue__jki_lib_state_machine.vi"("State(s) in (\"\")"=w459) -> ("States Out"=w458:string)  [unwired: 14 in]
              }
              event "Feedback Global": Value Change {
                # "Exit Button Value Change (pressed) Event\n(this executes Macro: Exit to terminate the VI)"
                n318 = event-data() -> ("NewVal"=w475:bool)  [unwired: 1 in, 5 out]
                n319 = call <vilib>:"Add State(s) to Queue__jki_lib_state_machine.vi"("State(s) in (\"\")"=w478) -> ("States Out"=w477:string)  [unwired: 14 in]
                n320 = Bundle By Name(cluster=w474, "Feedback global"=w475) -> (w473:T36)
              }
              event Value Change {
                n321 = event-data() -> ()  [unwired: 1 in, 6 out]
                n322 = call <vilib>:"Add State(s) to Queue__jki_lib_state_machine.vi"("State(s) in Front (\"\")"="Move Config", "State(s) in (\"\")"=w483) -> ("States Out"=w482:string)  [unwired: 13 in]
              }
              event Value Change {
                n323 = event-data() -> ()  [unwired: 1 in, 6 out]
                n324 = call <vilib>:"Add State(s) to Queue__jki_lib_state_machine.vi"("State(s) in Front (\"\")"="Detection Config", "State(s) in (\"\")"=w488) -> ("States Out"=w487:string)  [unwired: 13 in]
              }
              event "associated motors": Value Change {
                n325 = event-data() -> ()  [unwired: 1 in, 6 out]
                n326 = call <vilib>:"Add State(s) to Queue__jki_lib_state_machine.vi"("State(s) in (\"\")"=w493, "State(s) at Back (\"\")"="Motor Config" ("State(s) at Back (\"\")")) -> ("States Out"=w492:string)  [unwired: 13 in]
              }
              event "Reset History": Value Change {
                n327 = event-data() -> ()  [unwired: 1 in, 6 out]
                n328 = call <vilib>:"Add State(s) to Queue__jki_lib_state_machine.vi"("State(s) in (\"\")"=w499, "State(s) at Back (\"\")"="Reset History" ("State(s) at Back (\"\")")) -> ("States Out"=w498:string)  [unwired: 13 in]
                n329 = property on="Reset History" class="Bool (strict)"("Value"=FALSE ("Reset History")) -> ()  [unwired: 2 in, 2 out]
              }
              event "ActiveMotor": Value Change {
                n330 = event-data() -> ("NewVal"=w501:u16)  [unwired: 1 in, 5 out]
                n331 = property on="ActiveMotor" class="Ring (strict)"() -> ("Strings []"=w502:string[])  [unwired: 2 in, 2 out]
                n332 = Index Array(array=w502, index=w501) -> (element=w500:string)
                n333 = property on="ActiveMotorName::99" class="Str"("Val(Sgnl)"=w500) -> ()  [unwired: 2 in, 2 out]
                n334 = call <vilib>:"Add State(s) to Queue__jki_lib_state_machine.vi"("State(s) in (\"\")"=w506) -> ("States Out"=w505:string)  [unwired: 14 in]
              }
              event "Save Config": Value Change {
                n335 = event-data() -> ()  [unwired: 1 in, 6 out]
                n336 = call <vilib>:"Add State(s) to Queue__jki_lib_state_machine.vi"("State(s) in (\"\")"=w511, "State(s) at Back (\"\")"="Save Config" ("State(s) at Back (\"\")")) -> ("States Out"=w510:string)  [unwired: 13 in]
              }
              event "Load Config": Value Change {
                n337 = event-data() -> ()  [unwired: 1 in, 6 out]
                n338 = call <vilib>:"Add State(s) to Queue__jki_lib_state_machine.vi"("State(s) in (\"\")"=w516, "State(s) at Back (\"\")"="Load Config" ("State(s) at Back (\"\")")) -> ("States Out"=w515:string)  [unwired: 13 in]
              }
              event "Save Stats": Value Change {
                n339 = event-data() -> ()  [unwired: 1 in, 6 out]
                n340 = call <vilib>:"Add State(s) to Queue__jki_lib_state_machine.vi"("State(s) in (\"\")"=w521, "State(s) at Back (\"\")"="Save Stats" ("State(s) at Back (\"\")")) -> ("States Out"=w520:string)  [unwired: 13 in]
              }
              event "active CCDs": Value Change {
                n341 = event-data() -> ("NewVal"=w527:i32)  [unwired: 1 in, 5 out]
                n342 = Unbundle By Name(w523) -> ("active cams"=w522:string[])
                n343 = Index Array(array=w522, index=w527) -> (element=w525:string)
                n344 = call <vilib>:"Build State String with Arguments__jki_lib_state_machine.vi"("Arguments (\"\")"=w525, "State"="active" ("State(s) at Back (\"\")")) -> ("State with Arguments"=w524:string)  [unwired: 4 in]
                n345 = call <vilib>:"Add State(s) to Queue__jki_lib_state_machine.vi"("State(s) in (\"\")"=w530, "State(s) at Back (\"\")"=w524) -> ("States Out"=w529:string)  [unwired: 13 in]
              }
              event "Center": Value Change {
                n346 = event-data() -> ()  [unwired: 1 in, 6 out]
                n347 = call <vilib>:"Add State(s) to Queue__jki_lib_state_machine.vi"("State(s) in (\"\")"=w535, "State(s) at Back (\"\")"="Center" ("State(s) at Back (\"\")")) -> ("States Out"=w534:string)  [unwired: 13 in]
              }
              event "new tdms": Value Change {
                n348 = event-data() -> ()  [unwired: 1 in, 6 out]
                n349 = property on="new tdms" class="Bool (strict)"("Value"=FALSE ("new tdms")) -> ()  [unwired: 2 in, 2 out]
                n350 = call <vilib>:"Add State(s) to Queue__jki_lib_state_machine.vi"("State(s) in (\"\")"=w541, "State(s) at Back (\"\")"="newtdms" ("State(s) at Back (\"\")")) -> ("States Out"=w540:string)  [unwired: 13 in]
              }
              event "deivice ini": Value Change {
                n351 = event-data() -> ()  [unwired: 1 in, 6 out]
                n352 = property on="deivice ini" class="Bool (strict)"("Value"=FALSE ("new tdms")) -> ()  [unwired: 2 in, 2 out]
                n353 = call <vilib>:"Add State(s) to Queue__jki_lib_state_machine.vi"("State(s) in (\"\")"=w547, "State(s) at Back (\"\")"="Device Ini" ("State(s) at Back (\"\")")) -> ("States Out"=w546:string)  [unwired: 13 in]
              }
              event Panel Close? {
                # "Discard the event because we'll close the front panel ourselves in Macro: Exit"
                # "Close Panel button (pressed) Event\n(this executes Macro: Exit to terminate the VI)"
                n354 = event-data() -> ()  [unwired: 1 in, 1 out]
                n355 = call <vilib>:"Add State(s) to Queue__jki_lib_state_machine.vi"("State(s) in Front (\"\")"="Macro: Exit", "State(s) in (\"\")"=w553) -> ("States Out"=w552:string)  [unwired: 13 in]
                n356 = event-data("Discard?"=TRUE) -> ()  [unwired: 1 in, 1 out]
              }
            }
          }
          frame "---------- Core ----------" {
            # "Do not put any code in this frame.\n(it is a separator no-op)"
            n357 = call <vilib>:"Add State(s) to Queue__jki_lib_state_machine.vi"("State(s) in (\"\")"=w557) -> ("States Out"=w556:string)  [unwired: 14 in]
          }
          frame Default {
            w567 = 42 items=["No error", "Argument error", "Memory is full", "Out of zone", "End of file", "File already open", "Generic file I/O error", "File not found", "File permission error", "Disk is full", "Duplicate path", "Too many files open", "System feature not enabled", "Resource file not found", "Cannot add resource", "Resource not found", "Image not found", "Image memory error", "Pen does not exist", "Config type invalid", "Config token not found", "Config parse error", "Config memory error", "Bad external code format", "Bad external code offset", "External code not present", "Null window", "Destroy window error", "Null menu", "Print aborted", "Bad print record", "Print driver error", "Windows error during printing", "Memory error during printing", "Print dialog error", "Generic print error", "Invalid device refnum", "Device not found", "Device parameter error", "Device unit error", "Cannot open device", "Device call aborted", "Generic error", "Cancelled by user", "Object ID too low", "Object ID too high", "Object not in heap", "Unknown heap", "Unknown object (invalid DefProc)", "Unknown object (DefProc not in table)", "Message out of range", "Invalid (null) method", "Unknown message", "Manager call not supported", "Bad address", "Network operation in progress", "Network operation timed out", "Connection is busy", "Network attribute not supported", "Network error", "Address in use", "System out of memory", "Connection aborted", "Connection refused", "Not connected", "Already connected", "Connection closed", "Initialization error (interapplication manager)", "Bad occurrence", "Wait on unbound occurrence handler", "Occurrence queue overflow", "Datalog type conflict", "Unused", "Unrecognized type (interapplication manager)", "Memory corrupt", "Failed to make temporary DLL", "Old CIN version", "Drag socket not found", "Failed to load drop-object", "Failed to register OLE object", "Failed to release OLE object", "Format specifier type mismatch", "Unknown format specifier", "Too few format specifiers", "Too many format specifiers", "Scan failed", "Newer CIN version", "Error converting to variant", "Runtime menu error", "Password tampered", "Variant attribute not found", "Incompatible variant data type", "Event data is not available", "Event Store is not present", "Occurrence is not found", "Event Queue is not created", "Event info is not available", "Refnum passed is NULL", "Error retrieving Class GUID", "Error retrieving CoClass GUID", "Error retrieving TypeLib GUID.", "Bad built application magic bytes.", "Specific driver is different from the specific driver associated with the Logical Name.", "There is no session opened to the class driver.", "Max Error", "MAX - Error with config objects", "MAX - Error loading configuration", "MAX - Group not supported"]
            # "Current State"
            # "Do not delete, rename, or modify this frame.\n(this is used to capture unhandled states and typos)"
            # "Handle mistyped state name (developer tool)"
            n358 = Format Into String(format string="Software Exception: Unhandled State \"%s\"." ("message"), error in=w563, w558) -> (resulting string=w566:string, error out=w565:errorcluster)  [unwired: 1 in]
            n359 = call <vilib>:"Error Cluster From Error Code.vi"("show call chain? (False)"=TRUE, "error in (no error)"=w565, "error message (\"\")"=w566, "error code (0)"=w567) -> ("error out"=w564:errorcluster)  [unwired: 5 in]
            n360 = call <vilib>:"Add State(s) to Queue__jki_lib_state_machine.vi"("State(s) in (\"\")"=w562) -> ("States Out"=w561:string)  [unwired: 14 in]
          }
          frame "Initialize Core Data" {
            # "Do not delete, rename, or modify this frame.\n(this is used to determine panel behavior on exit)"
            # "originally closed?"
            # "exe?"
            # "If panel starts closed or is an EXE, then close it when we exit"
            n361 = property class="VI"() -> ("Front Panel.Open"=w577:bool)  [unwired: 2 in, 2 out]
            n362 = property class="App"() -> ("App.Kind"=w576:T16)  [unwired: 2 in, 2 out]
            n363 = control-ref of="Current VI Reference"() -> (w571:refnum<vi>)
            n364 = Not(x=w577) -> (.not. x?=w574:bool)
            n365 = Equal?(x=w576, y=T16."Run Time System" ("Application:Kind")) -> (x = y?=w573:bool)
            n366 = Or(x=w574, y=w573) -> (x .or. y?=w572:bool)
            n367 = Bundle By Name(cluster=w570, "Core.Current VI Reference"=w571, "Core.Close Panel on Exit?"=w572) -> (w569:T36)
            n368 = call <vilib>:"Add State(s) to Queue__jki_lib_state_machine.vi"("State(s) in (\"\")"=w580) -> ("States Out"=w579:string)  [unwired: 14 in]
          }
          frame "Error Handler" {
            # "Unhandled Error -- Display it"
            # "Handle any errors here.\nYou can also output any states to clean-up after errors occur"
            # "Clear error"
            n369 = call <vilib>:"General Error Handler.vi"("error in (no error)"=w582) -> ()  [unwired: 10 in, 5 out]
            n370 = call <vilib>:"Add State(s) to Queue__jki_lib_state_machine.vi"("State(s) in Front (\"\")"="/* Post Error States", "State(s) in (\"\")"=w586) -> ("States Out"=w585:string)  [unwired: 13 in]
          }
          frame "Exit" {
            # "Do not put any code in this frame.\n(No errors that occur here will be handled.)"
            n371 = call <vilib>:"Add State(s) to Queue__jki_lib_state_machine.vi"("State(s) in (\"\")"=w591) -> ("States Out"=w590:string)  [unwired: 14 in]
          }
          frame "---------- Data ----------" {
            # "Do not put any code in this frame.\n(It is a separator no-op. You can make a copy of this frame to create a new Data frame)"
            n372 = call <vilib>:"Add State(s) to Queue__jki_lib_state_machine.vi"("State(s) in (\"\")"=w595) -> ("States Out"=w594:string)  [unwired: 14 in]
          }
          frame "Data: Initialize" {
            w601 = bool[] [FALSE, FALSE, FALSE, FALSE, FALSE, FALSE, FALSE, FALSE, FALSE, FALSE, FALSE, TRUE]  # speedmode Y
            w602 = bool[] [FALSE, FALSE, FALSE, FALSE, FALSE, FALSE, FALSE, FALSE, FALSE, FALSE, FALSE, TRUE]  # speedmode X
            w603 = bool[] [FALSE, FALSE, FALSE, FALSE, TRUE, TRUE, TRUE, FALSE, FALSE, FALSE, FALSE, FALSE]  # detected
            w605 = cluster{"Lower value":sgl, "Upper value":sgl}[] [{"Lower value"=93.0, "Upper value"=255.0}, {"Lower value"=105.0, "Upper value"=255.0}, {"Lower value"=0.0, "Upper value"=255.0}, {"Lower value"=127.0, "Upper value"=255.0}, {"Lower value"=0.0, "Upper value"=255.0}, {"Lower value"=0.0, "Upper value"=255.0}, {"Lower value"=0.0, "Upper value"=255.0}, {"Lower value"=0.0, "Upper value"=255.0}, {"Lower value"=0.0, "Upper value"=255.0}, {"Lower value"=0.0, "Upper value"=255.0}, {"Lower value"=0.0, "Upper value"=255.0}, {"Lower value"=0.0, "Upper value"=255.0}]  # thresholds
            w616 = FALSE  # Feedback global
            w618 = 0  # active ccd
            w630 = 20  # img to avg
            w631 = T37 {"Current VI Reference"=refnum, "Close Panel on Exit?"=FALSE}  # Core
            # "Initialize the shift-register data, here.\n(data names are defined by what you wire into the bundle function)"
            n373 = TDMS Open(6:FALSE ("disable buffering (T)"), 7:enum16{"1.0", "2.0"}."2.0" ("file format version (2.0)"), 8:w606, 10:T17."create or replace" ("operation"), 11:w604) -> (0:w600:errorcluster, 3:w598:refnum<k34>)  [unwired: 1 in]
            n374 = call "TDMSbuffersize.vi"("error in (no error)"=w600, "group names"=w597, "Data Value Reference in"=w598) -> ("error out"=w599:errorcluster, "Data Value Reference out"=w596:refnum<k34>)  [unwired: 7 in]
            n375 = call <vilib>:"Add State(s) to Queue__jki_lib_state_machine.vi"("State(s) in (\"\")"=w633) -> ("States Out"=w632:string)  [unwired: 14 in]
            n376 = Bundle("Core"=w631, "detection para"="detection para", "thresholds"=w605, "Centroid X"="Centroid X", "Centroid Y"="Centroid Y", "img to avg"=w630, "Mean Centroid X"="Mean Centroid X", "Mean Centroid Y"="Mean Centroid Y", "Offset X"="Offset X", "Offset Y"="Offset Y", "Offset X stats"="Offset X stats", "Offset Y stats"="Offset Y stats", "Size"="Size", "Mean Size"="Mean Size", "Time"="Time", "move properties"="move properties", "active axis refs 2"="active axis refs 2", "active ccd"=w618, "Feedback global"=w616, "Motor X"="Motor X", "Motor Y"="Motor Y", "active cams"="active cams", "Data Value Reference out"=w596, "detected"=w603, "speedmode X"=w602, "speedmode Y"=w601) -> (w627:T36)  [unwired: 1 in]
          }
          frame "Data: Cleanup" {
            # "Cleanup any data and references, here.\n(this is called automatically, by the Macro: Exit)"
            n377 = Unbundle By Name(w637) -> ("Core.Current VI Reference"=w638:refnum<vi>)
            n378 = Close Reference(reference=w638, error in (no error)=w639) -> (error out=w635:errorcluster)
            n379 = Unbundle By Name(w637) -> ("Data Value Reference out"=w636:refnum<k34>)
            n380 = TDMS Close(8:w635, 11:w636) -> (0:w634:errorcluster)  [unwired: 1 out]
            n381 = call <vilib>:"Add State(s) to Queue__jki_lib_state_machine.vi"("State(s) in (\"\")"=w641) -> ("States Out"=w640:string)  [unwired: 14 in]
          }
          frame "---------- UI ----------" {
            # "Do not put any code in this frame.\n(It is a separator no-op. You can make a copy of this frame to create a new UI frame)"
            n382 = call <vilib>:"Add State(s) to Queue__jki_lib_state_machine.vi"("State(s) in (\"\")"=w645) -> ("States Out"=w644:string)  [unwired: 14 in]
          }
          frame "UI: Initialize" {
            # "Initialize the User Interface, here.\n(this is called automatically, by the Macro: Init)"
            n383 = call <vilib>:"Add State(s) to Queue__jki_lib_state_machine.vi"("State(s) in (\"\")"=w649) -> ("States Out"=w648:string)  [unwired: 14 in]
          }
          frame "UI: Cursor Set" {
            # "Argument"
            # "Set and Unset Cursor Busy.\n(Usage: \"UI: Cursor Set >> Busy|Idle\")"
            n384 = case shown="\"Idle\", Default" w650 {
              tunnel: w652 -> [w657 w659]
              tunnel: [w656 w658] -> w651
              frame "Idle", Default {
                n385 = call <vilib>:"Unset Busy.vi"("error in (no error)"=w657) -> ("error out"=w656:errorcluster)  [unwired: 10 in]
              }
              frame "Busy" {
                n386 = call <vilib>:"Set Busy.vi"("error in (no error)"=w659) -> ("error out"=w658:errorcluster)  [unwired: 9 in, 1 out]
              }
            }
            n387 = call <vilib>:"Add State(s) to Queue__jki_lib_state_machine.vi"("State(s) in (\"\")"=w655) -> ("States Out"=w654:string)  [unwired: 14 in]
          }
          frame "UI: Front Panel State" {
            # "Argument"
            # "Set Front Panel Open or Closed\n(Usage: \"UI: Front Panel State >> Open|Close\")"
            n388 = Unbundle By Name(w660) -> ("Core.Current VI Reference"=w662:refnum<vi>)
            n389 = case shown="\"Open\", Default" w661 {
              tunnel: w664 -> [w670 w681]
              tunnel: [w671 w682] -> w663
              tunnel: w662 -> [_ _]
              frame "Open", Default {
                n390 = property class="VI"(error in=w670) -> (reference out=w668:refnum<vi>, error out=w669:errorcluster, "Front Panel.Open"=w667:bool)  [unwired: 1 in]
                n391 = case shown="False" w667 {
                  tunnel: [w674 w677] -> w671
                  tunnel: w669 -> [w673 w677]
                  tunnel: w668 -> [w672 _]
                  frame False {
                    n392 = invoke class="VI" method="FP.Open"(reference=w672, error in=w673, "Activate"=TRUE, "State"=T18."Standard") -> (error out=w674:errorcluster)  [unwired: 1 in, 4 out]
                  }
                  frame True {
                  }
                }
              }
              frame "Close" {
                n393 = property class="VI"(error in=w681) -> (reference out=w679:refnum<vi>, error out=w680:errorcluster, "Front Panel.Open"=w678:bool)  [unwired: 1 in]
                n394 = case shown="True" w678 {
                  tunnel: [w683 w686] -> w682
                  tunnel: w680 -> [w683 w685]
                  tunnel: w679 -> [_ w684]
                  frame False {
                  }
                  frame True {
                    n395 = invoke class="VI" method="FP.Close"(reference=w684, error in=w685) -> (error out=w686:errorcluster)  [unwired: 1 in, 2 out]
                  }
                }
              }
            }
            n396 = call <vilib>:"Add State(s) to Queue__jki_lib_state_machine.vi"("State(s) in (\"\")"=w666) -> ("States Out"=w665:string)  [unwired: 14 in]
          }
          frame "---------- Macro ----------" {
            # "Do not put any code in this frame.\n(It is a separator no-op. You can make a copy of this frame to create a new Macro frame)"
            n397 = call <vilib>:"Add State(s) to Queue__jki_lib_state_machine.vi"("State(s) in (\"\")"=w690) -> ("States Out"=w689:string)  [unwired: 14 in]
          }
          frame "Macro: Initialize" {
            w691 = "Data: Initialize\nInitialize Core Data\nUI: Initialize\nUI: Front Panel State >> Open\nDevice Ini >> 3000"  # Data: Initialize Initialize Core Data UI: Initialize UI: Front Panel State >> Open Device Ini >> 3000
            # "Initialization Macro\n(This is called once, when the VI starts)"
            n398 = call <vilib>:"Add State(s) to Queue__jki_lib_state_machine.vi"("State(s) in Front (\"\")"=w691, "State(s) in (\"\")"=w695) -> ("States Out"=w694:string)  [unwired: 13 in]
          }
          frame "Macro: Exit" {
            # "Exit Macro\n(This is called once, when the VI exits)"
            n399 = Unbundle By Name(w697) -> ("Core.Close Panel on Exit?"=w696:bool)
            n400 = Select(t="UI: Front Panel State >> Close", s=w696, f="") -> (s? t:f=w700:string)
            n401 = call <vilib>:"Add State(s) to Queue__jki_lib_state_machine.vi"("State(s) in (\"\")"=w700, "State(s) at Back (\"\")"="Data: Cleanup\nExit") -> ("States Out"=w698:string)  [unwired: 13 in]
            n402 = call <vilib>:"Add State(s) to Queue__jki_lib_state_machine.vi"("State(s) in Front (\"\")"=w698, "State(s) in (\"\")"=w705) -> ("States Out"=w704:string)  [unwired: 13 in]
          }
          frame "---------- Ini and Configure ----------" {
            # "Template Separator\n(You can make a copy of, or modify, this frame)"
            n403 = call <vilib>:"Add State(s) to Queue__jki_lib_state_machine.vi"("State(s) in (\"\")"=w709) -> ("States Out"=w708:string)  [unwired: 14 in]
          }
          frame "Device Ini" {
            # "Your code here.\n(You can make a copy of, or modify, this frame)"
            n404 = Empty String/Path?(string/path=w722) -> (empty?=w720:bool)
            n405 = case shown="False" w720 {
              tunnel: w722 -> [w751 _]
              tunnel: [w750 0] -> w721
              frame False {
                n406 = Decimal String To Number(string=w751) -> (number=w750:i32)  [unwired: 2 in, 1 out]
              }
              frame True {
              }
            }
            n407 = flat-sequence {
              tunnel: w726 -> [w754]
              tunnel: [w754] -> w725
              tunnel: w721 -> [w753]
              tunnel: w725 -> [w757]
              tunnel: [w755] -> w713
              frame #0 {
                n408 = Wait (ms)(milliseconds to wait=w753) -> ()  [unwired: 1 out]
              }
              frame #1 {
                n409 = for {
                  tunnel: w757 -> [w759] mode=indexing
                  shift-right: [w760] -> w755
                  shift-left: string[] [] -> [w761]
                  n410 = Empty String/Path?(string/path=w759) -> (empty?=w758:bool)
                  n411 = case shown="False" w758 {
                    tunnel: w761 -> [w764 w770]
                    tunnel: [w763 w770] -> w760
                    tunnel: w759 -> [w762 _]
                    frame False {
                      n412 = call "send command.vi"("Device Name"=w762) -> ("status"=w765:bool)  [unwired: 4 in]
                      n413 = case shown="True" w765 {
                        tunnel: w764 -> [w766 w769]
                        tunnel: [w766 w768] -> w763
                        tunnel: w762 -> [_ w767]
                        frame False {
                        }
                        frame True {
                          n414 = Build Array (concatenate)(w769, w767) -> (w768:string[])
                        }
                      }
                    }
                    frame True {
                    }
                  }
                }
              }
            }
            n415 = Unbundle By Name(w719) -> ("active cams"=w714:string[])
            n416 = call <vilib>:"Add State(s) to Queue__jki_lib_state_machine.vi"("State(s) in (\"\")"=w727) -> ("States Out"=w711:string)  [unwired: 14 in]
            n417 = Empty Array?(array=w714) -> (empty?=w716:bool)
            n418 = Equal?(x=w714, y=w713) -> (x = y?=w717:bool[])
            n419 = Not(x=w716) -> (.not. x?=w715:bool)
            n420 = Build Array (concatenate)(w717, w715) -> (w718:bool[])
            n421 = And Array Elements(Boolean array=w718) -> (logical AND=w712:bool)
            n422 = case shown="False" w712 {
              tunnel: [w736 w749] -> w724
              tunnel: w719 -> [w735 w749]
              tunnel: w713 -> [w734 _]
              tunnel: w711 -> [w729 w748]
              tunnel: [w728 w748] -> w710
              frame False {
                n423 = Bundle By Name(cluster=w735, "active cams"=w734) -> (w737:T36)
                n424 = property on="active CCDs" class="LstBox (strict)"("Item Names"=w734) -> ()  [unwired: 2 in, 2 out]
                n425 = Array Size(array=w734) -> (size(s)=w740:i32)
                n426 = for {
                  N: 1 -> [_]
                  shift-right: [w742] -> w733
                  shift-left: timestamp[][] [] ("Time") -> [w744]
                  n427 = for {
                    N: 12 -> [_]
                    tunnel: w744 -> [w747] mode=indexing
                    tunnel: [w745] -> w742 mode=indexing
                    n428 = Get Date/Time In Seconds() -> (seconds since 1Jan1904=w746:timestamp)
                    n429 = Build Array (concatenate)(w747, w746) -> (w745:timestamp[])
                  }
                }
                n430 = Initialize Array(0.0 ("element"), w740, 0 ("dimension size")) -> (w738:dbl[][])
                n431 = Bundle By Name(cluster=w737, "Offset X stats"=w738, "Offset Y stats"=w738, "Centroid X"=w738, "Centroid Y"=w738, "Mean Centroid X"=w738, "Mean Centroid Y"=w738, "Offset X"=w738, "Offset Y"=w738, "Size"=w738, "Mean Size"=w738, "Motor X"=w738, "Motor Y"=w738) -> (w736:T36)
                n432 = property on="Time" class="Arr (strict)"("Value"=w733) -> ()  [unwired: 2 in, 2 out]
                n433 = call <vilib>:"Add State(s) to Queue__jki_lib_state_machine.vi"("State(s) in Front (\"\")"="newtdms\nMotor Config\nMove Config\nDetection Config\nactive\nCenter" ("State(s) in Front (\"\")"), "State(s) in (\"\")"=w729) -> ("States Out"=w728:string)  [unwired: 13 in]
                "name array" <- w734
              }
              frame True {
              }
            }
          }
          frame "Load Config" {
            # "Your code here.\n(You can make a copy of, or modify, this frame)"
            n434 = Unbundle By Name(w810) -> ("detection para"=w816:T3[], "move properties"=w813:T2[], "thresholds"=w805:cluster{"Lower value":sgl, "Upper value":sgl}[])
            n435 = call "File Dialog2"("error in"=w773, "pattern (all files)"="*.cfg", "pattern label"="config") -> ("selected path"=w820:path, "error out"=w772:errorcluster)  [unwired: 9 in, 2 out]
            n436 = property on="Load Config" class="Bool (strict)"("Value"=FALSE ("Load Config")) -> ()  [unwired: 2 in, 2 out]
            n437 = Open/Create/Replace File(file path (use dialog)=w820, error in=w772, operation (0:open)=T19."open or create") -> (refnum out=w824:refnum<file>, error out=w825:errorcluster)  [unwired: 3 in, 1 out]
            n438 = Read from Binary File(5:"output cluster 2", 8:w825, 11:w824) -> (0:w826:errorcluster, 2:w818:T5, 3:w827:refnum<file>)  [unwired: 3 in, 1 out]
            n439 = Close File(refnum=w827, error in=w826) -> (error out=w775:errorcluster)  [unwired: 1 out]
            n440 = Unbundle By Name(w818) -> ("Value"=w802:T7, "CCDs"=w817:string[], "detection para"=w815:T3[], "move properties"=w814:T2[], "thresholds"=w806:cluster{"Lower value":sgl, "Upper value":sgl}[])
            n441 = Cluster To Array(cluster=w802) -> (array=w803:u16[])
            n442 = call <vilib>:"Add State(s) to Queue__jki_lib_state_machine.vi"("State(s) in (\"\")"=w829, "State(s) at Back (\"\")"="Motor Config" ("State(s) at Back (\"\")")) -> ("States Out"=w828:string)  [unwired: 13 in]
            n443 = for {
              tunnel: w817 -> [w845]
              tunnel: w815 -> [w847]
              tunnel: w814 -> [w846]
              shift-right: [w839] -> w812
              shift-left: w816 -> [w844]
              shift-right: [w837] -> w811
              shift-left: w813 -> [w843]
              tunnel: w808 -> [w842] mode=indexing
              tunnel: w806 -> [w838]
              shift-right: [w834] -> w804
              shift-left: w805 -> [w836]
              tunnel: w803 -> [w833]
              tunnel: [w830] -> w801 mode=indexing
              i -> [w831]
              n444 = call-poly <userlib>:"Filter 1D Array__ogtk.vi"("items to filter"=w842, "array"=w845) -> ("filtered item indices"=w848:i32[])  [unwired: 4 in, 1 out]
              n445 = Index Array(array=w848) -> (element=w832:i32)  [unwired: 1 in]
              n446 = Index Array(array=w833, index=w832) -> (element=w830:u16)
              n447 = Index Array(array=w847, index=w832) -> (element=w841:T3)
              n448 = Index Array(array=w846, index=w832) -> (element=w840:T2)
              n449 = Index Array(array=w838, index=w832) -> (element=w835:cluster{"Lower value":sgl, "Upper value":sgl})
              n450 = Replace Array Subset(array=w844, new element=w841, index=w831) -> (w839:T3[])
              n451 = Replace Array Subset(array=w843, new element=w840, index=w831) -> (w837:T2[])
              n452 = Replace Array Subset(array=w836, new element=w835, index=w831) -> (w834:cluster{"Lower value":sgl, "Upper value":sgl}[])
            }
            n453 = Index Array(array=w801, index #1=0 ("index (row)"), index #2=1 ("index (row)"), index #3=2 ("index (row)"), index #4=3 ("index (row)"), index #5=4 ("index (row)"), index #6=5 ("index (row)"), index #7=6 ("index (row)"), index #8=7 ("index (row)"), index #9=8 ("index (row)"), index #10=9 ("index (row)"), index #11=10 ("index (row)"), index #12=11 ("index (row)")) -> (element #1=w788:u16, element #2=w787:u16, element #3=w786:u16, element #4=w785:u16, element #5=w784:u16, element #6=w783:u16, element #7=w782:u16, element #8=w781:u16, element #9=w780:u16, element #10=w779:u16, element #11=w778:u16, element #12=w777:u16)
            n454 = Bundle By Name(cluster=w802, "Motor CCD 1"=w788, "Motor CCD 2"=w787, "Motor CCD 3"=w786, "Motor CCD 4"=w785, "Motor CCD 5"=w784, "Motor CCD 6"=w783, "Motor CCD 7"=w782, "Motor CCD 8"=w781, "Motor CCD 9"=w780, "Motor CCD 10"=w779, "Motor CCD 11"=w778, "Motor CCD 12"=w777) -> (w776:T7)
            n455 = Bundle By Name(cluster=w810, "detection para"=w812, "move properties"=w811, "thresholds"=w804) -> (w809:T36)
            n456 = property on="associated motors" class="Clust (strict)"(error in=w775, "Val(Sgnl)"=w776) -> (error out=w774:errorcluster)  [unwired: 1 in, 1 out]
          }
          frame "Save Config" {
            # "Your code here.\n(You can make a copy of, or modify, this frame)"
            n457 = Unbundle By Name(w866) -> ("move properties"=w852:T2[], "detection para"=w861:T3[], "thresholds"=w849:cluster{"Lower value":sgl, "Upper value":sgl}[])
            n458 = property on="associated motors" class="Clust (strict)"() -> ("Value"=w860:T7)  [unwired: 2 in, 2 out]
            n459 = property on="Save Config" class="Bool (strict)"("Value"=FALSE ("Save Config")) -> ()  [unwired: 2 in, 2 out]
            n460 = local read "CCDs"() -> (w850:string[])
            n461 = call "File Dialog"("pattern (all files)"="*.cfg", "pattern label"="config") -> ("selected path"=w854:path)  [unwired: 10 in, 3 out]
            n462 = Bundle("CCDs"=w850, "move properties"=w852, "detection para"=w861, "thresholds"=w849, "Value"=w860) -> (w853:T5)  [unwired: 1 in]
            n463 = Open/Create/Replace File(file path (use dialog)=w854, error in=w858, operation (0:open)=T19."replace or create with confirmation") -> (refnum out=w862:refnum<file>, error out=w863:errorcluster)  [unwired: 3 in, 1 out]
            n464 = Write to Binary File(file (use dialog)=w862, data=w853, error in=w863) -> (refnum out=w865:refnum<file>, error out=w864:errorcluster)  [unwired: 3 in, 1 out]
            n465 = Close File(refnum=w865, error in=w864) -> (error out=w857:errorcluster)  [unwired: 1 out]
            n466 = call <vilib>:"Add State(s) to Queue__jki_lib_state_machine.vi"("State(s) in (\"\")"=w868) -> ("States Out"=w867:string)  [unwired: 14 in]
          }
          frame "active" {
            # "Your code here.\n(You can make a copy of, or modify, this frame)"
            n467 = call-poly <userlib>:"Filter 1D Array__ogtk.vi"("items to filter"=w878, "array"=w874) -> ("filtered item indices"=w877:i32[])  [unwired: 4 in, 1 out]
            n468 = Unbundle By Name(w873) -> ("move properties"=w876:T2[], "detection para"=w871:T3[])  [unwired: 1 out]
            n469 = Index Array(array=w877) -> (element=w869:i32)  [unwired: 1 in]
            n470 = Index Array(array=w876, index=w869) -> (element=w875:T2)
            n471 = Index Array(array=w871, index=w869) -> (element=w870:T3)
            n472 = property on="move config" class="Clust (strict)"("Value"=w875) -> ()  [unwired: 2 in, 2 out]
            n473 = property on="beam detection para" class="Clust (strict)"("Value"=w870) -> ()  [unwired: 2 in, 2 out]
            n474 = Bundle By Name(cluster=w873, "active ccd"=w869) -> (w872:T36)
            n475 = call <vilib>:"Add State(s) to Queue__jki_lib_state_machine.vi"("State(s) in (\"\")"=w881) -> ("States Out"=w880:string)  [unwired: 14 in]
          }
          frame "Detection Config" {
            # "Your code here.\n(You can make a copy of, or modify, this frame)"
            n476 = Unbundle By Name(w886) -> ("detection para"=w882:T3[], "active ccd"=w887:i32)
            n477 = Replace Array Subset(array=w882, new element="beam detection para", index=w887) -> (w883:T3[])
            n478 = Bundle By Name(cluster=w886, "detection para"=w883) -> (w885:T36)
            n479 = call <vilib>:"Add State(s) to Queue__jki_lib_state_machine.vi"("State(s) in (\"\")"=w890) -> ("States Out"=w889:string)  [unwired: 14 in]
          }
          frame "Motor Config" {
            # "Your code here.\n(You can make a copy of, or modify, this frame)"
            n480 = Unbundle By Name("associated motors") -> ("Motor CCD 1"=w910:u16, "Motor CCD 2"=w911:u16, "Motor CCD 3"=w912:u16, "Motor CCD 4"=w905:u16, "Motor CCD 5"=w904:u16, "Motor CCD 6"=w903:u16, "Motor CCD 7"=w902:u16, "Motor CCD 8"=w901:u16, "Motor CCD 9"=w900:u16, "Motor CCD 10"=w899:u16, "Motor CCD 11"=w898:u16, "Motor CCD 12"=w897:u16)
            n481 = local read "motor refs"() -> (w908:refnum<vi>[])
            n482 = property on="ActiveMotor" class="Ring (strict)"() -> ("Value"=w891:u16)  [unwired: 2 in, 2 out]
            n483 = property on="ActiveMotor" class="Ring (strict)"() -> ("Strings []"=w893:string[])  [unwired: 2 in, 2 out]
            n484 = Build Array(w910, w911, w912, w905, w904, w903, w902, w901, w900, w899, w898, w897) -> (w896:u16[])
            n485 = Increment(x=w896) -> (x+1=w895:u16[])
            n486 = Index Array(array=w893, index=w891) -> (element=w892:string)
            n487 = for {
              tunnel: w895 -> [w927] mode=indexing
              tunnel: w908 -> [w922]
              tunnel: [w916] -> w894 mode=indexing
              n488 = Multiply(x=w927, y=u16 3) -> (x*y=w923:u16)
              n489 = Subtract(x=w923, y=u16 3) -> (x-y=w921:u16)
              n490 = Subtract(x=w923, y=u16 2) -> (x-y=w920:u16)
              n491 = Index Array(array=w922, index=w921) -> (element=w919:refnum<vi>)
              n492 = Index Array(array=w922, index=w920) -> (element=w918:refnum<vi>)
              n493 = Bundle By Name(cluster="active Axis ref", "Ref X"=w919, "Ref Y"=w918) -> (w916:cluster{"Ref X":refnum<vi>, "Ref Y":refnum<vi>})
            }
            n494 = property on="ActiveMotorName::99" class="Str"("Val(Sgnl)"=w892) -> ()  [unwired: 2 in, 2 out]
            n495 = call <vilib>:"Add State(s) to Queue__jki_lib_state_machine.vi"("State(s) in (\"\")"=w915) -> ("States Out"=w914:string)  [unwired: 14 in]
            n496 = Bundle By Name(cluster=w907, "active axis refs 2"=w894) -> (w906:T36)
          }
          frame "Move Config" {
            # "Your code here.\n(You can make a copy of, or modify, this frame)"
            n497 = Unbundle By Name(w929) -> ("move properties"=w933:T2[], "active ccd"=w932:i32)
            n498 = Replace Array Subset(array=w933, new element="move config", index=w932) -> (w930:T2[])
            n499 = Bundle By Name(cluster=w929, "move properties"=w930) -> (w928:T36)
            n500 = call <vilib>:"Add State(s) to Queue__jki_lib_state_machine.vi"("State(s) in (\"\")"=w936) -> ("States Out"=w935:string)  [unwired: 14 in]
          }
          frame "----------Centroid & Move----------" {
            # "Template Separator\n(You can make a copy of, or modify, this frame)"
            n501 = call <vilib>:"Add State(s) to Queue__jki_lib_state_machine.vi"("State(s) in (\"\")"=w940) -> ("States Out"=w939:string)  [unwired: 14 in]
          }
          frame "detected" {
            n502 = Unbundle By Name(w968) -> ("Offset X"=w979:dbl[][], "Offset Y"=w978:dbl[][], "Size"=w977:dbl[][], "Mean Size"=w976:dbl[][], "Time"=w972:timestamp[][], "Motor X"=w948:dbl[][], "active axis refs 2"=w947:T12, "Motor Y"=w946:dbl[][])
            n503 = Spreadsheet String To Array(format string="%s", spreadsheet string=w952, array type (2D Dbl)=string[] []) -> (array=w942:string[])  [unwired: 1 in]
            n504 = for {
              tunnel: w943 -> [w992] mode=indexing
              tunnel: w942 -> [w991]
              tunnel: [w989] -> w941 mode=indexing
              n505 = for {
                tunnel: w992 -> [w995]
                tunnel: [w994] -> w990 mode=indexing
                tunnel: w991 -> [w993] mode=indexing
                n506 = Equal?(x=w995, y=w993) -> (x = y?=w994:bool)
              }
              n507 = Or Array Elements(Boolean array=w990) -> (logical OR=w989:bool)
            }
            n508 = call <vilib>:"Build State String with Arguments__jki_lib_state_machine.vi"("Arguments (\"\")"=w952, "State"="stats") -> ("State with Arguments"=w951:string)  [unwired: 4 in]
            n509 = Unbundle By Name(w968) -> ("Mean Centroid X"=w984:dbl[][], "Mean Centroid Y"=w983:dbl[][], "Centroid X"=w986:dbl[][], "Centroid Y"=w985:dbl[][])
            n510 = call <vilib>:"Add State(s) to Queue__jki_lib_state_machine.vi"("State(s) in (\"\")"=w950, "State(s) at Back (\"\")"=w951) -> ("States Out"=w949:string)  [unwired: 13 in]
            n511 = for {
              tunnel: w986 -> [w1045]
              tunnel: w985 -> [w1044]
              tunnel: w984 -> [w1043]
              tunnel: w983 -> [w1042]
              tunnel: [w1041] -> w967 mode=indexing
              tunnel: [w1040] -> w981 mode=indexing
              tunnel: w980 -> [w1011] mode=indexing
              tunnel: w979 -> [w1039]
              tunnel: w978 -> [w1038]
              tunnel: [w1037] -> w955 mode=indexing
              tunnel: [w1036] -> w970 mode=indexing
              tunnel: w977 -> [w1035]
              tunnel: w976 -> [w1034]
              tunnel: [w1033] -> w975 mode=indexing
              tunnel: w972 -> [w1032]
              tunnel: [w1031] -> w971 mode=indexing
              tunnel: w948 -> [w1003]
              tunnel: w947 -> [w1002]
              tunnel: w946 -> [w1001]
              tunnel: [w1000] -> w945 mode=indexing
              tunnel: [w999] -> w944 mode=indexing
              tunnel: w941 -> [w998]
              i -> [w997]
              n512 = Unbundle By Name(w1011) -> ("Target.X::12"=w1015:refnum<vi>, "Target.Y::12"=w1014:refnum<vi>)
              n513 = Index Array(array=w1003, index (row)=w997) -> (element=w1006:dbl[])  [unwired: 1 in]
              n514 = Index Array(array=w1002, index=w997) -> (element=w1005:cluster{"Ref X":refnum<vi>, "Ref Y":refnum<vi>})
              n515 = Index Array(array=w1001, index (row)=w997) -> (element=w1010:dbl[])  [unwired: 1 in]
              n516 = Index Array(array=w1043, index (row)=w997) -> (element=w1027:dbl[])  [unwired: 1 in]
              n517 = Index Array(array=w1042, index (row)=w997) -> (element=w1028:dbl[])  [unwired: 1 in]
              n518 = Index Array(array=w1045, index (row)=w997) -> (element=w1030:dbl[])  [unwired: 1 in]
              n519 = Index Array(array=w1044, index (row)=w997) -> (element=w1029:dbl[])  [unwired: 1 in]
              n520 = Index Array(array=w1039, index (row)=w997) -> (element=w1023:dbl[])  [unwired: 1 in]
              n521 = Index Array(array=w1038, index (row)=w997) -> (element=w1022:dbl[])  [unwired: 1 in]
              n522 = Index Array(array=w1035, index (row)=w997) -> (element=w1020:dbl[])  [unwired: 1 in]
              n523 = Index Array(array=w1034, index (row)=w997) -> (element=w1019:dbl[])  [unwired: 1 in]
              n524 = Index Array(array=w1032, index (row)=w997) -> (element=w1016:timestamp[])  [unwired: 1 in]
              n525 = Index Array(array=w998, index=w997) -> (element=w996:bool)
              n526 = Unbundle By Name(w1005) -> ("Ref X"=w1004:refnum<vi>, "Ref Y"=w1008:refnum<vi>)
              n527 = property class="DigNum (strict)"(reference=w1015) -> ("Value"=w1013:dbl)  [unwired: 1 in, 2 out]
              n528 = property class="DigNum (strict)"(reference=w1014) -> ("Value"=w1012:dbl)  [unwired: 1 in, 2 out]
              n529 = call <vilib>:"Std Deviation and Variance.vi"("X"=w1030) -> ("mean"=w1026:dbl)  [unwired: 1 in, 2 out]
              n530 = call <vilib>:"Std Deviation and Variance.vi"("X"=w1029) -> ("mean"=w1025:dbl)  [unwired: 1 in, 2 out]
              n531 = call <vilib>:"Std Deviation and Variance.vi"("X"=w1020) -> ("mean"=w1018:dbl)  [unwired: 1 in, 2 out]
              n532 = Get Date/Time In Seconds() -> (seconds since 1Jan1904=w1017:timestamp)
              n533 = property class="DigNum (strict)"(reference=w1004) -> ("Value"=w1007:dbl)  [unwired: 1 in, 2 out]
              n534 = property class="DigNum (strict)"(reference=w1008) -> ("Value"=w1009:dbl)  [unwired: 1 in, 2 out]
              n535 = Subtract(x=w1013, y=w1026) -> (x-y=w1024:dbl)
              n536 = Subtract(x=w1012, y=w1025) -> (x-y=w1021:dbl)
              n537 = case shown="False" w996 {
                tunnel: [w1063 w1077] -> w1041
                tunnel: [w1062 w1076] -> w1040
                tunnel: [w1061 w1075] -> w1037
                tunnel: [w1060 w1074] -> w1036
                tunnel: [w1059 w1073] -> w1033
                tunnel: [w1058 w1072] -> w1031
                tunnel: w1028 -> [w1057 w1071]
                tunnel: w1027 -> [w1056 w1070]
                tunnel: w1026 -> [w1055 _]
                tunnel: w1025 -> [w1054 _]
                tunnel: w1024 -> [w1053 _]
                tunnel: w1023 -> [w1052 w1069]
                tunnel: w1022 -> [w1051 w1068]
                tunnel: w1021 -> [w1050 _]
                tunnel: w1019 -> [w1049 w1067]
                tunnel: w1018 -> [w1048 _]
                tunnel: w1017 -> [w1047 w1066]
                tunnel: w1016 -> [w1046 w1065]
                frame True {
                  n538 = Build Array (concatenate)(w1056, w1055) -> (w1063:dbl[])
                  n539 = Build Array (concatenate)(w1057, w1054) -> (w1062:dbl[])
                  n540 = Build Array (concatenate)(w1052, w1053) -> (w1061:dbl[])
                  n541 = Build Array (concatenate)(w1051, w1050) -> (w1060:dbl[])
                  n542 = Build Array (concatenate)(w1049, w1048) -> (w1059:dbl[])
                  n543 = Build Array (concatenate)(w1046, w1047) -> (w1058:timestamp[])
                }
                frame False {
                  w1064 = 0.0
                  n544 = Build Array (concatenate)(w1070, w1064) -> (w1077:dbl[])
                  n545 = Build Array (concatenate)(w1071, w1064) -> (w1076:dbl[])
                  n546 = Build Array (concatenate)(w1069, w1064) -> (w1075:dbl[])
                  n547 = Build Array (concatenate)(w1068, w1064) -> (w1074:dbl[])
                  n548 = Build Array (concatenate)(w1067, w1064) -> (w1073:dbl[])
                  n549 = Build Array (concatenate)(w1065, w1066) -> (w1072:timestamp[])
                }
              }
              n550 = Build Array (concatenate)(w1010, w1009) -> (w999:dbl[])
              n551 = Build Array (concatenate)(w1006, w1007) -> (w1000:dbl[])
            }
            n552 = local write "Numeric"(0.0 ("Numeric")) -> ()
            n553 = Array Size(array=w955) -> (size(s)=w966:i32[])
            n554 = local read "Centroid X"() -> (w969:dbl[][])
            n555 = Index Array(array=w966, index=1) -> (element=w964:i32)
            "History index" <- w964
            n556 = local read "Size"() -> (w974:dbl[][])
            n557 = call <vilib>:"Add State(s) to Queue__jki_lib_state_machine.vi"("State(s) in (\"\")"=w949, "State(s) at Back (\"\")"="Check Move\ntdms" ("State(s) at Back (\"\")")) -> ("States Out"=w958:string)  [unwired: 13 in]
            n558 = Greater?(x=w964, y="History Size") -> (0:w962:bool)
            n559 = Bundle By Name(cluster=w968, "Centroid X"=w969, "Centroid Y"=w969, "Mean Centroid X"=w967, "Mean Centroid Y"=w981, "Offset X"=w955, "Offset Y"=w970, "Mean Size"=w975, "Size"=w974, "Time"=w971, "Motor X"=w945, "Motor Y"=w944) -> (w982:T36)
            n560 = Select(t="history" ("State(s) at Back (\"\")"), s=w962, f="") -> (s? t:f=w959:string)
            n561 = call <vilib>:"Add State(s) to Queue__jki_lib_state_machine.vi"("State(s) in (\"\")"=w958, "State(s) at Back (\"\")"=w959) -> ("States Out"=w957:string)  [unwired: 13 in]
          }
          frame "Check Move" {
            # "Your code here.\n(You can make a copy of, or modify, this frame)"
            n562 = Unbundle By Name(w1082) -> ("move properties"=w1085:T2[], "Mean Size"=w1108:dbl[][], "move properties"=w1111:T2[], "Offset X"=w1110:dbl[][], "Offset Y"=w1109:dbl[][], "active cams"=w1089:string[])
            n563 = for {
              tunnel: w1111 -> [w1201] mode=indexing
              tunnel: w1110 -> [w1203] mode=indexing
              tunnel: w1109 -> [w1202] mode=indexing
              tunnel: w1108 -> [w1200] mode=indexing
              tunnel: [w1179] -> w1107 mode=indexing
              tunnel: [w1175] -> w1106 mode=indexing
              tunnel: w1089 -> [w1197] mode=indexing
              tunnel: [w1199] -> w1105 mode=indexing
              tunnel: [w1198] -> w1104 mode=indexing
              tunnel: w1085 -> [w1196] mode=indexing
              tunnel: [w1173] -> w1083 mode=indexing
              tunnel: [w1168] -> w1079 mode=indexing
              tunnel: "Speedmode @" -> [w1167]
              n564 = Unbundle By Name(w1196) -> ("enable feedback"=w1178:bool)
              n565 = Unbundle By Name(w1201) -> ("Tolerance [%]"=w1190:dbl)
              n566 = Reverse 1D Array(array=w1203) -> (reversed array=w1195:dbl[])
              n567 = Reverse 1D Array(array=w1202) -> (reversed array=w1194:dbl[])
              n568 = Reverse 1D Array(array=w1200) -> (reversed array=w1189:dbl[])
              n569 = Index Array(array=w1195) -> (element=w1193:dbl)  [unwired: 1 in]
              n570 = Index Array(array=w1194) -> (element=w1192:dbl)  [unwired: 1 in]
              n571 = Index Array(array=w1189) -> (element=w1188:dbl)  [unwired: 1 in]
              n572 = Absolute Value(x=w1193) -> (abs(x)=w1174:dbl)
              n573 = Absolute Value(x=w1192) -> (abs(x)=w1171:dbl)
              n574 = Square Root(x=w1188) -> (sqrt(x)=w1187:dbl)
              n575 = Divide(x=w1190, y=100.0) -> (x/y=w1186:dbl)
              n576 = Multiply(x=w1187, y=w1186) -> (x*y=w1170:dbl)
              n577 = Not Equal To 0?(x=w1171) -> (x != 0?=w1176:bool)
              n578 = Not Equal To 0?(x=w1174) -> (x != 0?=w1181:bool)
              n579 = Greater Or Equal?(x=w1174, y=w1170) -> (x >= y?=w1180:bool)
              n580 = Greater Or Equal?(x=w1171, y=w1170) -> (x >= y?=w1177:bool)
              n581 = Divide(x=w1174, y=w1170) -> (x/y=w1172:dbl)
              n582 = Divide(x=w1171, y=w1170) -> (x/y=w1169:dbl)
              n583 = Compound Arithmetic op=AND(w1178, w1181, w1180) -> (w1179:bool)
              n584 = Compound Arithmetic op=AND(w1178, w1177, w1176) -> (w1175:bool)
              n585 = Boolean To (0,1)(Boolean=w1175) -> (0, 1=w1182:i16)
              n586 = Greater?(x=w1172, y=w1167) -> (0:w1173:bool)
              n587 = Greater?(x=w1169, y=w1167) -> (0:w1168:bool)
              n588 = Multiply(x=w1182, y=w1171) -> (x*y=w1183:dbl)
              n589 = Boolean To (0,1)(Boolean=w1179) -> (0, 1=w1185:i16)
              n590 = Multiply(x=w1185, y=w1174) -> (x*y=w1184:dbl)
              n591 = Bundle(w1183, "GUIdevice 8"=w1197) -> (w1198:cluster{dbl, "GUIdevice 8":string})  [unwired: 1 in]
              n592 = Bundle(w1184, "GUIdevice 8"=w1197) -> (w1199:cluster{dbl, "GUIdevice 8":string})  [unwired: 1 in]
            }
            "required X" <- w1107
            "required Y" <- w1106
            "speedmode X" <- w1083
            "speedmode Y" <- w1079
            n593 = case shown="True" "Align" {
              tunnel: w1105 -> [w1119 w1124]
              tunnel: w1104 -> [w1118 w1121]
              tunnel: [w1117 w1123] -> w1101
              tunnel: [w1116 w1120] -> w1095
              frame False {
                n594 = Sort 1D Array(array=w1118) -> (sorted array=w1115:cluster{dbl, "GUIdevice 8":string}[])
                n595 = Sort 1D Array(array=w1119) -> (sorted array=w1114:cluster{dbl, "GUIdevice 8":string}[])
                n596 = Reverse 1D Array(array=w1115) -> (reversed array=w1116:cluster{dbl, "GUIdevice 8":string}[])
                n597 = Reverse 1D Array(array=w1114) -> (reversed array=w1117:cluster{dbl, "GUIdevice 8":string}[])
              }
              frame True {
                w1122 = cluster{dbl, "GUIdevice 8":string}[] [] ("Array")
                n598 = for {
                  shift-right: [w1134] -> w1123
                  shift-left: w1122 -> [w1136]
                  tunnel: w1124 -> [w1135] mode=indexing
                  n599 = Unbundle(w1135) -> (w1138:dbl)  [unwired: 1 out]
                  n600 = Not Equal To 0?(x=w1138) -> (x != 0?=w1137:bool)
                  n601 = case shown="True" w1137 {
                    tunnel: w1136 -> [w1139 w1142]
                    tunnel: w1135 -> [_ w1141]
                    tunnel: [w1139 w1140] -> w1134
                    frame False {
                    }
                    frame True {
                      n602 = Build Array (concatenate)(w1142, w1141) -> (w1140:cluster{dbl, "GUIdevice 8":string}[])
                    }
                  }
                }
                n603 = for {
                  shift-right: [w1125] -> w1120
                  shift-left: w1122 -> [w1127]
                  tunnel: w1121 -> [w1126] mode=indexing
                  n604 = Unbundle(w1126) -> (w1129:dbl)  [unwired: 1 out]
                  n605 = Not Equal To 0?(x=w1129) -> (x != 0?=w1128:bool)
                  n606 = case shown="True" w1128 {
                    tunnel: w1127 -> [w1130 w1133]
                    tunnel: w1126 -> [_ w1132]
                    tunnel: [w1130 w1131] -> w1125
                    frame False {
                    }
                    frame True {
                      n607 = Build Array (concatenate)(w1133, w1132) -> (w1131:cluster{dbl, "GUIdevice 8":string}[])
                    }
                  }
                }
              }
            }
            n608 = call <vilib>:"Add State(s) to Queue__jki_lib_state_machine.vi"("State(s) in (\"\")"=w1088) -> ("States Out"=w1087:string)  [unwired: 14 in]
            n609 = Bundle By Name(cluster=w1082, "speedmode X"=w1083, "speedmode Y"=w1079) -> (w1081:T36)
            n610 = Empty Array?(array=w1101) -> (empty?=w1098:bool)
            n611 = Empty Array?(array=w1095) -> (empty?=w1093:bool)
            n612 = Index Array(array=w1101) -> (element=w1091:cluster{dbl, "GUIdevice 8":string})  [unwired: 1 in]
            n613 = Index Array(array=w1095) -> (element=w1090:cluster{dbl, "GUIdevice 8":string})  [unwired: 1 in]
            n614 = Unbundle(w1091) -> (w1100:dbl)  [unwired: 1 out]
            n615 = Unbundle(w1090) -> (w1096:dbl)  [unwired: 1 out]
            n616 = Equal To 0?(x=w1100) -> (x = 0?=w1099:bool)
            n617 = Equal To 0?(x=w1096) -> (x = 0?=w1094:bool)
            n618 = property on="autodetect" class="Bool (strict)"("Value"=FALSE ("autodetect")) -> ()  [unwired: 2 in, 2 out]
            n619 = Unbundle By Name(w1081) -> ("Feedback global"=w1102:bool)
            n620 = Or(x=w1099, y=w1098) -> (x .or. y?=w1097:bool)
            n621 = Or(x=w1094, y=w1093) -> (x .or. y?=w1092:bool)
            n622 = case shown="True" w1102 {
              tunnel: w1097 -> [_ w1150]
              tunnel: w1101 -> [_ w1149]
              tunnel: w1092 -> [_ w1147]
              tunnel: w1095 -> [_ w1146]
              tunnel: w1087 -> [w1143 w1145]
              tunnel: [w1143 w1144] -> w1103
              frame False {
              }
              frame True {
                n623 = case shown="False" w1150 {
                  tunnel: w1149 -> [w1165 _]
                  tunnel: w1145 -> [w1161 w1166]
                  tunnel: [w1159 w1166] -> w1148
                  frame False {
                    n624 = Index Array(array=w1165) -> (element=w1164:cluster{dbl, "GUIdevice 8":string})  [unwired: 1 in]
                    n625 = Unbundle By Name(w1164) -> ("GUIdevice 8"=w1163:string)
                    n626 = call <vilib>:"Build State String with Arguments__jki_lib_state_machine.vi"("Arguments (\"\")"=w1163, "State"="Move X") -> ("State with Arguments"=w1160:string)  [unwired: 4 in]
                    n627 = call <vilib>:"Add State(s) to Queue__jki_lib_state_machine.vi"("State(s) in (\"\")"=w1161, "State(s) at Back (\"\")"=w1160) -> ("States Out"=w1159:string)  [unwired: 13 in]
                  }
                  frame True {
                  }
                }
                n628 = case shown="False" w1147 {
                  tunnel: w1146 -> [w1157 _]
                  tunnel: w1148 -> [w1153 w1158]
                  tunnel: [w1151 w1158] -> w1144
                  frame False {
                    n629 = Index Array(array=w1157) -> (element=w1156:cluster{dbl, "GUIdevice 8":string})  [unwired: 1 in]
                    n630 = Unbundle By Name(w1156) -> ("GUIdevice 8"=w1155:string)
                    n631 = call <vilib>:"Build State String with Arguments__jki_lib_state_machine.vi"("Arguments (\"\")"=w1155, "State"="Move Y") -> ("State with Arguments"=w1152:string)  [unwired: 4 in]
                    n632 = call <vilib>:"Add State(s) to Queue__jki_lib_state_machine.vi"("State(s) in (\"\")"=w1153, "State(s) at Back (\"\")"=w1152) -> ("States Out"=w1151:string)  [unwired: 13 in]
                  }
                  frame True {
                  }
                }
              }
            }
            n633 = call <vilib>:"Add State(s) to Queue__jki_lib_state_machine.vi"("State(s) in Front (\"\")"="Device Ini" ("State(s) in Front (\"\")"), "State(s) in (\"\")"=w1087, "State(s) at Back (\"\")"=w1103) -> ("States Out"=w1113:string)  [unwired: 12 in]
          }
          frame "Move X" {
            # "Your code here.\n(You can make a copy of, or modify, this frame)"
            n634 = Unbundle By Name(w1227) -> ("Offset X"=w1226:dbl[][])
            n635 = call-poly <userlib>:"Filter 1D Array__ogtk.vi"("items to filter"=w1211, "array"=w1231) -> ("filtered item indices"=w1215:i32[])  [unwired: 4 in, 1 out]
            n636 = Unbundle By Name(w1227) -> ("speedmode X"=w1210:bool[], "active axis refs 2"=w1230:T12, "move properties"=w1214:T2[])
            n637 = for {
              tunnel: w1215 -> [w1236] mode=indexing
              tunnel: w1214 -> [w1240]
              shift-right: [w1235] -> w1212
              shift-left: i32[] [] ("filtered item indices") -> [w1238]
              n638 = Index Array(array=w1240, index=w1236) -> (element=w1239:T2)
              n639 = Unbundle By Name(w1239) -> ("enable feedback"=w1237:bool)
              n640 = case shown="True" w1237 {
                tunnel: w1238 -> [w1241 w1244]
                tunnel: w1236 -> [_ w1243]
                tunnel: [w1241 w1242] -> w1235
                frame False {
                }
                frame True {
                  n641 = Build Array (concatenate)(w1244, w1243) -> (w1242:i32[])
                }
              }
            }
            n642 = Index Array(array=w1212) -> (element=w1209:i32)  [unwired: 1 in]
            n643 = Index Array(array=w1226, index (row)=w1209) -> (element=w1225:dbl[])  [unwired: 1 in]
            n644 = Reverse 1D Array(array=w1225) -> (reversed array=w1224:dbl[])
            n645 = Index Array(array=w1230, index=w1209) -> (element=w1229:cluster{"Ref X":refnum<vi>, "Ref Y":refnum<vi>})
            n646 = Index Array(array=w1224) -> (element=w1222:dbl)  [unwired: 1 in]
            n647 = Index Array(array=w1214, index=w1209) -> (element=w1228:T2)
            n648 = Unbundle By Name(w1229) -> ("Ref X"=w1219:refnum<vi>, "Ref Y"=w1218:refnum<vi>)
            n649 = Index Array(array=w1210, index=w1209) -> (element=w1208:bool)
            n650 = Unbundle By Name(w1228) -> ("Invert Direction X"=w1220:bool, "Invert Axis"=w1223:bool, "Stepsize"=w1206:dbl, "enable feedback"=w1217:bool)
            n651 = Greater Or Equal To 0?(x=w1222) -> (x >= 0?=w1221:bool)
            n652 = call <vilib>:"Add State(s) to Queue__jki_lib_state_machine.vi"("State(s) in Front (\"\")"="Wait" ("State(s) in Front (\"\")"), "State(s) in (\"\")"=w1234) -> ("States Out"=w1233:string)  [unwired: 13 in]
            n653 = property on="Speedmode @" class="DigNum (strict)"() -> ("Value"=w1205:dbl)  [unwired: 2 in, 2 out]
            n654 = Multiply(x=w1205, y=w1206) -> (x*y=w1207:dbl)
            n655 = Select(t=w1207, s=w1208, f=w1206) -> (s? t:f=w1204:dbl)
            n656 = case shown="True" w1217 {
              tunnel: w1223 -> [_ w1250]
              tunnel: w1221 -> [_ w1249]
              tunnel: w1204 -> [_ w1248]
              tunnel: w1220 -> [_ w1247]
              tunnel: w1219 -> [_ w1246]
              tunnel: w1218 -> [_ w1245]
              frame False {
              }
              frame True {
                n657 = case shown="False" w1249 {
                  tunnel: w1247 -> [w1258 w1280]
                  tunnel: w1248 -> [w1256 w1278]
                  tunnel: w1250 -> [w1255 w1277]
                  tunnel: w1250 -> [w1254 w1276]
                  tunnel: w1246 -> [w1252 w1274]
                  tunnel: w1245 -> [w1251 w1273]
                  frame True {
                    n658 = case shown="False" w1255 {
                      tunnel: [w1269 w1271] -> w1257
                      tunnel: w1252 -> [w1270 _]
                      tunnel: w1251 -> [_ w1272]
                      frame False {
                        n659 = property class="DigNum (strict)"(reference=w1270) -> ("Value"=w1269:dbl)  [unwired: 1 in, 2 out]
                      }
                      frame True {
                        n660 = property class="DigNum (strict)"(reference=w1272) -> ("Value"=w1271:dbl)  [unwired: 1 in, 2 out]
                      }
                    }
                    n661 = case shown="False" w1258 {
                      tunnel: w1257 -> [w1265 w1268]
                      tunnel: w1256 -> [w1264 w1267]
                      tunnel: [w1263 w1266] -> w1253
                      frame False {
                        n662 = Add(x=w1265, y=w1264) -> (x+y=w1263:dbl)
                      }
                      frame True {
                        n663 = Subtract(x=w1268, y=w1267) -> (x-y=w1266:dbl)
                      }
                    }
                    n664 = case shown="False" w1254 {
                      tunnel: w1253 -> [w1259 w1261]
                      tunnel: w1252 -> [w1260 _]
                      tunnel: w1251 -> [_ w1262]
                      frame False {
                        n665 = property class="DigNum (strict)"(reference=w1260, "Val(Sgnl)"=w1259) -> ()  [unwired: 1 in, 2 out]
                      }
                      frame True {
                        n666 = property class="DigNum (strict)"(reference=w1262, "Val(Sgnl)"=w1261) -> ()  [unwired: 1 in, 2 out]
                      }
                    }
                  }
                  frame False {
                    n667 = case shown="False" w1277 {
                      tunnel: [w1291 w1293] -> w1279
                      tunnel: w1274 -> [w1292 _]
                      tunnel: w1273 -> [_ w1294]
                      frame False {
                        n668 = property class="DigNum (strict)"(reference=w1292) -> ("Value"=w1291:dbl)  [unwired: 1 in, 2 out]
                      }
                      frame True {
                        n669 = property class="DigNum (strict)"(reference=w1294) -> ("Value"=w1293:dbl)  [unwired: 1 in, 2 out]
                      }
                    }
                    n670 = case shown="False" w1280 {
                      tunnel: w1279 -> [w1287 w1290]
                      tunnel: w1278 -> [w1286 w1289]
                      tunnel: [w1285 w1288] -> w1275
                      frame False {
                        n671 = Subtract(x=w1287, y=w1286) -> (x-y=w1285:dbl)
                      }
                      frame True {
                        n672 = Add(x=w1290, y=w1289) -> (x+y=w1288:dbl)
                      }
                    }
                    n673 = case shown="False" w1276 {
                      tunnel: w1275 -> [w1281 w1283]
                      tunnel: w1274 -> [w1282 _]
                      tunnel: w1273 -> [_ w1284]
                      frame False {
                        n674 = property class="DigNum (strict)"(reference=w1282, "Val(Sgnl)"=w1281) -> ()  [unwired: 1 in, 2 out]
                      }
                      frame True {
                        n675 = property class="DigNum (strict)"(reference=w1284, "Val(Sgnl)"=w1283) -> ()  [unwired: 1 in, 2 out]
                      }
                    }
                  }
                }
              }
            }
            "Arguments X" <- w1211
            "Moving X" <- w1211
          }
          frame "Move Y" {
            # "Your code here.\n(You can make a copy of, or modify, this frame)"
            n676 = Unbundle By Name(w1318) -> ("Offset Y"=w1317:dbl[][])
            n677 = call-poly <userlib>:"Filter 1D Array__ogtk.vi"("items to filter"=w1302, "array"=w1322) -> ("filtered item indices"=w1307:i32[])  [unwired: 4 in, 1 out]
            n678 = Unbundle By Name(w1318) -> ("speedmode Y"=w1301:bool[], "active axis refs 2"=w1321:T12, "move properties"=w1305:T2[])
            n679 = for {
              tunnel: w1307 -> [w1327] mode=indexing
              tunnel: w1305 -> [w1331]
              shift-right: [w1326] -> w1306
              shift-left: i32[] [] ("filtered item indices") -> [w1329]
              n680 = Index Array(array=w1331, index=w1327) -> (element=w1330:T2)
              n681 = Unbundle By Name(w1330) -> ("enable feedback"=w1328:bool)
              n682 = case shown="True" w1328 {
                tunnel: w1329 -> [w1332 w1335]
                tunnel: w1327 -> [_ w1334]
                tunnel: [w1332 w1333] -> w1326
                frame False {
                }
                frame True {
                  n683 = Build Array (concatenate)(w1335, w1334) -> (w1333:i32[])
                }
              }
            }
            n684 = Index Array(array=w1306) -> (element=w1300:i32)  [unwired: 1 in]
            n685 = Index Array(array=w1317, index (row)=w1300) -> (element=w1316:dbl[])  [unwired: 1 in]
            n686 = Reverse 1D Array(array=w1316) -> (reversed array=w1315:dbl[])
            n687 = Index Array(array=w1321, index=w1300) -> (element=w1320:cluster{"Ref X":refnum<vi>, "Ref Y":refnum<vi>})
            n688 = Index Array(array=w1315) -> (element=w1313:dbl)  [unwired: 1 in]
            n689 = Index Array(array=w1305, index=w1300) -> (element=w1319:T2)
            n690 = Index Array(array=w1301, index=w1300) -> (element=w1299:bool)
            n691 = Unbundle By Name(w1320) -> ("Ref Y"=w1310:refnum<vi>, "Ref X"=w1309:refnum<vi>)
            n692 = Unbundle By Name(w1319) -> ("Invert Direction Y"=w1311:bool, "Invert Axis"=w1314:bool, "Stepsize"=w1297:dbl, "enable feedback"=w1308:bool)
            n693 = Greater Or Equal To 0?(x=w1313) -> (x >= 0?=w1312:bool)
            n694 = call <vilib>:"Add State(s) to Queue__jki_lib_state_machine.vi"("State(s) in Front (\"\")"="Wait" ("State(s) in Front (\"\")"), "State(s) in (\"\")"=w1325) -> ("States Out"=w1324:string)  [unwired: 13 in]
            n695 = property on="Speedmode @" class="DigNum (strict)"() -> ("Value"=w1296:dbl)  [unwired: 2 in, 2 out]
            n696 = Multiply(x=w1296, y=w1297) -> (x*y=w1295:dbl)
            n697 = Select(t=w1295, s=w1299, f=w1297) -> (s? t:f=w1298:dbl)
            n698 = case shown="True" w1308 {
              tunnel: w1314 -> [_ w1341]
              tunnel: w1312 -> [_ w1340]
              tunnel: w1298 -> [_ w1339]
              tunnel: w1311 -> [_ w1338]
              tunnel: w1310 -> [_ w1337]
              tunnel: w1309 -> [_ w1336]
              frame False {
              }
              frame True {
                n699 = case shown="True" w1340 {
                  tunnel: w1338 -> [w1349 w1371]
                  tunnel: w1339 -> [w1347 w1369]
                  tunnel: w1341 -> [w1346 w1368]
                  tunnel: w1341 -> [w1345 w1367]
                  tunnel: w1337 -> [w1343 w1365]
                  tunnel: w1336 -> [w1342 w1364]
                  frame True {
                    n700 = case shown="False" w1346 {
                      tunnel: [w1360 w1362] -> w1348
                      tunnel: w1343 -> [w1361 _]
                      tunnel: w1342 -> [_ w1363]
                      frame False {
                        n701 = property class="DigNum (strict)"(reference=w1361) -> ("Value"=w1360:dbl)  [unwired: 1 in, 2 out]
                      }
                      frame True {
                        n702 = property class="DigNum (strict)"(reference=w1363) -> ("Value"=w1362:dbl)  [unwired: 1 in, 2 out]
                      }
                    }
                    n703 = case shown="False" w1349 {
                      tunnel: w1348 -> [w1356 w1359]
                      tunnel: w1347 -> [w1355 w1358]
                      tunnel: [w1354 w1357] -> w1344
                      frame False {
                        n704 = Add(x=w1356, y=w1355) -> (x+y=w1354:dbl)
                      }
                      frame True {
                        n705 = Subtract(x=w1359, y=w1358) -> (x-y=w1357:dbl)
                      }
                    }
                    n706 = case shown="False" w1345 {
                      tunnel: w1344 -> [w1350 w1352]
                      tunnel: w1343 -> [w1351 _]
                      tunnel: w1342 -> [_ w1353]
                      frame False {
                        n707 = property class="DigNum (strict)"(reference=w1351, "Val(Sgnl)"=w1350) -> ()  [unwired: 1 in, 2 out]
                      }
                      frame True {
                        n708 = property class="DigNum (strict)"(reference=w1353, "Val(Sgnl)"=w1352) -> ()  [unwired: 1 in, 2 out]
                      }
                    }
                  }
                  frame False {
                    n709 = case shown="False" w1368 {
                      tunnel: [w1382 w1384] -> w1370
                      tunnel: w1365 -> [w1383 _]
                      tunnel: w1364 -> [_ w1385]
                      frame False {
                        n710 = property class="DigNum (strict)"(reference=w1383) -> ("Value"=w1382:dbl)  [unwired: 1 in, 2 out]
                      }
                      frame True {
                        n711 = property class="DigNum (strict)"(reference=w1385) -> ("Value"=w1384:dbl)  [unwired: 1 in, 2 out]
                      }
                    }
                    n712 = case shown="False" w1371 {
                      tunnel: w1370 -> [w1378 w1381]
                      tunnel: w1369 -> [w1377 w1380]
                      tunnel: [w1376 w1379] -> w1366
                      frame False {
                        n713 = Subtract(x=w1378, y=w1377) -> (x-y=w1376:dbl)
                      }
                      frame True {
                        n714 = Add(x=w1381, y=w1380) -> (x+y=w1379:dbl)
                      }
                    }
                    n715 = case shown="False" w1367 {
                      tunnel: w1366 -> [w1372 w1374]
                      tunnel: w1365 -> [w1373 _]
                      tunnel: w1364 -> [_ w1375]
                      frame False {
                        n716 = property class="DigNum (strict)"(reference=w1373, "Val(Sgnl)"=w1372) -> ()  [unwired: 1 in, 2 out]
                      }
                      frame True {
                        n717 = property class="DigNum (strict)"(reference=w1375, "Val(Sgnl)"=w1374) -> ()  [unwired: 1 in, 2 out]
                      }
                    }
                  }
                }
              }
            }
            "Arguments Y" <- w1302
            "Moving Y" <- w1302
          }
          frame "Wait" {
            # "Your code here.\n(You can make a copy of, or modify, this frame)"
            n718 = flat-sequence {
              frame #0 {
                n719 = Wait (ms)(milliseconds to wait=u32 300) -> ()  [unwired: 1 out]
              }
              frame #1 {
                n720 = property on="Moving Y" class="Str"("Value"="") -> ()  [unwired: 2 in, 2 out]
                n721 = property on="Moving X" class="Str"("Value"="") -> ()  [unwired: 2 in, 2 out]
              }
            }
            n722 = call <vilib>:"Add State(s) to Queue__jki_lib_state_machine.vi"("State(s) in (\"\")"=w1391) -> ("States Out"=w1390:string)  [unwired: 14 in]
            n723 = local read "Mean Centroid X"() -> (w1386:dbl[][])
            n724 = Bundle By Name(cluster=w1388, "Mean Centroid X"=w1386, "Mean Centroid Y"=w1386) -> (w1387:T36)
          }
          frame "stats" {
            # "Your code here.\n(You can make a copy of, or modify, this frame)"
            n725 = Unbundle By Name(w1400) -> ("Offset X"=w1399:dbl[][], "Offset Y"=w1398:dbl[][], "Time"=w1397:timestamp[][], "Motor X"=w1396:dbl[][], "Motor Y"=w1395:dbl[][])
            n726 = for {
              tunnel: w1398 -> [w1438]
              tunnel: w1397 -> [w1439]
              tunnel: w1399 -> [w1440]
              tunnel: [w1443] -> w1426 mode=indexing
              tunnel: w1396 -> [w1437]
              tunnel: w1395 -> [w1436]
              tunnel: w1401 -> [_] mode=indexing
              i -> [w1430]
              n727 = Index Array(array=w1438, index (row)=w1430) -> (element=w1434:dbl[])  [unwired: 1 in]
              n728 = Index Array(array=w1437, index (row)=w1430) -> (element=w1432:dbl[])  [unwired: 1 in]
              n729 = Index Array(array=w1436, index (row)=w1430) -> (element=w1431:dbl[])  [unwired: 1 in]
              n730 = Index Array(array=w1440, index (row)=w1430) -> (element=w1435:dbl[])  [unwired: 1 in]
              n731 = Index Array(array=w1439, index (row)=w1430) -> (element=w1433:timestamp[])  [unwired: 1 in]
              n732 = Bundle("Time"=w1433, "Motor X"=w1432) -> (w1442:cluster{"Time":timestamp[], "Motor X":dbl[]})  [unwired: 1 in]
              n733 = Bundle("Time"=w1433, "Motor Y"=w1431) -> (w1441:cluster{"Time":timestamp[], "Motor Y":dbl[]})  [unwired: 1 in]
              n734 = Bundle("Time"=w1433, "Offset X"=w1435) -> (w1444:cluster{"Time":timestamp[], "Offset X":dbl[]})  [unwired: 1 in]
              n735 = Bundle("Time"=w1433, "Offset Y"=w1434) -> (w1445:cluster{"Time":timestamp[], "Offset Y":dbl[]})  [unwired: 1 in]
              n736 = Build Array(w1445, w1444, w1442, w1441) -> (w1443:cluster{"Time":timestamp[], "Motor Y":dbl[]}[])
            }
            n737 = call <vilib>:"Add State(s) to Queue__jki_lib_state_machine.vi"("State(s) in (\"\")"=w1429) -> ("States Out"=w1428:string)  [unwired: 14 in]
            n738 = Index Array(array=w1426, index (row) #1=0 ("index (row)"), index (row) #2=1 ("index (row)"), index (row) #3=2 ("index (row)"), index (row) #4=3 ("index (row)"), index (row) #5=4 ("index (row)"), index (row) #6=5 ("index (row)"), index (row) #7=6 ("index (row)"), index (row) #8=7 ("index (row)"), index (row) #9=8 ("index (row)"), index (row) #10=9 ("index (row)"), index (row) #11=10 ("index (row)"), index (row) #12=11 ("index (row)")) -> (element #1=→"CCD 1":cluster{"Time":timestamp[], "Motor Y":dbl[]}[], element #2=→"CCD 2":cluster{"Time":timestamp[], "Motor Y":dbl[]}[], element #3=→"CCD 3":cluster{"Time":timestamp[], "Motor Y":dbl[]}[], element #4=→"CCD 4":cluster{"Time":timestamp[], "Motor Y":dbl[]}[], element #5=→"CCD 5":cluster{"Time":timestamp[], "Motor Y":dbl[]}[], element #6=→"CCD 6":cluster{"Time":timestamp[], "Motor Y":dbl[]}[], element #7=→"CCD 7":cluster{"Time":timestamp[], "Motor Y":dbl[]}[], element #8=→"CCD 8":cluster{"Time":timestamp[], "Motor Y":dbl[]}[], element #9=→"CCD 9":cluster{"Time":timestamp[], "Motor Y":dbl[]}[], element #10=→"CCD 10":cluster{"Time":timestamp[], "Motor Y":dbl[]}[], element #11=→"CCD 11":cluster{"Time":timestamp[], "Motor Y":dbl[]}[], element #12=→"CCD 12":cluster{"Time":timestamp[], "Motor Y":dbl[]}[])  [unwired: 12 in]
          }
          frame "---------------Statistics--------------" {
            # "Template Separator\n(You can make a copy of, or modify, this frame)"
            n739 = call <vilib>:"Add State(s) to Queue__jki_lib_state_machine.vi"("State(s) in (\"\")"=w1449) -> ("States Out"=w1448:string)  [unwired: 14 in]
          }
          frame "Save Stats" {
            # "Your code here.\n(You can make a copy of, or modify, this frame)"
            n740 = property on="CCD 1" class="XYGraph (strict)"() -> ("Value"=w1459:cluster{timestamp[], dbl[]}[])  [unwired: 2 in, 2 out]
            n741 = property on="CCD 2" class="XYGraph (strict)"() -> ("Value"=w1458:cluster{timestamp[], dbl[]}[])  [unwired: 2 in, 2 out]
            n742 = property on="CCD 3" class="XYGraph (strict)"() -> ("Value"=w1457:cluster{timestamp[], dbl[]}[])  [unwired: 2 in, 2 out]
            n743 = property on="CCD 4" class="XYGraph (strict)"() -> ("Value"=w1456:cluster{timestamp[], dbl[]}[])  [unwired: 2 in, 2 out]
            n744 = property on="CCD 5" class="XYGraph (strict)"() -> ("Value"=w1455:cluster{timestamp[], dbl[]}[])  [unwired: 2 in, 2 out]
            n745 = property on="CCD 6" class="XYGraph (strict)"() -> ("Value"=w1454:cluster{timestamp[], dbl[]}[])  [unwired: 2 in, 2 out]
            n746 = property on="CCD 7" class="XYGraph (strict)"() -> ("Value"=w1453:cluster{timestamp[], dbl[]}[])  [unwired: 2 in, 2 out]
            n747 = property on="CCD 8" class="XYGraph (strict)"() -> ("Value"=w1452:cluster{timestamp[], dbl[]}[])  [unwired: 2 in, 2 out]
            n748 = Build Array(w1459, w1458, w1457, w1456, w1455, w1454, w1453, w1452) -> (w1451:cluster{timestamp[], dbl[]}[][])
            n749 = for {
              tunnel: w1451 -> [w1467] mode=indexing
              tunnel: w1450 -> [w1466] mode=indexing
              n750 = Empty String/Path?(string/path=w1466) -> (empty?=w1465:bool)
              n751 = case shown="False" w1465 {
                tunnel: w1467 -> [w1473 _]
                tunnel: w1466 -> [w1471 _]
                frame False {
                  n752 = Index Array(array=w1473, index #1=0 ("index"), index #2=1 ("index"), index #3=2 ("index"), index #4=3 ("index")) -> (element #1=w1508:cluster{timestamp[], dbl[]}, element #2=w1502:cluster{timestamp[], dbl[]}, element #3=w1501:cluster{timestamp[], dbl[]}, element #4=w1500:cluster{timestamp[], dbl[]})  [unwired: 1 in, 1 out]
                  n753 = Concatenate Strings(w1471, ".dat" ("string")) -> (w1469:string)
                  n754 = Unbundle(w1508) -> (w1507:timestamp[], w1485:dbl[])
                  n755 = Unbundle(w1502) -> (w1476:dbl[])  [unwired: 1 out]
                  n756 = Unbundle(w1501) -> (w1475:dbl[])  [unwired: 1 out]
                  n757 = Unbundle(w1500) -> (w1474:dbl[])  [unwired: 1 out]
                  n758 = Build Path(base path="save path", name or relative path=w1469) -> (appended path=w1468:path)
                  n759 = for {
                    tunnel: w1507 -> [w1510] mode=indexing
                    tunnel: [w1509] -> w1483 mode=indexing
                    n760 = Format Date/Time String(time format string (%c)="%Y%m%d%H%M%S", seconds (now)=w1510) -> (date/time string=w1509:string)  [unwired: 1 in]
                  }
                  n761 = Array Size(array=w1485) -> (size(s)=w1486:i32)
                  n762 = Number To Fractional String(number=w1485) -> (F-format string=w1482:string[])  [unwired: 3 in]
                  n763 = Number To Fractional String(number=w1476) -> (F-format string=w1479:string[])  [unwired: 3 in]
                  n764 = Number To Fractional String(number=w1475) -> (F-format string=w1478:string[])  [unwired: 3 in]
                  n765 = Number To Fractional String(number=w1474) -> (F-format string=w1477:string[])  [unwired: 3 in]
                  n766 = Initialize Array("", w1486, 5 ("dimension size")) -> (w1484:string[][])
                  n767 = Insert Into Array(array=w1484, index (col)=0 ("disabled index (col)"), new element=w1483) -> (w1494:string[][])  [unwired: 1 in]
                  n768 = Insert Into Array(array=w1494, index (col)=1 ("disabled index (col)"), new element=w1482) -> (w1493:string[][])  [unwired: 1 in]
                  n769 = Insert Into Array(array=w1493, index (col)=2 ("disabled index (col)"), new element=w1479) -> (w1497:string[][])  [unwired: 1 in]
                  n770 = Insert Into Array(array=w1497, index (col)=3 ("disabled index (col)"), new element=w1478) -> (w1498:string[][])  [unwired: 1 in]
                  n771 = Insert Into Array(array=w1498, index (col)=4 ("disabled index (col)"), new element=w1477) -> (w1499:string[][])  [unwired: 1 in]
                  n772 = Insert Into Array(array=w1499, index (row)=0, new element=string[] ["time", "Centroid X", "Centroid Y", "Motor Axis 1", "Motor Axis 2"] ("new element/subarray 2")) -> (w1481:string[][])  [unwired: 1 in]
                  n773 = call-poly <vilib>:"Write To Spreadsheet File.vi"("2D data"=w1481, "file path (dialog if empty)"=w1468) -> ()  [unwired: 6 in, 1 out]
                }
                frame True {
                }
              }
            }
            n774 = call <vilib>:"Add State(s) to Queue__jki_lib_state_machine.vi"("State(s) in (\"\")"=w1464) -> ("States Out"=w1463:string)  [unwired: 14 in]
            n775 = property on="Save Stats" class="Bool (strict)"("Value"=FALSE ("Save Stats")) -> ()  [unwired: 2 in, 2 out]
          }
          frame "tdms" {
            w1517 = 21600.0 ("new tdms")
            # "Your code here.\n(You can make a copy of, or modify, this frame)"
            n776 = Unbundle By Name(w1536) -> ("Data Value Reference out"=w1533:refnum<k34>, "Offset X"=w1535:dbl[][], "Offset Y"=w1530:dbl[][], "active axis refs 2"=w1532:T12)
            n777 = for {
              tunnel: w1535 -> [w1581]
              tunnel: w1530 -> [w1580]
              tunnel: w1534 -> [w1544] mode=indexing
              tunnel: w1533 -> [w1545]
              tunnel: w1532 -> [w1566]
              tunnel: w1531 -> [w1550]
              tunnel: [w1548] -> w1529
              i -> [w1567]
              n778 = Index Array(array=w1581, index (row)=w1567) -> (element=w1579:dbl[])  [unwired: 1 in]
              n779 = Index Array(array=w1580, index (row)=w1567) -> (element=w1578:dbl[])  [unwired: 1 in]
              n780 = Index Array(array=w1566, index=w1567) -> (element=w1565:cluster{"Ref X":refnum<vi>, "Ref Y":refnum<vi>})
              n781 = Reverse 1D Array(array=w1578) -> (reversed array=w1576:dbl[])
              n782 = Reverse 1D Array(array=w1579) -> (reversed array=w1577:dbl[])
              n783 = Unbundle By Name(w1565) -> ("Ref X"=w1564:refnum<vi>, "Ref Y"=w1563:refnum<vi>)
              n784 = Index Array(array=w1577) -> (element=w1575:dbl)  [unwired: 1 in]
              n785 = Index Array(array=w1576) -> (element=w1574:dbl)  [unwired: 1 in]
              n786 = property class="DigNum (strict)"(reference=w1564, error in=w1550) -> (error out=w1549:errorcluster, "Value"=w1558:dbl)  [unwired: 1 out]
              n787 = Build Array(w1575) -> (w1547:dbl[])
              n788 = Build Array(w1574) -> (w1569:dbl[])
              n789 = Get Date/Time In Seconds() -> (seconds since 1Jan1904=w1546:timestamp)
              n790 = Build Array(w1546) -> (w1542:timestamp[])
              n791 = property class="DigNum (strict)"(reference=w1563, error in=w1549) -> (error out=w1540:errorcluster, "Value"=w1552:dbl)  [unwired: 1 out]
              n792 = Build Array(w1558) -> (w1557:dbl[])
              n793 = TDMS Write(0:w1545, 5:w1544, 7:"time", 9:w1542, 11:w1540) -> (4:w1541:refnum<k34>, 15:w1539:errorcluster)  [unwired: 1 in, 2 out]
              n794 = Build Array(w1552) -> (w1551:dbl[])
              n795 = TDMS Write(0:w1541, 5:w1544, 7:"centroid X", 9:w1547, 11:w1539) -> (4:w1572:refnum<k34>, 6:w1571:string, 15:w1570:errorcluster)  [unwired: 1 in, 1 out]
              n796 = TDMS Write(0:w1572, 5:w1571, 7:"centroid Y", 9:w1569, 11:w1570) -> (4:w1561:refnum<k34>, 6:w1560:string, 15:w1562:errorcluster)  [unwired: 1 in, 1 out]
              n797 = TDMS Write(0:w1561, 5:w1560, 7:"Motor Axis 1", 9:w1557, 11:w1562) -> (4:w1556:refnum<k34>, 6:w1555:string, 15:w1553:errorcluster)  [unwired: 1 in, 1 out]
              n798 = TDMS Write(0:w1556, 5:w1555, 7:"Motor Axis 2", 9:w1551, 11:w1553) -> (15:w1548:errorcluster)  [unwired: 1 in, 3 out]
            }
            n799 = property on="millisecond timer value" class="DigNum (strict)"() -> ("Value"=w1523:u32)  [unwired: 2 in, 2 out]
            n800 = local read "millisecond timer 2"() -> (w1525:u32)
            n801 = Tick Count (ms)() -> (millisecond timer value=w1524:u32)
            n802 = call <userlib>:"Tick Count (ms)__ogtk.vi"("error in (no error)"=w1529) -> ("error out"=w1526:errorcluster, "millisecond timer value"=w1528:u32)  [unwired: 9 in]
            n803 = Subtract(x=w1524, y=w1523) -> (x-y=w1522:u32)
            n804 = Subtract(x=w1528, y=w1525) -> (x-y=→"Waveform Chart":u32)
            n805 = Divide(x=w1522, y=u32 1000) -> (x/y=w1520:dbl)
            n806 = Quotient & Remainder(x=w1520, y=w1517) -> (x-y*floor(x/y)=w1519:dbl)  [unwired: 1 out]
            n807 = Subtract(x=w1517, y=20.0) -> (x-y=w1515:dbl)
            n808 = Greater?(x=w1519, y=w1515) -> (0:w1518:bool)
            n809 = Select(t="newtdms", s=w1518, f="") -> (s? t:f=w1512:string)
            n810 = call <vilib>:"Add State(s) to Queue__jki_lib_state_machine.vi"("State(s) in (\"\")"=w1538, "State(s) at Back (\"\")"=w1512) -> ("States Out"=w1537:string)  [unwired: 13 in]
          }
          frame "Reset History" {
            # "Your code here.\n(You can make a copy of, or modify, this frame)"
            n811 = for {
              N: 1 -> [_]
              shift-right: [w1591] -> w1583
              shift-left: timestamp[][] [] ("Time") -> [w1593]
              n812 = for {
                N: 12 -> [_]
                tunnel: w1593 -> [w1596] mode=indexing
                tunnel: [w1594] -> w1591 mode=indexing
                n813 = Get Date/Time In Seconds() -> (seconds since 1Jan1904=w1595:timestamp)
                n814 = Build Array (concatenate)(w1596, w1595) -> (w1594:timestamp[])
              }
            }
            n815 = local read "Offset X"() -> (w1582:dbl[][])
            n816 = Bundle By Name(cluster=w1587, "Offset X"=w1582, "Offset Y"=w1582, "Time"=w1583, "Motor X"=w1582) -> (w1586:T36)
            n817 = call <vilib>:"Add State(s) to Queue__jki_lib_state_machine.vi"("State(s) in (\"\")"=w1590) -> ("States Out"=w1589:string)  [unwired: 14 in]
          }
          frame "New Category: 2" {
            # "Your code here.\n(You can make a copy of, or modify, this frame)"
            n818 = call <vilib>:"Add State(s) to Queue__jki_lib_state_machine.vi"("State(s) in (\"\")"=w1600) -> ("States Out"=w1599:string)  [unwired: 14 in]
          }
          frame "newtdms" {
            # "Your code here.\n(You can make a copy of, or modify, this frame)"
            n819 = Unbundle By Name(w1609) -> ("Data Value Reference out"=w1608:refnum<k34>)
            n820 = TDMS Close(8:w1607, 11:w1608) -> (0:w1606:errorcluster)  [unwired: 1 out]
            n821 = Get Date/Time In Seconds() -> (seconds since 1Jan1904=w1620:timestamp)
            n822 = Format Date/Time String(time format string (%c)="%Y%m%d%H%M", seconds (now)=w1620) -> (date/time string=w1611:string)  [unwired: 1 in]
            n823 = Concatenate Strings(w1611, "Beampointing_Pico.tdms" ("string")) -> (w1617:string)
            n824 = String To Path(string=w1617) -> (path=w1618:path)
            n825 = Build Path(base path=path "w:/BP_upstairs", name or relative path=w1618) -> (appended path=w1612:path)
            n826 = TDMS Open(6:FALSE ("disable buffering (T)"), 7:enum16{"1.0", "2.0"}."2.0" ("file format version (2.0)"), 8:w1606, 10:T17."create or replace" ("operation"), 11:w1612) -> (0:w1602:errorcluster, 3:w1605:refnum<k34>)  [unwired: 1 in]
            n827 = call "TDMSbuffersize.vi"("error in (no error)"=w1602, "group names"=w1604, "Data Value Reference in"=w1605) -> ("error out"=w1601:errorcluster, "Data Value Reference out"=w1603:refnum<k34>)  [unwired: 7 in]
            n828 = call <vilib>:"Add State(s) to Queue__jki_lib_state_machine.vi"("State(s) in (\"\")"=w1623) -> ("States Out"=w1622:string)  [unwired: 14 in]
            n829 = Bundle By Name(cluster=w1609, "Data Value Reference out"=w1603) -> (w1610:T36)
          }
          frame "Center" {
            # "Your code here.\n(You can make a copy of, or modify, this frame)"
            n830 = property on="Center" class="Bool (strict)"("Value"=FALSE ("Center")) -> ()  [unwired: 2 in, 2 out]
            n831 = control-ref of="image::1"() -> (w1638:refnum<vi>)
            n832 = control-ref of="image::2"() -> (w1637:refnum<vi>)
            n833 = control-ref of="image::3"() -> (w1636:refnum<vi>)
            n834 = control-ref of="image::4"() -> (w1635:refnum<vi>)
            n835 = control-ref of="image::5"() -> (w1634:refnum<vi>)
            n836 = control-ref of="image::6"() -> (w1633:refnum<vi>)
            n837 = control-ref of="image::7"() -> (w1632:refnum<vi>)
            n838 = control-ref of="image::8"() -> (w1631:refnum<vi>)
            n839 = control-ref of="image::9"() -> (w1630:refnum<vi>)
            n840 = control-ref of="image::10"() -> (w1629:refnum<vi>)
            n841 = control-ref of="image::11"() -> (w1628:refnum<vi>)
            n842 = control-ref of="image::12"() -> (w1627:refnum<vi>)
            n843 = for {
              tunnel: w1624 -> [w1651] mode=indexing
              tunnel: [w1646] -> w1639 mode=indexing
              n844 = Unbundle By Name(w1651) -> ("Target.X::12"=w1650:refnum<vi>, "Target.Y::12"=w1649:refnum<vi>)
              n845 = property class="DigNum (strict)"(reference=w1650) -> ("Value"=w1648:dbl)  [unwired: 1 in, 2 out]
              n846 = property class="DigNum (strict)"(reference=w1649) -> ("Value"=w1647:dbl)  [unwired: 1 in, 2 out]
              n847 = Bundle("Value"=w1648, "Value"=w1647) -> (w1646:cluster{"Value":dbl, "Value":dbl})  [unwired: 1 in]
            }
            n848 = call <vilib>:"Add State(s) to Queue__jki_lib_state_machine.vi"("State(s) in (\"\")"=w1643) -> ("States Out"=w1642:string)  [unwired: 14 in]
            n849 = Build Array(w1638, w1637, w1636, w1635, w1634, w1633, w1632, w1631, w1630, w1629, w1628, w1627) -> (w1626:refnum<vi>[])
            n850 = for {
              tunnel: w1626 -> [w1645] mode=indexing
              tunnel: w1639 -> [w1644] mode=indexing
              n851 = property class="ImageControl"(reference=w1645, "Image Center Position"=w1644) -> ()  [unwired: 1 in, 2 out]
            }
          }
          frame "history" {
            # "Your code here.\n(You can make a copy of, or modify, this frame)"
            n852 = Unbundle By Name(w1661) -> ("Offset X"=w1667:dbl[][], "Offset Y"=w1666:dbl[][], "Mean Centroid X"=w1665:dbl[][], "Mean Centroid Y"=w1664:dbl[][], "Motor X"=w1663:dbl[][], "Motor Y"=w1662:dbl[][], "Time"=w1653:timestamp[][])
            n853 = for {
              tunnel: w1667 -> [w1685] mode=indexing
              tunnel: w1666 -> [w1683] mode=indexing
              tunnel: w1665 -> [w1682] mode=indexing
              tunnel: w1664 -> [w1681] mode=indexing
              tunnel: w1663 -> [w1680] mode=indexing
              tunnel: w1662 -> [w1679] mode=indexing
              tunnel: [w1684] -> w1659 mode=indexing
              tunnel: [w1678] -> w1658 mode=indexing
              tunnel: [w1674] -> w1657 mode=indexing
              tunnel: [w1677] -> w1656 mode=indexing
              tunnel: [w1676] -> w1655 mode=indexing
              tunnel: [w1675] -> w1654 mode=indexing
              tunnel: w1653 -> [w1673] mode=indexing
              tunnel: [w1671] -> w1652 mode=indexing
              w1672 = 0
              n854 = Delete From Array(array=w1680, index=w1672) -> (array with subset deleted=w1676:dbl[])  [unwired: 1 in, 1 out]
              n855 = Delete From Array(array=w1679, index=w1672) -> (array with subset deleted=w1675:dbl[])  [unwired: 1 in, 1 out]
              n856 = Delete From Array(array=w1673, index=w1672) -> (array with subset deleted=w1671:timestamp[])  [unwired: 1 in, 1 out]
              n857 = Delete From Array(array=w1682, index=w1672) -> (array with subset deleted=w1674:dbl[])  [unwired: 1 in, 1 out]
              n858 = Delete From Array(array=w1681, index=w1672) -> (array with subset deleted=w1677:dbl[])  [unwired: 1 in, 1 out]
              n859 = Delete From Array(array=w1683, index=w1672) -> (array with subset deleted=w1678:dbl[])  [unwired: 1 in, 1 out]
              n860 = Delete From Array(array=w1685, index=w1672) -> (array with subset deleted=w1684:dbl[])  [unwired: 1 in, 1 out]
            }
            n861 = call <vilib>:"Add State(s) to Queue__jki_lib_state_machine.vi"("State(s) in (\"\")"=w1670) -> ("States Out"=w1669:string)  [unwired: 14 in]
            n862 = Bundle By Name(cluster=w1661, "Offset X"=w1659, "Offset Y"=w1658, "Mean Centroid X"=w1657, "Mean Centroid Y"=w1656, "Motor X"=w1655, "Motor Y"=w1654, "Time"=w1652) -> (w1660:T36)
          }
        }
        n863 = property on="Box" class="Arr (strict)"() -> ("Value"=w260:T6)  [unwired: 2 in, 2 out]
        n864 = for {
          tunnel: w262 -> [w286]
          tunnel: w261 -> [w287]
          tunnel: w253 -> [w279] mode=indexing
          tunnel: w260 -> [w280] mode=indexing
          n865 = call-poly <userlib>:"Filter 1D Array__ogtk.vi"("items to filter"=w279, "array"=w287) -> ("filtered item indices"=w288:i32[])  [unwired: 4 in, 1 out]
          n866 = Index Array(array=w288) -> (element=w282:i32)  [unwired: 1 in]
          n867 = Index Array(array=w286, index=w282) -> (element=w285:T30)
          n868 = Unbundle By Name(w285) -> ("Target.X::12"=w290:refnum<vi>, "Target.Y::12"=w289:refnum<vi>)
          n869 = property class="DigNum (strict)"(reference=w290) -> ("Value"=w284:dbl)  [unwired: 1 in, 2 out]
          n870 = property class="DigNum (strict)"(reference=w289) -> ("Value"=w283:dbl)  [unwired: 1 in, 2 out]
          n871 = call "draw crosshair imaq.vi"("Color"=u32 16774656, "Target.Y"=w283, "size"=cluster{"xhair size":dbl, "xhair size 2":dbl} {"xhair size"=25.0, "xhair size 2"=25.0}, "Target.X"=w284, "Bounding Rectangle"=T15 {"Left"=0, "Top"=0, "Right"=0, "Bottom"=0}, "image in"=w279) -> ("image out"=w278:T9)  [unwired: 4 in, 1 out]
          n872 = call "draw box imaq.vi"("Color"=u32 1244928, "Rectangle"=w280, "image in"=w278) -> ()  [unwired: 8 in, 1 out]
        }
        n873 = property on="ActiveMotor" class="Ring (strict)"() -> ("Strings []"=w255:string[])  [unwired: 2 in, 2 out]
        n874 = Index Array(array=w255, index="ActiveMotor") -> (element=w256:string)
        n875 = Not Equal?(x="ActiveMotorName::99", y=w256) -> (x != y?=w257:bool)
        n876 = case shown="True" w257 {
          tunnel: w255 -> [_ w276]
          tunnel: "ActiveMotorName::99" -> [_ w275]
          frame False {
          }
          frame True {
            n877 = Search 1D Array(1D array=w276, element=w275) -> (index of element=w274:i32)  [unwired: 1 in]
            n878 = property on="ActiveMotor" class="Ring (strict)"("Value"=w274) -> ()  [unwired: 2 in, 2 out]
          }
        }
      }
      n879 = control-ref of="This Application"() -> (w243:refnum<vi>)
      n880 = control-ref of="This VI"() -> (w247:refnum<vi>)
      n881 = Current VI's Menubar() -> (w246:refnum<k9>)
      n882 = call "GUI_Master_subvi_reentrant_queues.vi"("This Application"=w243, "error in (no error)"=w244, "tcp data event"=w242, "Caller menu reference"=w246, "Caller VI ref"=w247) -> ("error out"=→"error IO 2":errorcluster)  [unwired: 6 in]
      n883 = Unbundle By Name(w132) -> ("Data Value Reference out"=w131:refnum<k34>)
      n884 = for {
        tunnel: w161 -> [w251] mode=indexing
        tunnel: w160 -> [w250]
        tunnel: [w249] -> w130
        n885 = call "IMAQ Dispose"("Image"=w251, "error in (no error)"=w250) -> ("error out"=w249:errorcluster)  [unwired: 4 in]
      }
      n886 = TDMS Close(8:w130, 11:w131) -> (0:→"error out 2":errorcluster)  [unwired: 1 out]
    }
  }
